vi "Actor Core.vi"(8 "error in":errorcluster, 11 "ZenGage v3.0 UI in":refnum<class "ZenGage v3.0 UI.lvclass">) -> (0 "error out":errorcluster, 3 "Actor out":refnum<class "Actor.lvclass">)   [LabVIEW 2019, in "ZenGage v3.0 UI.lvclass"]
uses:
  ZenGage v3.0 UI.lvclass
  <vilib>/ActorFramework/Actor/Actor.lvclass
  <vilib>/ActorFramework/Message Enqueuer/Message Priority.ctl
  <vilib>/ActorFramework/Message Enqueuer/Message Enqueuer.lvclass
  <vilib>/event_ctls.llb/usereventprio.ctl
  Type Definitions/Controls and Indicators/General_Control references.ctl
  Type Definitions/Controls and Indicators/Inspection control references.ctl
  Type Definitions/Controls and Indicators/Diagnostics control referencs.ctl
  Type Definitions/Controls and Indicators/EDL control references.ctl
  Type Definitions/Controls and Indicators/Controls and Indicators Cluster.ctl
  Common/Controls/Acknowledgement.ctl
  Type Definitions/Controls and Indicators/String2.ctl
  <vilib>/vision/Image Controls.llb/IMAQ Image.ctl
  Type Definitions/Diagnostics/OpticsPOSTInputCluster.ctl
  <vilib>/Utility/miscctls.llb/LVPoint32TypeDef.ctl
  User Interface Messages/User Interface messages/Call function_UI Msg/ButtonPress_UI.lvclass
  Common/Controls/Pop-up Input.ctl
  User Interface Messages/User Interface messages/Display Popup Msg/DisplayPopup_UI.lvclass
  Type Definitions/General/OutputDetails.ctl
  Type Definitions/General/Output choice.ctl
  Type Definitions/JSON Read/UI JSON read cluster.ctl
  Type Definitions/General/JSONRead.ctl
  Type Definitions/Inspection/Inspection Cluster.ctl
  Type Definitions/Diagnostics/Diagnostics(Cluster).ctl
  Type Definitions/Edit tolerance settings/Rack Selection.ctl
  Type Definitions/Edit tolerance settings/Edit Tolerance Input.ctl
  Type Definitions/Edit tolerance settings/Edit Tolerance Overall Cluster.ctl
  Type Definitions/General/UI States(UI button enable disable).ctl
  Type Definitions/General/UIDataCluster.ctl
  Type Definitions/General/Master sample references.ctl
  C:/Program Files/National Instruments/LabVIEW 2019/vi.lib/ActorFramework/Actor/Actor.lvclass
  User interface UX/LabVIEW components (Controls and Indiactors)/Tables and listboxes/Combo box conventional list.ctl
panel:
  out "Ignored count":u64
  in  "Main Tab":T1(tab)=enum."Blank"
  in  "Diagnostics Tab":T2(tab)
  out "TL":string
  out "SensorDiagnosticsImage":T3(plugin-control)
  out "BUZZER OFF":u32(colorbox)=14803425
  out "STOP":u32(colorbox)=14803425
  out "PAUSE":u32(colorbox)=14803425
  out "RUN":u32(colorbox)=14803425
  out "CAMERA STATUS\n       MESSAGE":string
  out "DUST INDICATOR":dbl format="%#.3f"
  out "Diagnostics Image_Diagnostics":T3(plugin-control)
  in  "Master sample tab":enum32{"Master sample", "Inspection"}(tab)
  out "Master sample message":string
  in  "Hide":bool
  out "Counts":T4 {"Production counts clustwer"."TOTAL" scale=0.0..100.0; "Production counts clustwer"."PASS" scale=0.0..100.0; "Production counts clustwer"."FAIL" scale=0.0..100.0; "Reel counts cluster"."TOTAL" scale=0.0..100.0; "Reel counts cluster"."PASS" scale=0.0..100.0; "Reel counts cluster"."FAIL" scale=0.0..100.0}
  in  "Image label 4":string(combo)
  in  "Image label 3":string(combo)
  in  "Image label 1":string(combo)
  out "Image 4":T3(plugin-control)
  out "Image 3":T3(plugin-control)
  in  "Image label 2":string(combo)
  out "Image 2":T3(plugin-control)
  out "Image 1":T3(plugin-control)
  in  "Tolerance Limits Listbox":i32(listbox)
  in  "Command Tab":T5(tab)=enum."Inspection"
  out "Production Fail Ignore Count":u64
  in  "Fail count reverse":bool
  in  "Select a part":T6="Select a part"
  in  "Door Poka \nYoke":bool
  in  "Factory reset":bool
  in  "Restore to defaults_Edit Tolerance":bool
  in  "Logout_EditTolerance":bool
  in  "Measurement\nEnable":bool
  in  "Update List":bool
  in  "Save":bool
  out "Reel Fail Ignore Count":u64
  in  "Select message":string
  in  "Settings_Inspection":bool
  in  "Analytics_Inspection":bool
  in  "Event reason switching tab":enum32{"EventReason", "InspectionButtons"}(tab)
  in  "Event  Reason  List":string(combo)
  out "Event reason blink":string="Select an event\n  reason below"
  in  "confirm_eventReason":bool
  in  "Run_Inspection":bool
  in  "Pause_Inspection":bool
  in  "Stop_Inspection":bool
  in  "confirm":bool
  in  "Total Count":u64
  in  "Reel Count":u64
  in  "Operator Name":string
  in  "Part Name":T6
  in  "reset":bool
  in  "ok":bool
  in  "change":bool
  out "VERIFIED":bool
  in  "Master sample part message":string
  in  "Repeat":bool
  in  "Next":bool
  in  "Select a sub diagnostics":T6="Select a part"
  in  "logout_Diagnostics":bool
  in  "Select a diagnostics":T6="Select a part"
  in  "JSONRead.ConfigurationCluster.UIParameters.ImageIndicatorLayouts":T7(array[cluster])=[{"NumberOfImageIndicators"=1.0, "ImageSpecificData"=[{"Width"=0.98, "Left"=0.0, "Top"=0.0, "ImagePercentage"={"Height"=0.95, "Widthcorrection"=-20, "Heightcorrection"=-44, "Leftcorrection"=0.0, "Topcorrection"=0.0}, "StringPercentage"={"Height"=0.05, "Widthcorrection"=-14, "Heightcorrection"=0.0, "Leftcorrection"=0.0, "Topcorrection"=5.0}}]}, {"NumberOfImageIndicators"=2.0, "ImageSpecificData"=[{"Width"=0.5, "Left"=0.0, "Top"=0.0, "ImagePercentage"={"Height"=0.95, "Widthcorrection"=-20, "Heightcorrection"=-47, "Leftcorrection"=0.0, "Topcorrection"=3.0}, "StringPercentage"={"Height"=0.05, "Widthcorrection"=-30, "Heightcorrection"=0.0, "Leftcorrection"=0.0, "Topcorrection"=7.0}}, {"Width"=0.5, "Left"=0.0, "Top"=0.0, "ImagePercentage"={"Height"=0.95, "Widthcorrection"=-20, "Heightcorrection"=-47, "Leftcorrection"=0.0, "Topcorrection"=3.0}, "StringPercentage"={"Height"=0.05, "Widthcorrection"=-30, "Heightcorrection"=0.0, "Leftcorrection"=0.0, "Topcorrection"=7.0}}]}, {"NumberOfImageIndicators"=3.0, "ImageSpecificData"=[{"Width"=0.5, "Left"=0.0, "Top"=0.0, "ImagePercentage"={"Height"=0.45, "Widthcorrection"=-30, "Heightcorrection"=-50, "Leftcorrection"=0.0, "Topcorrection"=5.0}, "StringPercentage"={"Height"=0.05, "Widthcorrection"=-30, "Heightcorrection"=0.0, "Leftcorrection"=0.0, "Topcorrection"=7.0}}, {"Width"=0.5, "Left"=0.0, "Top"=0.5, "ImagePercentage"={"Height"=0.45, "Widthcorrection"=-30, "Heightcorrection"=-50, "Leftcorrection"=0.0, "Topcorrection"=5.0}, "StringPercentage"={"Height"=0.05, "Widthcorrection"=-30, "Heightcorrection"=0.0, "Leftcorrection"=0.0, "Topcorrection"=5.0}}, {"Width"=0.5, "Left"=0.5, "Top"=0.0, "ImagePercentage"={"Height"=0.95, "Widthcorrection"=-30, "Heightcorrection"=-47, "Leftcorrection"=-3.0, "Topcorrection"=5.0}, "StringPercentage"={"Height"=0.05, "Widthcorrection"=-33, "Heightcorrection"=3.0, "Leftcorrection"=3.0, "Topcorrection"=5.0}}]}, {"NumberOfImageIndicators"=3.0, "ImageSpecificData"=[{"Width"=0.5, "Left"=0.0, "Top"=0.0, "ImagePercentage"={"Height"=0.45, "Widthcorrection"=-30, "Heightcorrection"=-50, "Leftcorrection"=0.0, "Topcorrection"=5.0}, "StringPercentage"={"Height"=0.05, "Widthcorrection"=-30, "Heightcorrection"=0.0, "Leftcorrection"=0.0, "Topcorrection"=7.0}}, {"Width"=0.5, "Left"=0.0, "Top"=0.5, "ImagePercentage"={"Height"=0.45, "Widthcorrection"=-30, "Heightcorrection"=-50, "Leftcorrection"=0.0, "Topcorrection"=5.0}, "StringPercentage"={"Height"=0.05, "Widthcorrection"=-30, "Heightcorrection"=0.0, "Leftcorrection"=0.0, "Topcorrection"=5.0}}, {"Width"=0.5, "Left"=0.5, "Top"=0.0, "ImagePercentage"={"Height"=0.95, "Widthcorrection"=-30, "Heightcorrection"=-47, "Leftcorrection"=-3.0, "Topcorrection"=5.0}, "StringPercentage"={"Height"=0.05, "Widthcorrection"=-33, "Heightcorrection"=3.0, "Leftcorrection"=3.0, "Topcorrection"=5.0}}, {"Width"=0.5, "Left"=0.5, "Top"=0.5, "ImagePercentage"={"Height"=0.45, "Widthcorrection"=-30, "Heightcorrection"=-50, "Leftcorrection"=0.0, "Topcorrection"=5.0}, "StringPercentage"={"Height"=0.05, "Widthcorrection"=-30, "Heightcorrection"=0.0, "Leftcorrection"=0.0, "Topcorrection"=5.0}}]}]
  in  "UpdateImagingViews":bool
  out "Program flow":string
  in  "Inspection Tab":T8(tab)=enum."Diagnostics"
  in  "Tab Control":enum32{"EventReason"}(tab)
  out "Cards array":T9(array[cluster]) {"Measurement value" format="%#.3g"}
  out "Pass-Fail Indicator String":string
  out "Status display":u32(colorbox)=14277081
  in  "Diagnostics Status\nString":string
  out "Current\nDiagnostics\nStatus":u32(colorbox)=11776947
  in  "ETS tab":enum32{"Display", "Blank"}(tab)=enum."Blank"
  in  "Cluster of limits":T10
  in  "Threshold limits":T11 {"Spec Limit Fail Window" max=100000; "Control Limit Fail Window" max=100; "Spec Limit Fail Allowable" max=100000; "Control Limit Fail Allowable" max=100}
  in  "Bias Correction":dbl
  in  "Linearity Correction":dbl
  in  "ETL count error message":string
  out "ETL help string":string
  in  "SoftwareExit":bool caption="SoftwareExit_Inspection"
  # "Please select a measurement checkbox to make the required changes for that particular measurement"
  # "%"
  # "PRODUCTION"
  # "REEL"
  # "MASTER SAMPLE       VALIDATION"
  # "mm"
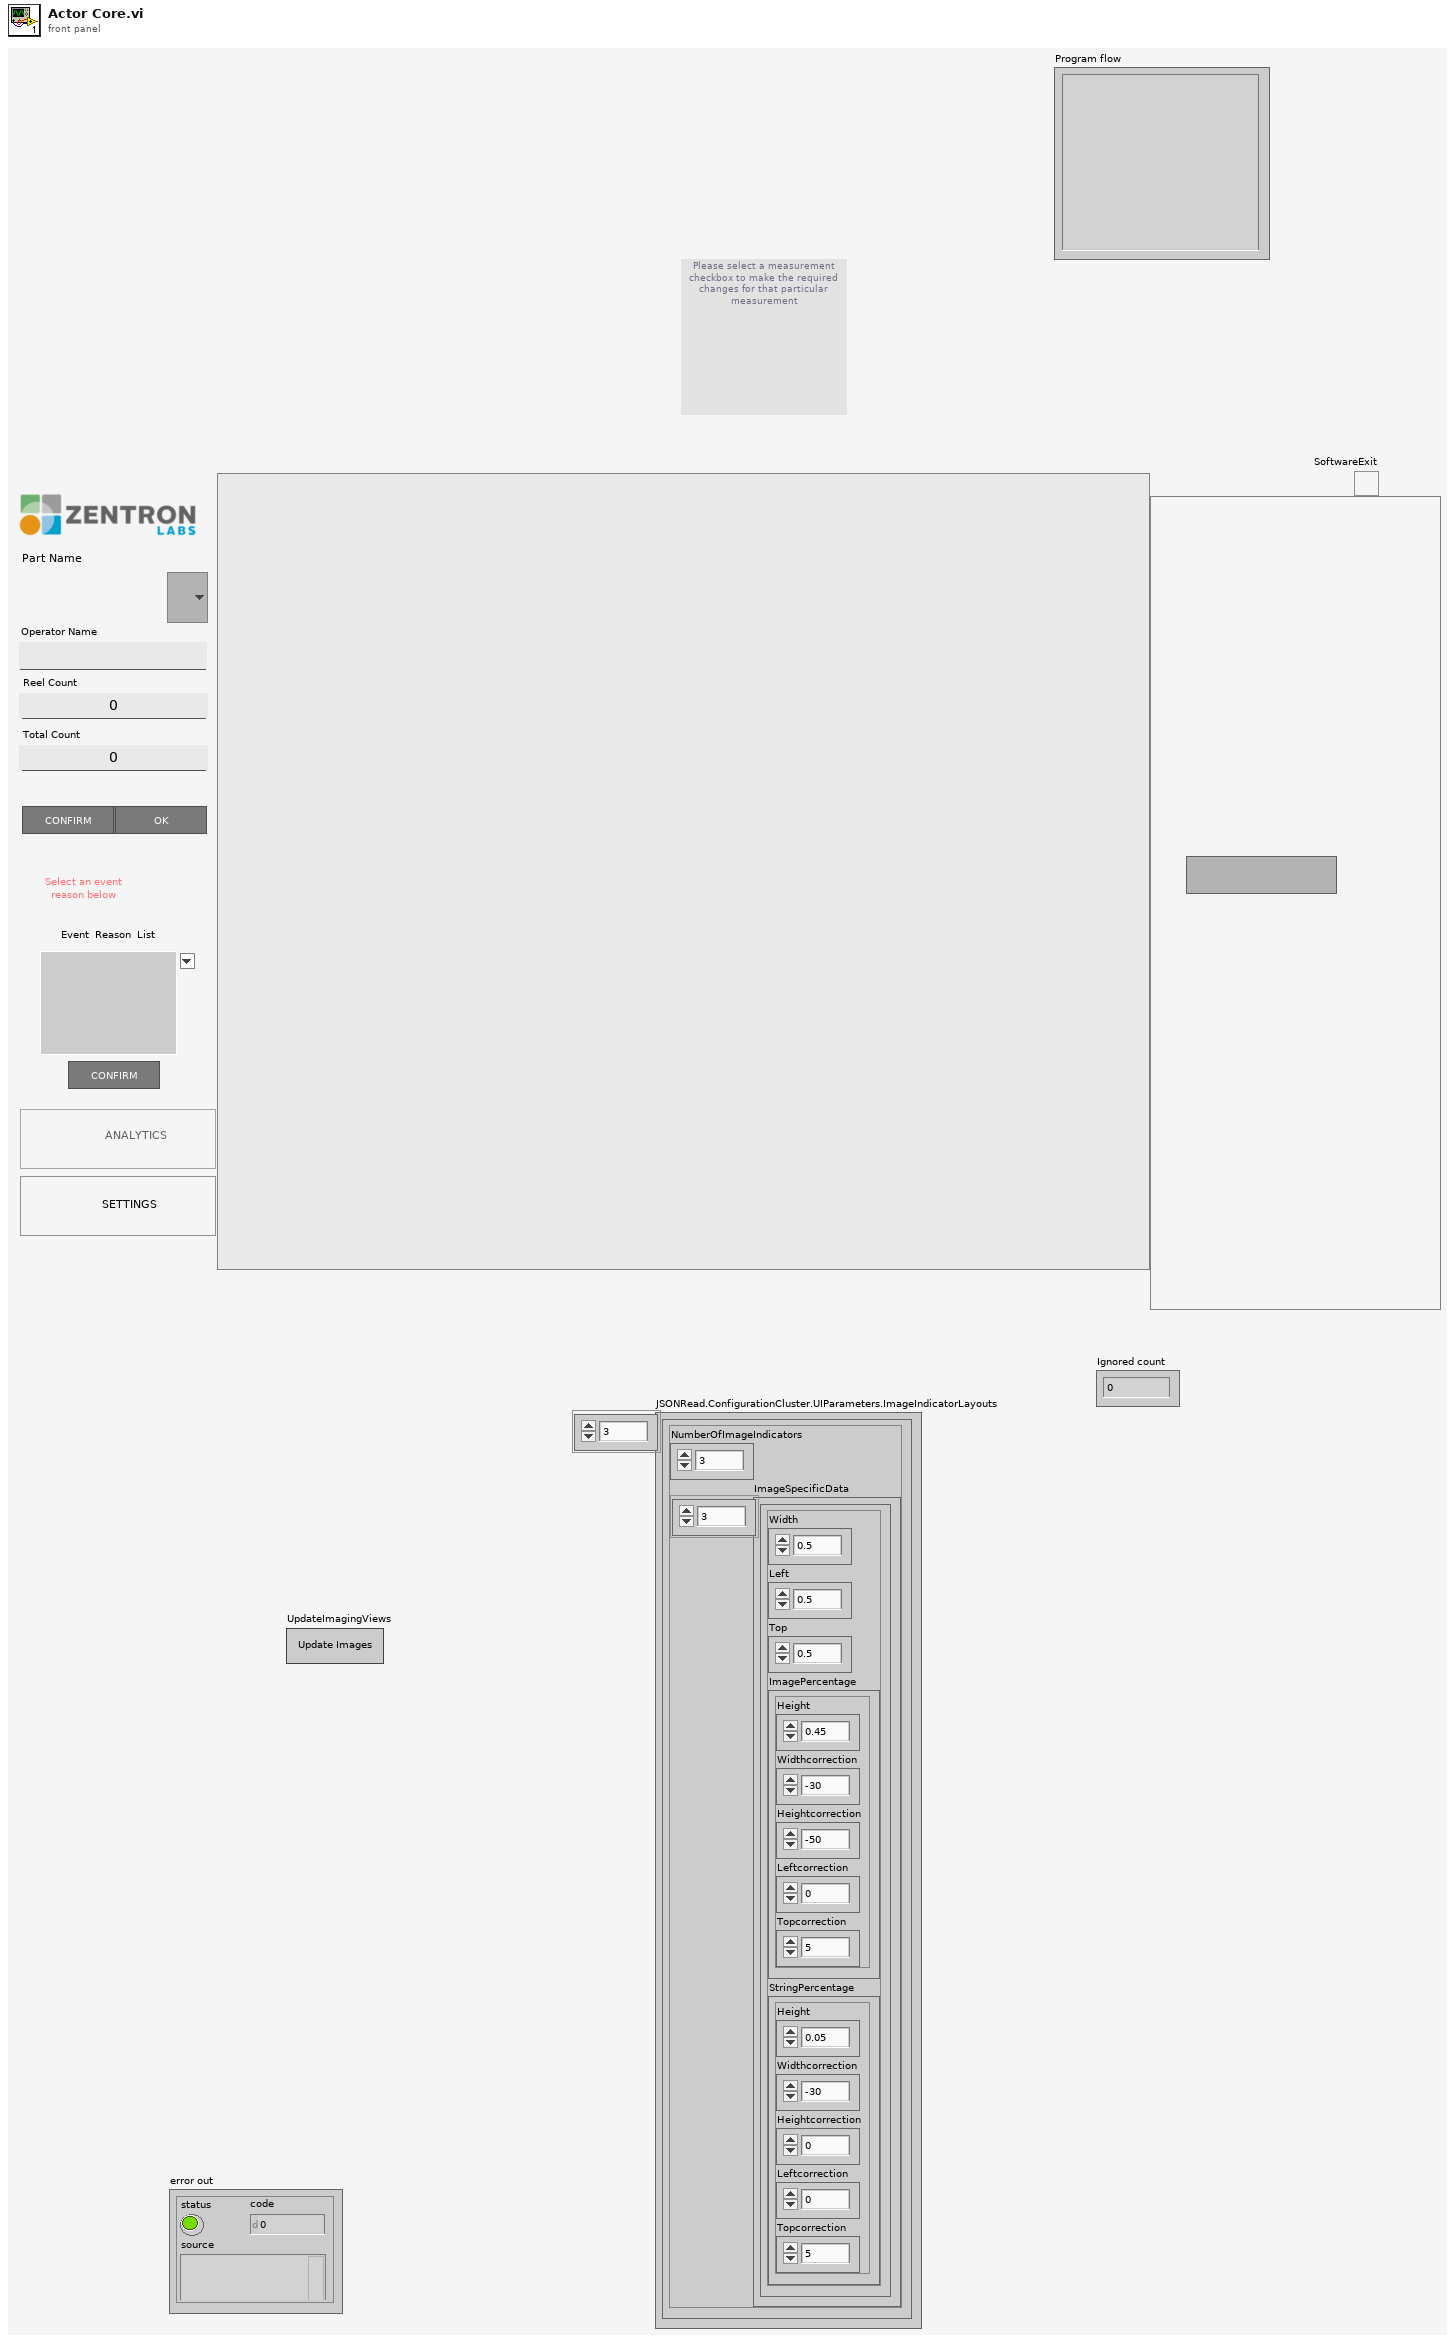
[diagram p1: front panel]
types:
  T1 = enum32{"Analytics", "Blank", "Diagnostics", "Run", "Edit Tolerance Settings"}
  T2 = enum32{"Arduino Motor", "Sensor trigger", "Hardware Button", "Camera Optics"}
  T3 = typedef "IMAQ Image.ctl" = refnum<image>
  T4 = cluster{"Reel counts cluster":cluster{"PASS":u64, "FAIL":u64, "TOTAL":u64}, "Production counts clustwer":cluster{"PASS":u64, "FAIL":u64, "TOTAL":u64}}
  T5 = enum32{"Edit Tolerance Limits1", "Inspection", "Master sample", "Diagnostics"}
  T6 = typedef "ZenGage v3.0 UI.lvclass/Combo box conventional list.ctl" = string
  T7 = cluster{"NumberOfImageIndicators":dbl, "ImageSpecificData":cluster{"Width":dbl, "Left":dbl, "Top":dbl, "ImagePercentage":cluster{"Height":dbl, "Widthcorrection":i64, "Heightcorrection":i64, "Leftcorrection":dbl, "Topcorrection":dbl}, "StringPercentage":cluster{"Height":dbl, "Widthcorrection":i64, "Heightcorrection":dbl, "Leftcorrection":dbl, "Topcorrection":dbl}}[]}[]
  T8 = enum32{"Inspection", "Diagnostics", "Edit Tolerance Settings"}
  T9 = cluster{"Measruement Name":string, "Measruement pass?":bool, "LSL":string, "USL 2":string, "Measurement value":dbl}[]
  T10 = cluster{"LSL":dbl, "USL":dbl, "LCL":dbl, "UCL":dbl}
  T11 = cluster{"Control Limit Fail Allowable":u64, "Spec Limit Fail Allowable":u64, "Control Limit Fail Window":u64, "Spec Limit Fail Window":u64}
  T12 = typedef "ZenGage v3.0 UI.lvclass/Controls and Indicators Cluster.ctl" = cluster{"General":T13, "Inspection":T14, "Diagnostics":T15, "Edit Tolerance Limits":T16, "Master sample":T17}
  T13 = typedef "ZenGage v3.0 UI.lvclass/General_Control references.ctl" = cluster{"Main Tab":refnum<vi>, "Inspection SubPanel_Inspection":refnum<vi>, "Zen Logo_Inspection":refnum<vi>, "SoftwareExit":refnum<vi>, "Loading Bar VI Ref":refnum<vi>, "Right Pane Tab":refnum<vi>, "Image Reference array":refnum<vi>[], "Command tab":refnum<vi>, "Inspection subTab control ref":refnum<vi>, "SelectionCluster":cluster{"ok":refnum<vi>, "confirm":refnum<vi>, "reset":refnum<vi>, "change":refnum<vi>, "TOTAL COUNT":refnum<vi>, "REEL COUNT":refnum<vi>, "PART NAME":refnum<vi>, "VERIFIED":refnum<vi>, "OPERATOR NAME":refnum<vi>, "Select message":refnum<vi>}, "Event  Reason  List":refnum<vi>, "Event reason blink":refnum<vi>, "Event reason switching tab":refnum<vi>, "confirm_eventReason":refnum<vi>}
  T14 = typedef "ZenGage v3.0 UI.lvclass/Inspection control references.ctl" = cluster{"Inspection Status":refnum<vi>, "Run_Inspection":refnum<vi>, "Pause_Inspection":refnum<vi>, "Stop_Inspection":refnum<vi>, "Settings_Inspection":refnum<vi>, "Inspection Images VI Ref":refnum<vi>, "Pass-Fail Indicator String":refnum<vi>, "Analytics_Inspection":refnum<vi>, "Label array":refnum<vi>[], "Analytics VI\nreference":refnum<vi>, "Counts":refnum<vi>, "Cards array":refnum<vi>, "Counts array":refnum<vi>[]}
  T15 = typedef "ZenGage v3.0 UI.lvclass/Diagnostics control referencs.ctl" = cluster{"Diagnostics Tab":refnum<vi>, "Dust indicator :":refnum<vi>, "Logout_Diagnostics":refnum<vi>, "CAMERA STATUS MESSAGE":refnum<vi>, "BUZZER OFF":refnum<vi>, "PAUSE":refnum<vi>, "STOP":refnum<vi>, "RUN":refnum<vi>, "Current Diagnostics Status":refnum<vi>, "Select a diagnostics":refnum<vi>, "Diagnostics Status":refnum<vi>, "Select a sub diagnostics":refnum<vi>, "Optics img":refnum<vi>, "Diagnostics Status\nString":refnum<vi>}
  T16 = typedef "ZenGage v3.0 UI.lvclass/EDL control references.ctl" = cluster{"Tolerance Limits Listbox":refnum<vi>, "Enable Disable":refnum<vi>, "Cluster of limits":refnum<vi>, "Thresholds limits":refnum<vi>, "Update List":refnum<vi>, "Save":refnum<vi>, "Back_Edit Tolerance":refnum<vi>, "logout":refnum<vi>, "Select a part":refnum<vi>, "Bias Correction":refnum<vi>, "Linearity Correction":refnum<vi>, "Select a Rack":refnum<vi>, "ETS tab":refnum<vi>, "Factory reset":refnum<vi>, "Door\nPoka Yoke":refnum<vi>, "Fail count reverse":refnum<vi>, "ETL count error message":refnum<vi>, "ETL help string":refnum<vi>}
  T17 = typedef "Master sample references.ctl" = cluster{"Master sample message":refnum<vi>, "Master sample tab":refnum<vi>, "Next":refnum<vi>, "Repeat":refnum<vi>, "Master sample part message":refnum<vi>}
  T18 = cluster{"ok":refnum<vi>, "confirm":refnum<vi>, "reset":refnum<vi>, "change":refnum<vi>, "TOTAL COUNT":refnum<vi>, "REEL COUNT":refnum<vi>, "PART NAME":refnum<vi>, "VERIFIED":refnum<vi>, "OPERATOR NAME":refnum<vi>, "Select message":refnum<vi>}
  T19 = typedef "ZenGage v3.0 UI.lvclass/OpticsPOSTInputCluster.ctl" = cluster{"Dust Percentage":dbl, "Diagnostics Sstatus string":string, "Pass?":bool, "final image":T3}
  T20 = typedef "ZenGage v3.0 UI.lvclass/String2.ctl" = string
  T21 = cluster{"MNA":string[], "ISIM":u8[], "Image update":cluster{"Rack Id":i32, "Update image":bool[]}[], "Current rack Id":u8, "LSL":string[], "USL":string[]}
  T22 = cluster{"Camera names":string[], "Rack Id 2":u8, "Measurement names":string[], "Number of racks":u8, "Tolerance limits":string[]}
  T23 = enum32{"invalid app kind", "Development System", "Run Time System", "Student Edition", "Embedded LabVIEW", "Evaluation", "Custom"}
  T24 = typedef "ZenGage v3.0 UI.lvclass/Output choice.ctl" = enum16{"SendIgnoredFailCount", "SendPartDetails", "ButtonPress", "SendAcknowledgement", "InitiateCameraDiagnostics", "InitiateSensorDiagnostics", "SendPopupResponse", "SendEventReasonResponse", "SendErrorDetails"}
  T25 = typedef "ZenGage v3.0 UI.lvclass/OutputDetails.ctl" = cluster{"Acknowledgement_SM":T26, "Button name":string, "PartDetails":cluster{"PartName":string, "ConnectorsInReel":u64, "TotalCounts":u64, "OperatorName":string, "StampingMachineID":u32}, "SensorName":string, "CameraName":string, "PopupFeedbackDetails":cluster{"Pop-up Type":enum16{"Open Logo Display", "Close Logo Display", "Open Loading Bar", "Close Loading Bar", "Open Alert Display", "Close Alert Display", "One button dialog box", "Two button dialog box", "User Authentication"}, "Message":string, "Pressed Button":string}, "EventResponse":string, "ErrorMessage":string, "FailCountIgnore":cluster{"ReelIgnoreCount":u64, "ProductionIgnoreCount":u64}}
  T26 = typedef "Acknowledgement.ctl" = cluster{"Enqueuer":refnum<class "Message Enqueuer.lvclass">, "VIReference":refnum<vi>, "VIName":string}
  T27 = enum32{"Invalid", "Standard", "Closed", "Hidden", "Minimized", "Maximized"}
  T28 = enum8{"Enabled", "Disabled", "Disabled and Grayed Out"}
  T29 = typedef "usereventprio.ctl" = enum32{"high priority", "normal priority"}
  T30 = cluster{"Image refnum":refnum<vi>, "Label refnum":refnum<vi>}
  T31 = cluster{"Part Name":refnum<vi>, "Verification":refnum<vi>, "Change":refnum<vi>, "Confirm":refnum<vi>, "OK Button":refnum<vi>, "Reset Button":refnum<vi>, "Total count":refnum<vi>, "Reel count":refnum<vi>, "Operator ID":refnum<vi>, "Select message":refnum<vi>, "Inspection Run":refnum<vi>}
  T32 = cluster{"Selection cluster":cluster{"ok":refnum<vi>, "confirm":refnum<vi>, "reset":refnum<vi>, "change":refnum<vi>, "TOTAL COUNT":refnum<vi>, "REEL COUNT":refnum<vi>, "PART NAME":refnum<vi>, "VERIFIED":refnum<vi>, "OPERATOR NAME":refnum<vi>, "Select message":refnum<vi>}, "Event  Reason  List":refnum<vi>}
  T33 = cluster{"Label array":refnum<vi>[], "Image ref array":refnum<vi>[], "Rack 1 Tbl Refnum":refnum<vi>, "Tab control":refnum<vi>, "Rack 2 Tbl Refnum":refnum<vi>, "String label":refnum<vi>[], "Diagnostics tab ref":refnum<vi>, "Counts":refnum<vi>}
  T34 = typedef "Actor Framework.lvlib/Message Enqueuer.lvclass/Message Priority.ctl" = enum16{"Low", "Normal", "High"}
  T35 = enum16{"Open Logo Display", "Close Logo Display", "Open Loading Bar", "Close Loading Bar", "Open Alert Display", "Close Alert Display", "One button dialog box", "Two button dialog box", "User Authentication"}
  T36 = cluster{"Stop slave user event_UI":refnum<user-event>, "Enable shortkey":refnum<user-event>, "SendClusterData":refnum<user-event>, "SendClusterData to MainLoop":refnum<user-event>}
  T37 = typedef "ZenGage v3.0 UI.lvclass/UserEvents_UI.ctl" = cluster{"LoadingBar_General_UI":refnum<user-event>, "OpticsDiagnostics_UI":refnum<user-event>, "DisplayResult_UI":refnum<user-event>, "DisplayPopup_UI":refnum<user-event>, "DisplayProcessCapabilityPopup_UI":refnum<user-event>, "ButtonPress_UI":refnum<user-event>, "GetAnalyticsVI_UI":refnum<user-event>, "SystemInfo_UI":refnum<user-event>, "PartInfo_UI":refnum<user-event>, "TriggerSensorDiagnostics_UI":refnum<user-event>, "AskEventReason_UI":refnum<user-event>, "Display CpCpk data_UI":refnum<user-event>, "MasterSampleMessageUpdate_UI":refnum<user-event>}
  T38 = typedef "UIDataCluster.ctl" = cluster{"JSONRead":T39, "Inspection":T41, "Diagnostics":T42, "EditToleranceSettings":T43, "ControlsIndicators":T12, "AdditionalFeatures":cluster{"Cp Cpk details":cluster{"CpCpkData":string[][], "Cp Cpk popup":refnum<vi>}, "Popup":cluster{"Restore main tab":string, "Popup data":cluster{"Loading bar data":cluster{"Open?":bool, "Display string":string}, "Pop-up":T47}}, "DynamicImageHandling":cluster{"Image update":cluster{"Rack Id":i32, "Update image":bool[]}[], "RBCIA":cluster{"Rack Id":u8, "Imaging view names":string[]}[], "ISIM":u8[], "Camera labels list":string[], "Enable DIH?":bool, "Init DIH params?":bool}, "PageHandling":cluster{"Previous State":T48, "Current state":string, "Previous control access state":string}, "Core":cluster{"Current VI Reference":refnum<vi>, "Close Panel on Exit?":bool}, "SlaveLoopData":cluster{"EnableShortKeyPress":bool, "Point32":T46}, "Chosen event reason":string, "Master sample validation":cluster{"Master sample general message":string, "Master sample part message":string}, "Fail Ignore Count Reversal":cluster{"Production ignored count":u64, "Reel ignored count":u64}}}
  T39 = typedef "ZenGage v3.0 UI.lvclass/JSONRead.ctl" = cluster{"ConfigurationFilePaths":cluster{"Default JSON Path in":path, "Rack Controller Override JSON file path in":path, "Algorithm Overrride JSON file path in ":path}, "ConfigurationVariants":cluster{"Default JSON \nVariant":variant, "Algorithm Override\nJSON Variant":variant, "Rack Controller Override\nJSON Variant":variant}, "ConfigurationCluster":T40}
  T40 = typedef "ZenGage v3.0 UI.lvclass/UI JSON read cluster.ctl" = cluster{"UIParameters":cluster{"SpecificationVersion":string, "Title":string, "NumberOfImagesToBeDisplayed":dbl, "ImageCountWindow":dbl, "FontName":string, "FontSize":dbl, "CustomerLogoFilePath":string, "ZentronLogoFilePath":string, "CompatibleSoftwareVersions":string[], "CameraLabelMapping":cluster{"CameraName":string, "ImageLabel":string}[], "ImageIndicatorLayouts":cluster{"NumberOfImageIndicators":dbl, "ImageSpecificData":cluster{"Width":dbl, "Left":dbl, "Top":dbl, "ImagePercentage":cluster{"Height":dbl, "Widthcorrection":i64, "Heightcorrection":i64, "Leftcorrection":dbl, "Topcorrection":dbl}, "StringPercentage":cluster{"Height":dbl, "Widthcorrection":i64, "Heightcorrection":dbl, "Leftcorrection":dbl, "Topcorrection":dbl}}[]}[], "SoftwareButtonLabels":cluster{"SelectLabel":string, "RunLabel":string, "PauseLabel":string, "StopLabel":string}, "DiagnosticsParameters":cluster{"CameraOpticsDiagnostics":cluster{"Label":string, "CameraLabelsList":cluster{"CameraName":string, "ImageLabel":string}[]}, "ArduinoDiagnostics":cluster{"Label":string}, "MotorDiagnostics":cluster{"Label":string}, "ReelerMotor":cluster{"Label":string}, "TowerLampDiagnostics":cluster{"Label":string}, "TriggerSensor":cluster{"Label":string, "SensorsList":cluster{"SensorName":string, "LabelName":string}[]}, "HardwareButtonDiagnostics":cluster{"Label":string}, "MasterSampleDiagnostics":cluster{"Label":string}}, "DieIdParameters":cluster{"DefaultDieId":string, "DieIdsList":string[]}, "EventReasonsList":cluster{"Pause":string[], "Stop":string[], "FailPause":string[], "Ignored":string[], "DefaultEventReason":string}, "StampingMachineIds":string[], "ErrorPopupStrings":cluster{"ErrorCode":string, "ErrorString":string}[]}}
  T41 = typedef "ZenGage v3.0 UI.lvclass/Inspection Cluster.ctl" = cluster{"Inspection After Stop":bool, "IsPaused":bool, "Camera Names":string[], "Fail Array":bool[], "Reel Number":u32, "Image details_init":cluster{"Mapped view names":string[], "Camera image map array":i32[], "Camera names":string[]}[], "LSL":string[], "USL":string[], "Max limits":cluster{"Production max":u64, "Reel max":u64}, "parts List":string[], "#Racks":u8, "MeasurementNames":string[], "Reel complete":bool, "Fail event reason list":string[]}
  T42 = typedef "ZenGage v3.0 UI.lvclass/Diagnostics(Cluster).ctl" = cluster{"Selection Done?":bool, "Diagnostics details":cluster{"Diagnostics names":cluster{"Main diagnostics":string[], "Sub diagnostics names":cluster{"Camera optics":string[], "Trigger sensor":string[]}}, "Diagnostics labels":cluster{"Main diagnostics":string[], "Sub diagnostics names":cluster{"Camera optics":string[], "Trigger sensor":string[]}}}, "DiagnosticsFeatures":cluster{"ArduinoDiagnostics":bool, "MotorDiagnostics":bool, "CameraOpticsDiagnostics":bool, "ReelerMotor":bool, "HardwareButtonDiagnostics":bool, "TriggerSensor":bool, "TowerLampDiagnostics":bool, "MasterSampleDiagnostics":bool}, "SelectedDiagnostics":string}
  T43 = typedef "ZenGage v3.0 UI.lvclass/Edit Tolerance Overall Cluster.ctl" = cluster{"Input ListBox":T44, "Saved?":bool, "IsETLSelected":bool, "IsPartSelected":bool}
  T44 = typedef "ZenGage v3.0 UI.lvclass/Edit Tolerance Input.ctl" = cluster{"Measurement Values":string[][], "Cluster of Limits":cluster{"LSL":dbl, "USL":dbl, "LCL":dbl, "UCL":dbl}, "Rack Selection":T45, "M and N Array":cluster{"M1":u64, "M2":u64, "N1":u64, "N2":u64}[], "Ticked Measurement Index":u32[], "Measurements Enabled":bool[], "Current Active Position":T46, "Current ticked measurement":dbl}
  T45 = typedef "ZenGage v3.0 UI.lvclass/Rack Selection.ctl" = enum16{"Both Racks", "Rack 2", "Rack 1"}
  T46 = typedef "LVPoint32TypeDef.ctl" = cluster{"Horizontal":i32, "Vertical":i32}
  T47 = typedef "Pop-up Input.ctl" = cluster{"Pop-up Type":enum16{"Open Logo Display", "Close Logo Display", "Open Loading Bar", "Close Loading Bar", "Open Alert Display", "Close Alert Display", "One button dialog box", "Two button dialog box", "User Authentication"}, "Title":string, "Message":string, "Button 1 Text":string, "Button 2 Text":string, "Show Close? T/F":bool, "Title Blink? T/F":bool, "Title Blink Colour":u32}
  T48 = typedef "ZenGage v3.0 UI.lvclass/UI States(UI button enable disable).ctl" = cluster{"Inspection":cluster{"Inspection States":enum16{"PreSelect", "Back _Inspection", "Analytics", "Ready To Run", "Ready To Insert", "Enable All buttons", "Disable All Buttons", "Settings", "Select", "Stop", "Pause", "Inspect"}}, "Diagnostics":cluster{"Diagnostics States":enum16{"Enable All", "Camera Optics Fail", "Loading Bar", "Camera Optics", "Motor", "Arduino", "POST Done", "POST"}}, "Edit Tolerance":cluster{"Edit Limits":enum16{"Update List"}, "Enable Disable Measurements":enum16{"Back to Edit Tolerance"}, "Page Select":enum16{"Edit Tolerance Limits", "Enable Disable Buttons"}}, "Page Select":enum16{"Edit Tolerance", "Diagnostics", "Inspection"}}
  T49 = cluster{"Total Count":dbl, "Total Pass":dbl, "Total Fail":dbl}
  T50 = typedef "ZenGage v3.0 UI.lvclass/Result Cluster.ctl" = cluster{"Rack Id":u64, "Measurement Values Array ":dbl[], "Images_Array_in":T3[], "ResultPF":bool, "Production count details":cluster{"Total Count":dbl, "Total Pass":dbl, "Total Fail":dbl}, "Control Pass Fail":bool[], "ReelCount Details":cluster{"Reel Count":dbl, "Reel Pass":dbl, "Reel Fail":dbl}, "Specification Pass Fail":bool[], "SpecificationFail":bool}
  T51 = cluster{"Top Left":T3, "Bottom Left":T3, "Top Right":T3, "Inspection Status 2":u32, "Pass-Fail Indicator String 2":string, "Bottom right":T3, "Valid image data?":bool[], "Valid table data?":bool[], "Cards":cluster{"Measurement Name":string, "Pass?":bool, "LSL":string, "USL":string, "Measruement Value":dbl}[], "Counts":cluster{"Reel":cluster{"Pass":u64, "Fail":u64, "Total":u64}, "Production":cluster{"Pass":u64, "Fail":u64, "Total":u64}}}
  T52 = cluster{"Reel":cluster{"Pass":u64, "Fail":u64, "Total":u64}, "Production":cluster{"Pass":u64, "Fail":u64, "Total":u64}}
  T53 = cluster{"Measurement Name":string, "Pass?":bool, "LSL":string, "USL":string, "Measruement Value":dbl}[]
  T54 = cluster{"ArduinoDiagnostics":bool, "MotorDiagnostics":bool, "CameraOpticsDiagnostics":bool, "ReelerMotor":bool, "TowerLampDiagnostics":bool, "HardwareButtonDiagnostics":bool, "TriggerSensor":bool, "MasterSampleDiagnostics":bool}
  T55 = cluster{"Part name":string, "NumberOfRacks":u8}[]
  T56 = cluster{"LCL":dbl, "UCL":dbl, "LSL":dbl, "USL":dbl, "NominalValue":dbl}[]
  T57 = cluster{"Mapped view names":string[], "Camera image map array":i32[], "Camera names":string[]}[]
  T58 = cluster{"Cp Cpk details":cluster{"CpCpkData":string[][], "Cp Cpk popup":refnum<vi>}, "Popup":cluster{"Restore main tab":string, "Popup data":cluster{"Loading bar data":cluster{"Open?":bool, "Display string":string}, "Pop-up":T47}}, "DynamicImageHandling":cluster{"Image update":cluster{"Rack Id":i32, "Update image":bool[]}[], "RBCIA":cluster{"Rack Id":u8, "Imaging view names":string[]}[], "ISIM":u8[], "Camera labels list":string[], "Enable DIH?":bool, "Init DIH params?":bool}, "PageHandling":cluster{"Previous State":T48, "Current state":string, "Previous control access state":string}, "Core":cluster{"Current VI Reference":refnum<vi>, "Close Panel on Exit?":bool}, "SlaveLoopData":cluster{"EnableShortKeyPress":bool, "Point32":T46}, "Chosen event reason":string, "Master sample validation":cluster{"Master sample general message":string, "Master sample part message":string}, "Fail Ignore Count Reversal":cluster{"Production ignored count":u64, "Reel ignored count":u64}}
  T59 = cluster{"Image update":cluster{"Rack Id":i32, "Update image":bool[]}[], "RBCIA":cluster{"Rack Id":u8, "Imaging view names":string[]}[], "ISIM":u8[], "Camera labels list":string[], "Enable DIH?":bool, "Init DIH params?":bool}
  T60 = cluster{"Image update":cluster{"Rack Id":i32, "Update image":bool[]}[], "RBCIA":cluster{"Rack Id":u8, "Imaging view names":string[]}[], "ISIM":u8[], "Camera labels list":string[], "Enable DIH?":bool, "Init params":bool}
  T61 = cluster{"Default JSON Path in":path, "Rack Controller Override JSON file path in":path, "Algorithm Overrride JSON file path in ":path}
  T62 = cluster{"Current VI Reference":refnum<vi>, "Close Panel on Exit?":bool}
  T63 = typedef "ZenGage v3.0 UI.lvclass/Pop-up Output.ctl" = cluster{"Pop-up Type":enum16{"Open Logo Display", "Close Logo Display", "Open Loading Bar", "Close Loading Bar", "Open Alert Display", "Close Alert Display", "One button dialog box", "Two button dialog box", "User Authentication"}, "Message":string, "Pressed Button":string}
  T64 = cluster{"PartName":string, "ConnectorsInReel":u64, "TotalCounts":u64, "OperatorName":string, "StampingMachineID":u32}
  T65 = cluster{"CameraName":string, "ImageLabel":string}[]
  T66 = enum16{"cancel", "edit tolerance", "diagnostics"}
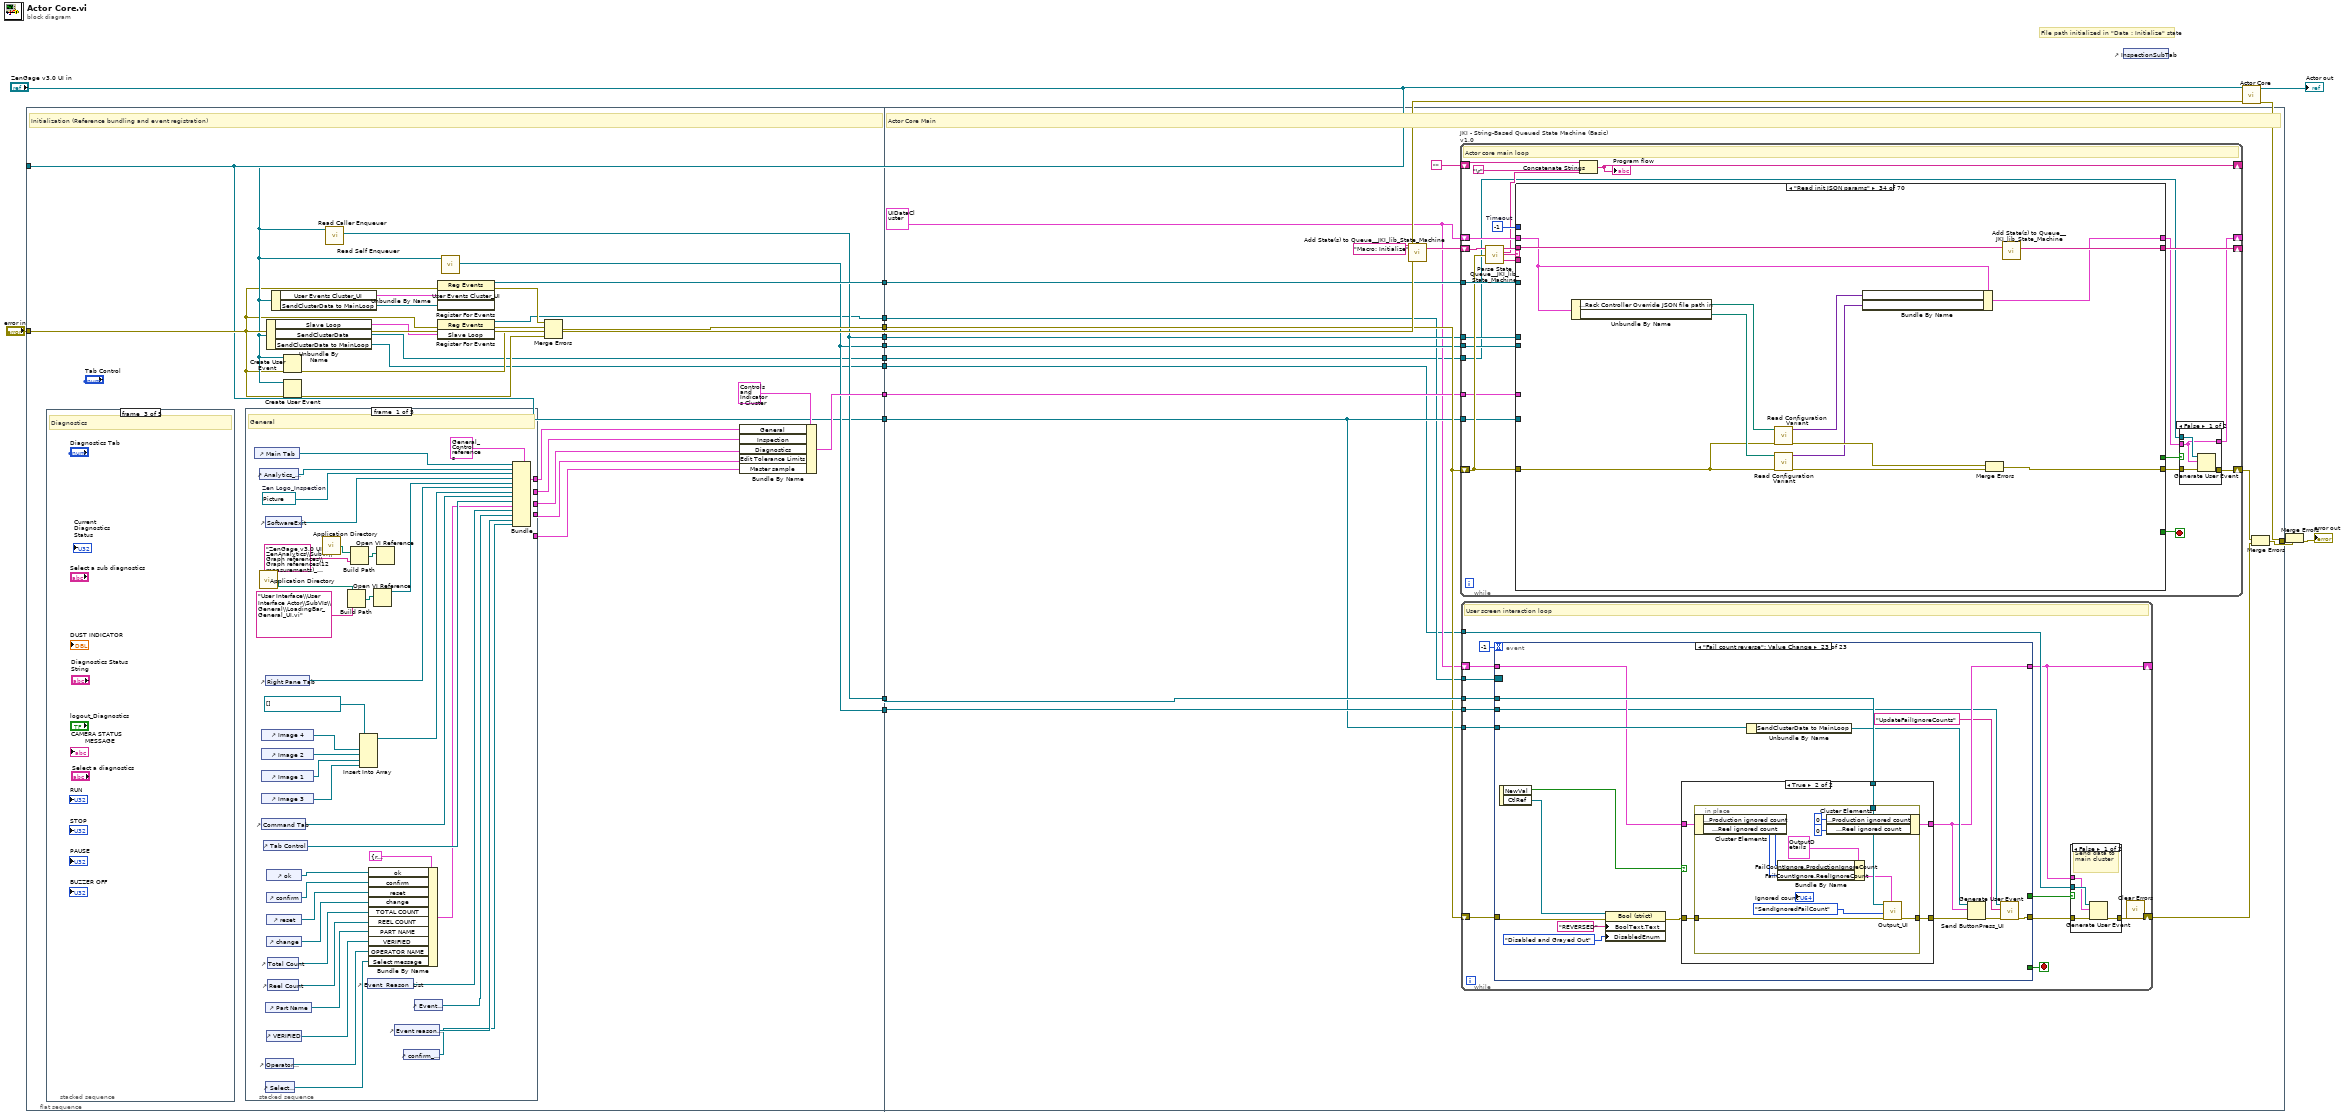
[diagram p0: block diagram]
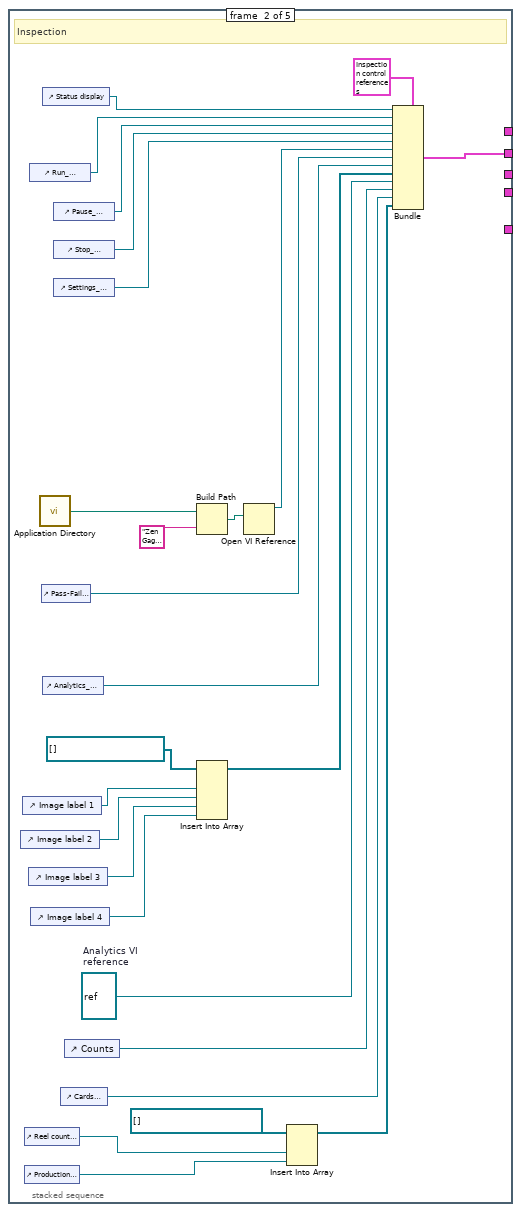
[diagram p2: hidden frame]
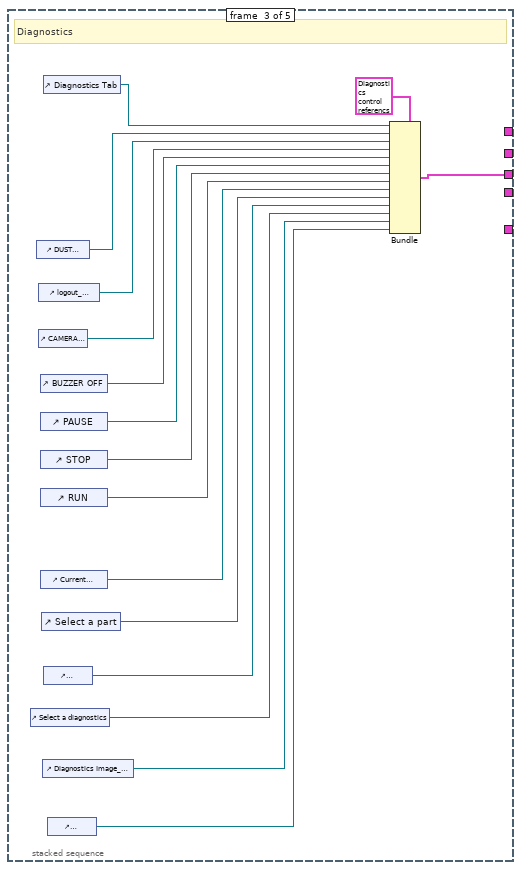
[diagram p3: hidden frame]
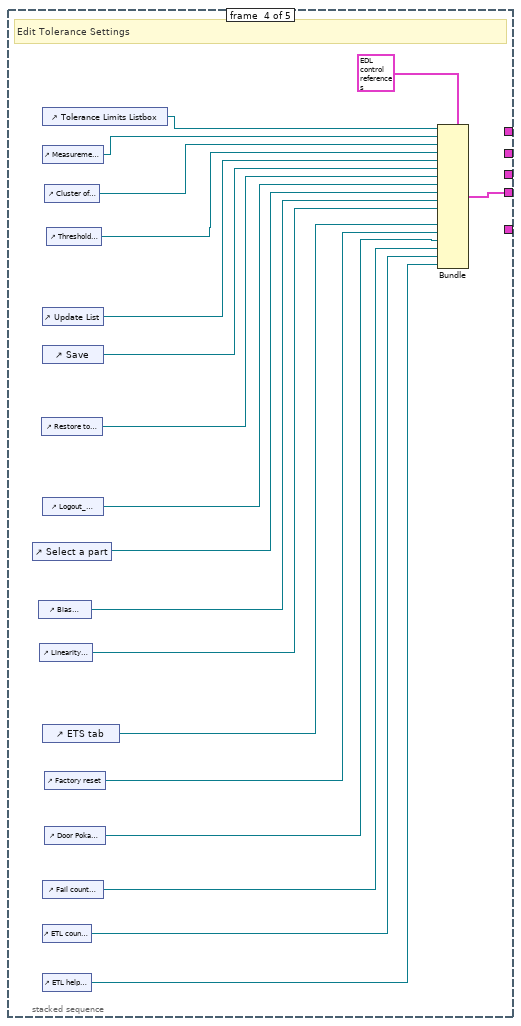
[diagram p4: hidden frame]
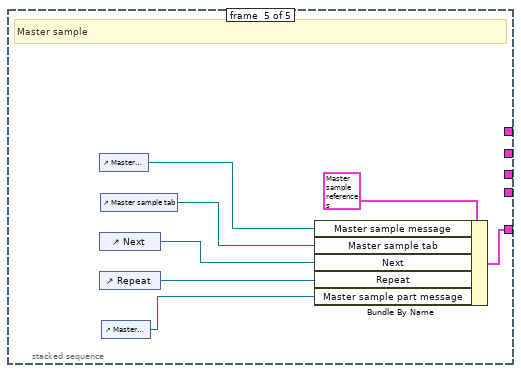
[diagram p5: hidden frame]
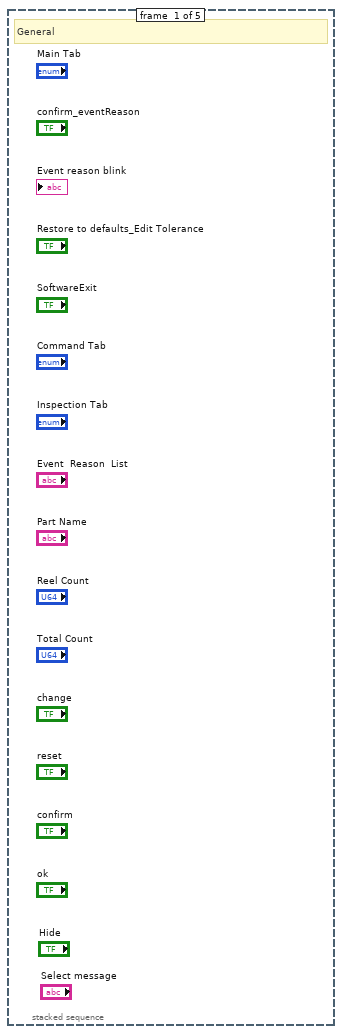
[diagram p6: hidden frame]
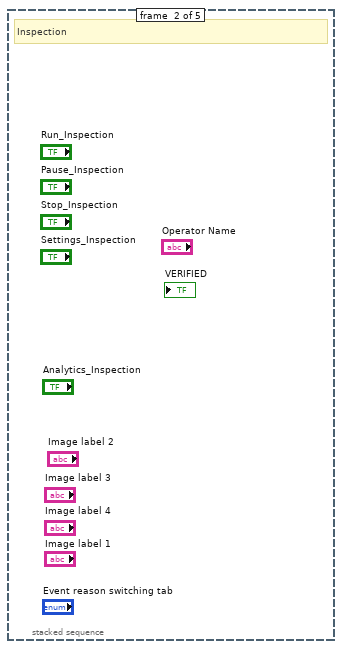
[diagram p7: hidden frame]
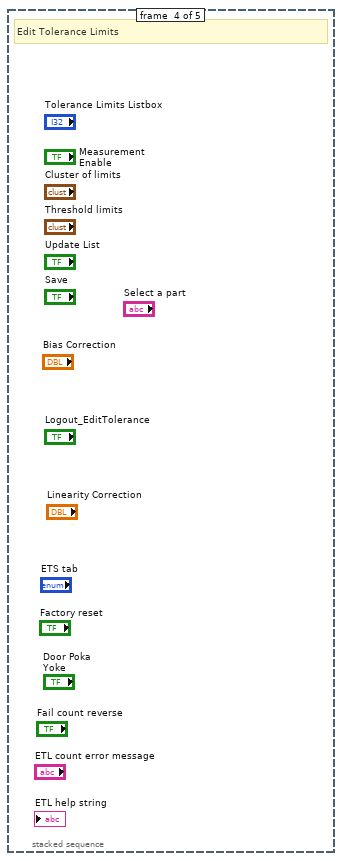
[diagram p8: hidden frame]
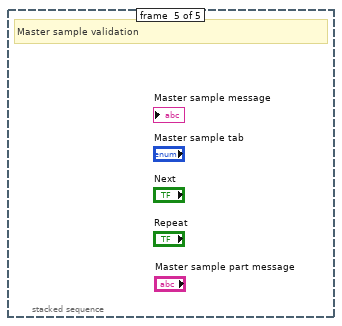
[diagram p9: hidden frame]
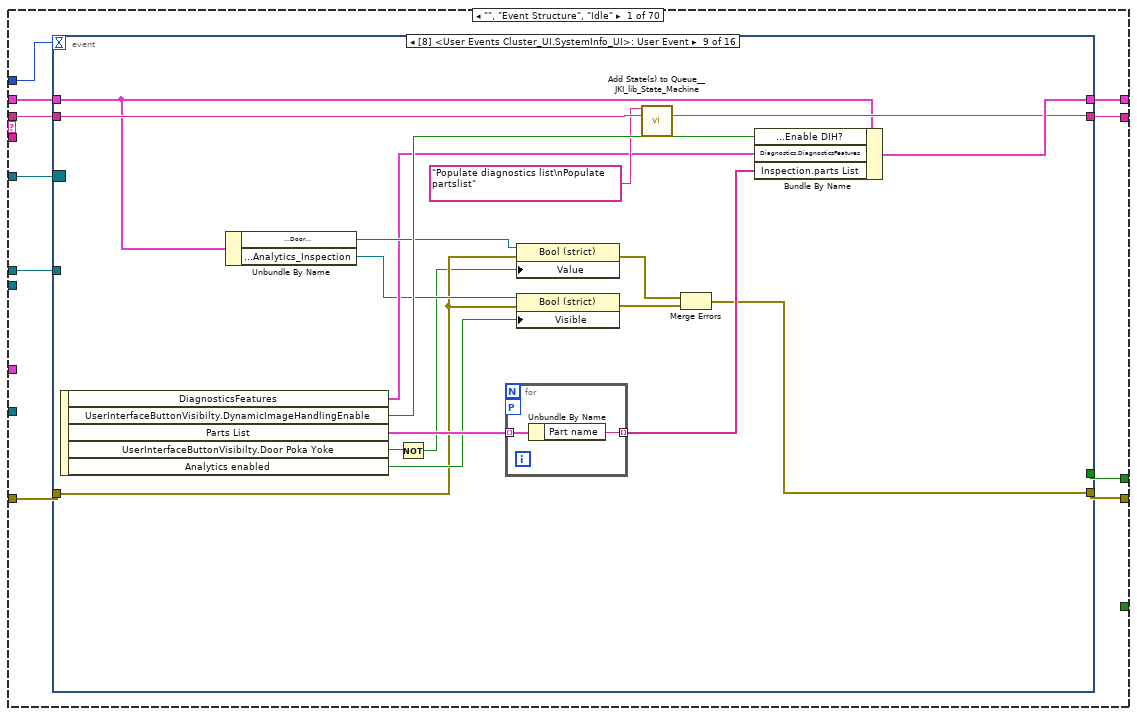
[diagram p11: hidden frame]
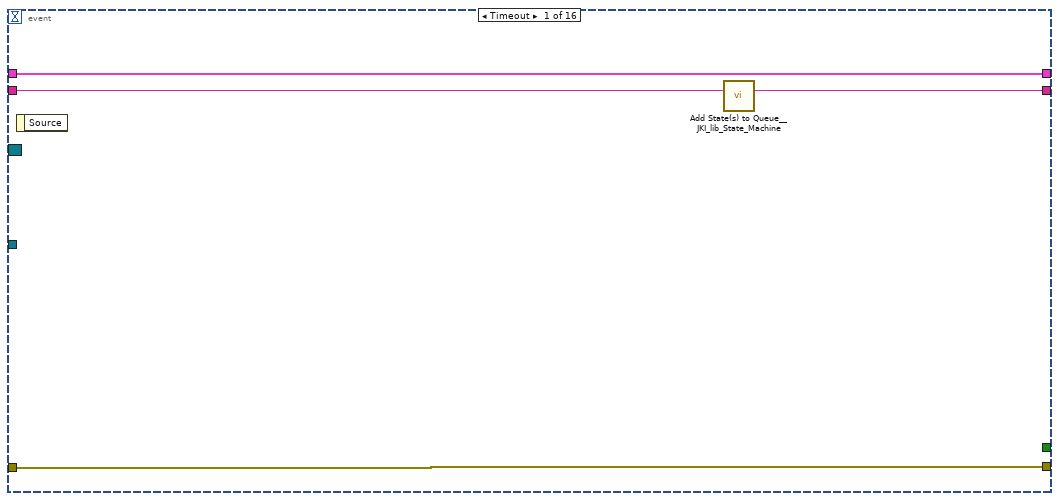
[diagram p12: hidden frame]
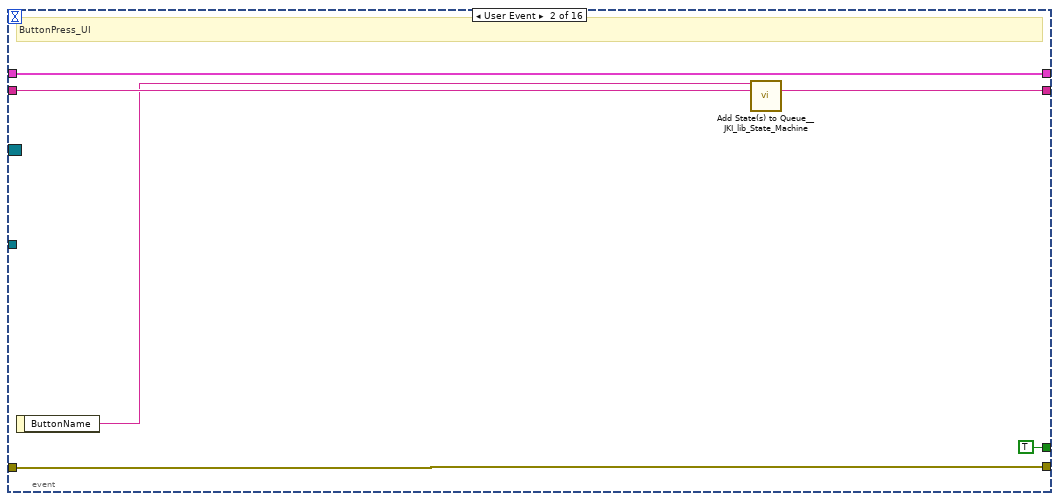
[diagram p13: hidden frame]
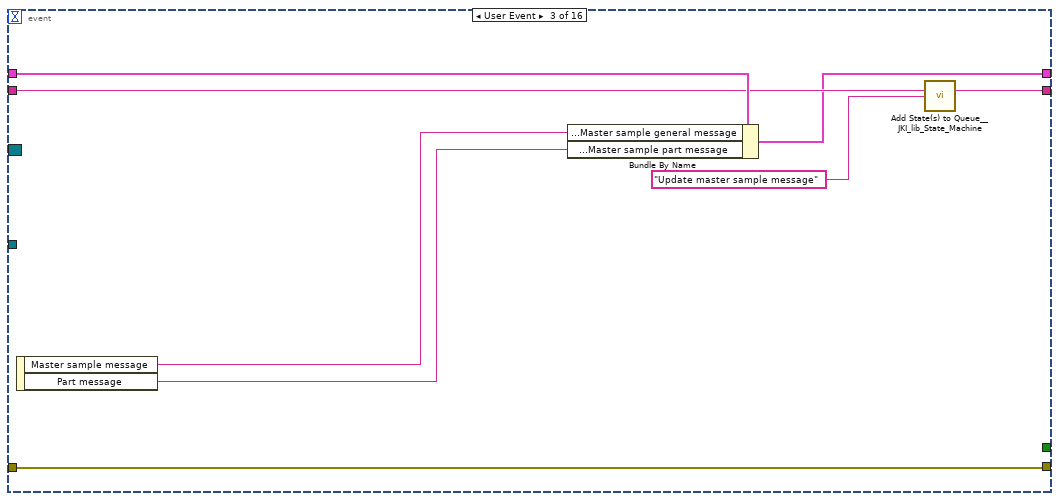
[diagram p14: hidden frame]
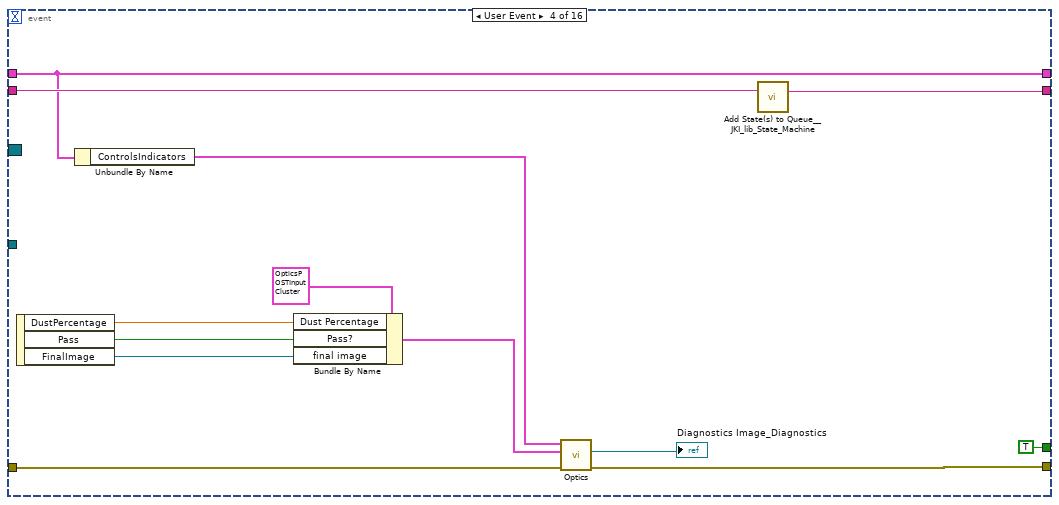
[diagram p15: hidden frame]
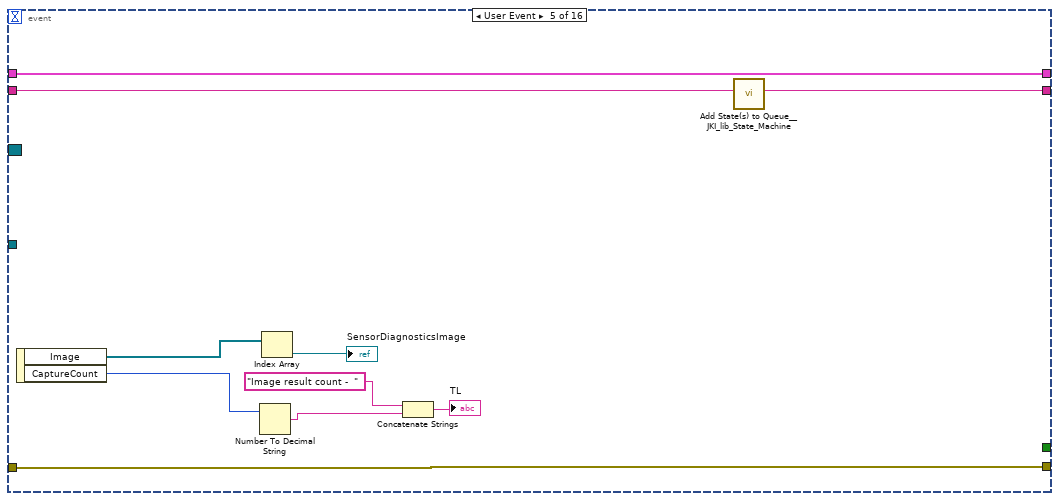
[diagram p16: hidden frame]
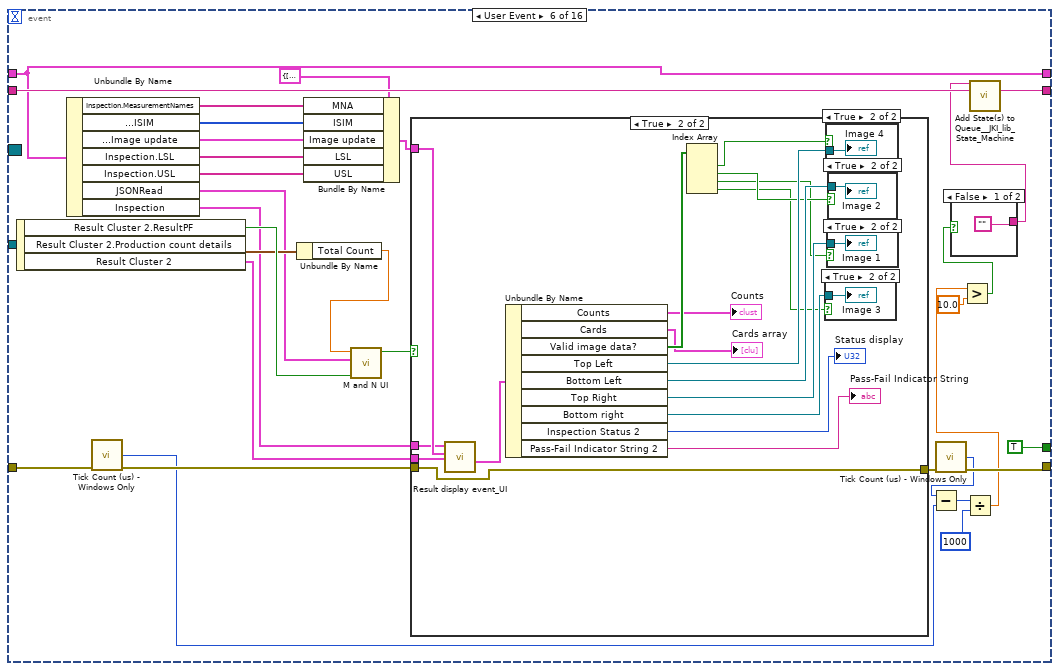
[diagram p17: hidden frame]
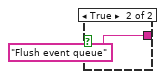
[diagram p18: hidden frame]
diagram:
  # "File path initialized in \"Data : Initialize\" state"
  n1 = flat-sequence {
    tunnel: "error in" -> [w24]
    tunnel: "ZenGage v3.0 UI in" -> [w27]
    tunnel: [w33] -> w17
    tunnel: [w32] -> w16
    tunnel: [w29] -> w15
    tunnel: [w28] -> w14
    tunnel: [w27] -> w13
    tunnel: [w30] -> w6
    tunnel: [w29] -> w5
    tunnel: [w28] -> w4
    tunnel: [w21] -> w3
    tunnel: [w19] -> w2
    tunnel: [w18] -> w1
    tunnel: w17 -> [w153]
    tunnel: w16 -> [w157]
    tunnel: w15 -> [w160]
    tunnel: w14 -> [w159]
    tunnel: w13 -> [w152]
    tunnel: [w158] -> w9
    tunnel: w6 -> [w156]
    tunnel: w5 -> [w155]
    tunnel: w4 -> [w154]
    tunnel: w3 -> [w150]
    tunnel: w2 -> [w148]
    tunnel: w1 -> [w147]
    frame #0 {
      # "Initialization (Reference bundling and event registration)"
      n2 = stacked-sequence {
        frame #0 {
          # "General"
        }
        frame #1 {
          # "Inspection"
        }
        frame #2 {
          # "Diagnostics"
        }
        frame #3 {
          # "Edit Tolerance Limits"
        }
        frame #4 {
          # "Master sample validation"
        }
      }
      n3 = stacked-sequence {
        tunnel: [_ _ _ w134 _] -> w36
        tunnel: [w73 _ _ _ _] -> w39
        tunnel: [_ w101 _ _ _] -> w38
        tunnel: [_ _ w119 _ _] -> w37
        tunnel: [_ _ _ _ w146] -> w20
        frame #0 {
          w63 = refnum<vi> refnum  # Zen Logo_Inspection
          # "General"
          n4 = control-ref of="Main Tab"() -> (w71:refnum<vi>)
          n5 = call <vilib>:"Application Directory.vi"() -> ("Application Directory"=w74:path)
          n6 = control-ref of="Analytics_subpanel"() -> (w64:refnum<vi>)
          n7 = control-ref of="Image 4"() -> (w69:refnum<vi>)
          n8 = control-ref of="Image 2"() -> (w68:refnum<vi>)
          n9 = control-ref of="Image 1"() -> (w66:refnum<vi>)
          n10 = control-ref of="Image 3"() -> (w65:refnum<vi>)
          n11 = control-ref of="Command Tab"() -> (w44:refnum<vi>)
          n12 = control-ref of="Tab Control"() -> (w48:refnum<vi>)
          n13 = control-ref of="Right Pane Tab"() -> (w60:refnum<vi>)
          n14 = control-ref of="Operator Name"() -> (w50:refnum<vi>)
          n15 = control-ref of="SoftwareExit"() -> (w62:refnum<vi>)
          n16 = control-ref of="Part Name"() -> (w52:refnum<vi>)
          n17 = control-ref of="Select message"() -> (w41:refnum<vi>)
          n18 = control-ref of="ok"() -> (w58:refnum<vi>)
          n19 = control-ref of="confirm"() -> (w57:refnum<vi>)
          n20 = control-ref of="reset"() -> (w56:refnum<vi>)
          n21 = control-ref of="change"() -> (w55:refnum<vi>)
          n22 = control-ref of="VERIFIED"() -> (w51:refnum<vi>)
          n23 = control-ref of="Total Count"() -> (w54:refnum<vi>)
          n24 = control-ref of="Reel Count"() -> (w53:refnum<vi>)
          n25 = call <vilib>:"Application Directory.vi"() -> ("Application Directory"=w78:path)
          n26 = Build Path(base path=w74, name or relative path="User Interface\\User Interface Actor\\SubVIs\\General\\LoadingBar_General_UI.vi") -> (appended path=w76:path)
          n27 = Build Path(base path=w78, name or relative path="ZenGage v3.0 UI\\ZenAnalytics\\SubVI\\Graph references\\Graph references(12 measurements)_Trend_Hist_test.vi") -> (appended path=w77:path)
          n28 = Insert Into Array(array=refnum<vi>[] [], new element #1=w69, new element #2=w68, new element #3=w66, new element #4=w65) -> (w59:refnum<vi>[])  [unwired: 1 in]
          n29 = control-ref of="Event  Reason  List"() -> (w49:refnum<vi>)
          n30 = Bundle By Name(cluster=T18 {"ok"=refnum, "confirm"=refnum, "reset"=refnum, "change"=refnum, "TOTAL COUNT"=refnum, "REEL COUNT"=refnum, "PART NAME"=refnum, "VERIFIED"=refnum, "OPERATOR NAME"=refnum, "Select message"=refnum} ("SelectionCluster"), "ok"=w58, "confirm"=w57, "reset"=w56, "change"=w55, "TOTAL COUNT"=w54, "REEL COUNT"=w53, "PART NAME"=w52, "VERIFIED"=w51, "OPERATOR NAME"=w50, "Select message"=w41) -> (w42:T18)
          n31 = Open VI Reference(vi path=w76) -> (vi reference=w61:refnum<vi>)  [unwired: 5 in, 1 out]
          n32 = Open VI Reference(vi path=w77) -> ()  [unwired: 5 in, 2 out]
          n33 = control-ref of="Event reason switching tab"() -> (w46:refnum<vi>)
          n34 = control-ref of="confirm_eventReason"() -> (w45:refnum<vi>)
          n35 = control-ref of="Event reason blink"() -> (w47:refnum<vi>)
          n36 = Bundle(cluster=T13 {"Main Tab"=refnum, "Inspection SubPanel_Inspection"=refnum, "Zen Logo_Inspection"=refnum, "SoftwareExit"=refnum, "Loading Bar VI Ref"=refnum, "Right Pane Tab"=refnum, "Image Reference array"=[], "Command tab"=refnum, "Inspection subTab control ref"=refnum, "SelectionCluster"={"ok"=refnum, "confirm"=refnum, "reset"=refnum, "change"=refnum, "TOTAL COUNT"=refnum, "REEL COUNT"=refnum, "PART NAME"=refnum, "VERIFIED"=refnum, "OPERATOR NAME"=refnum, "Select message"=refnum}, "Event  Reason  List"=refnum, "Event reason blink"=refnum, "Event reason switching tab"=refnum, "confirm_eventReason"=refnum} ("General"), "Main Tab"=w71, "Inspection SubPanel_Inspection"=w64, "Zen Logo_Inspection"=w63, "SoftwareExit"=w62, "Loading Bar VI Ref"=w61, "Right Pane Tab"=w60, "Image Reference array"=w59, "Command tab"=w44, "Inspection subTab control ref"=w48, "SelectionCluster"=w42, "Event  Reason  List"=w49, "Event reason blink"=w47, "Event reason switching tab"=w46, "confirm_eventReason"=w45) -> (w73:T13)
        }
        frame #1 {
          w85 = refnum<vi> refnum  # Analytics VI reference
          # "Inspection"
          n37 = control-ref of="Image label 2"() -> (w97:refnum<vi>)
          n38 = control-ref of="Image label 1"() -> (w98:refnum<vi>)
          n39 = control-ref of="Reel counts cluster"() -> (w79:refnum<vi>)
          n40 = control-ref of="Production counts clustwer"() -> (w80:refnum<vi>)
          n41 = control-ref of="Image label 3"() -> (w96:refnum<vi>)
          n42 = control-ref of="Run_Inspection"() -> (w93:refnum<vi>)
          n43 = control-ref of="Image label 4"() -> (w95:refnum<vi>)
          n44 = call <vilib>:"Application Directory.vi"() -> ("Application Directory"=w103:path)
          n45 = control-ref of="Pass-Fail Indicator String"() -> (w88:refnum<vi>)
          n46 = control-ref of="Status display"() -> (w94:refnum<vi>)
          n47 = control-ref of="Analytics_Inspection"() -> (w87:refnum<vi>)
          n48 = control-ref of="Pause_Inspection"() -> (w92:refnum<vi>)
          n49 = control-ref of="Stop_Inspection"() -> (w91:refnum<vi>)
          n50 = control-ref of="Settings_Inspection"() -> (w90:refnum<vi>)
          n51 = control-ref of="Cards array"() -> (w83:refnum<vi>)
          n52 = control-ref of="Counts"() -> (w84:refnum<vi>)
          n53 = Build Path(base path=w103, name or relative path="ZenGage v3.0 UI\\SubVIs\\Inspection\\Inspection Images\\Inspection(Simulate3images)_without Zoom Factor_Inspection_UI.vi") -> (appended path=w104:path)
          n54 = Insert Into Array(array=refnum<vi>[] [] ("Array"), new element #1=w98, new element #2=w97, new element #3=w96, new element #4=w95) -> (w86:refnum<vi>[])  [unwired: 1 in]
          n55 = Open VI Reference(vi path=w104) -> (vi reference=w89:refnum<vi>)  [unwired: 5 in, 1 out]
          n56 = Insert Into Array(array=refnum<vi>[] [] ("Counts array"), new element #1=w79, new element #2=w80) -> (w81:refnum<vi>[])  [unwired: 1 in]
          n57 = Bundle(cluster=T14 {"Inspection Status"=refnum, "Run_Inspection"=refnum, "Pause_Inspection"=refnum, "Stop_Inspection"=refnum, "Settings_Inspection"=refnum, "Inspection Images VI Ref"=refnum, "Pass-Fail Indicator String"=refnum, "Analytics_Inspection"=refnum, "Label array"=[], "Analytics VI\nreference"=refnum, "Counts"=refnum, "Cards array"=refnum, "Counts array"=[]} ("Inspection"), "Inspection Status"=w94, "Run_Inspection"=w93, "Pause_Inspection"=w92, "Stop_Inspection"=w91, "Settings_Inspection"=w90, "Inspection Images VI Ref"=w89, "Pass-Fail Indicator String"=w88, "Analytics_Inspection"=w87, "Label array"=w86, "Analytics VI\nreference"=w85, "Counts"=w84, "Cards array"=w83, "Counts array"=w81) -> (w101:T14)
        }
        frame #2 {
          # "Diagnostics"
          n58 = control-ref of="Select a diagnostics"() -> (w106:refnum<vi>)
          n59 = control-ref of="DUST INDICATOR"() -> (w117:refnum<vi>)
          n60 = control-ref of="logout_Diagnostics"() -> (w116:refnum<vi>)
          n61 = control-ref of="CAMERA STATUS\n       MESSAGE"() -> (w115:refnum<vi>)
          n62 = control-ref of="BUZZER OFF"() -> (w114:refnum<vi>)
          n63 = control-ref of="PAUSE"() -> (w113:refnum<vi>)
          n64 = control-ref of="STOP"() -> (w112:refnum<vi>)
          n65 = control-ref of="RUN"() -> (w111:refnum<vi>)
          n66 = control-ref of="Current\nDiagnostics\nStatus"() -> (w110:refnum<vi>)
          n67 = control-ref of="Select a part"() -> (w107:refnum<vi>)
          n68 = control-ref of="Diagnostics Image_Diagnostics"() -> (w108:refnum<vi>)
          n69 = control-ref of="Diagnostics Tab"() -> (w120:refnum<vi>)
          n70 = control-ref of="Diagnostics Status\nString"() -> (w109:refnum<vi>)
          n71 = control-ref of="Diagnostics Status\nString"() -> (w105:refnum<vi>)
          n72 = Bundle(cluster=T15 {"Diagnostics Tab"=refnum, "Dust indicator :"=refnum, "Logout_Diagnostics"=refnum, "CAMERA STATUS MESSAGE"=refnum, "BUZZER OFF"=refnum, "PAUSE"=refnum, "STOP"=refnum, "RUN"=refnum, "Current Diagnostics Status"=refnum, "Select a diagnostics"=refnum, "Diagnostics Status"=refnum, "Select a sub diagnostics"=refnum, "Optics img"=refnum, "Diagnostics Status\nString"=refnum} ("Diagnostics"), "Diagnostics Tab"=w120, "Dust indicator :"=w117, "Logout_Diagnostics"=w116, "CAMERA STATUS MESSAGE"=w115, "BUZZER OFF"=w114, "PAUSE"=w113, "STOP"=w112, "RUN"=w111, "Current Diagnostics Status"=w110, "Select a diagnostics"=w107, "Diagnostics Status"=w109, "Select a sub diagnostics"=w106, "Optics img"=w108, "Diagnostics Status\nString"=w105) -> (w119:T15)
        }
        frame #3 {
          # "Edit Tolerance Settings"
          n73 = control-ref of="Select a part"() -> (w128:refnum<vi>)
          n74 = control-ref of="Bias Correction"() -> (w125:refnum<vi>)
          n75 = control-ref of="Linearity Correction"() -> (w124:refnum<vi>)
          n76 = control-ref of="Restore to defaults_Edit Tolerance"() -> (w135:refnum<vi>)
          n77 = control-ref of="Tolerance Limits Listbox"() -> (w133:refnum<vi>)
          n78 = control-ref of="Measurement\nEnable"() -> (w139:refnum<vi>)
          n79 = control-ref of="Update List"() -> (w138:refnum<vi>)
          n80 = control-ref of="Save"() -> (w137:refnum<vi>)
          n81 = control-ref of="Logout_EditTolerance"() -> (w136:refnum<vi>)
          n82 = control-ref of="ETS tab"() -> (w131:refnum<vi>)
          n83 = control-ref of="Fail count reverse"() -> (w123:refnum<vi>)
          n84 = control-ref of="ETL count error message"() -> (w122:refnum<vi>)
          n85 = control-ref of="ETL help string"() -> (w121:refnum<vi>)
          n86 = control-ref of="Cluster of limits"() -> (w127:refnum<vi>)
          n87 = control-ref of="Factory reset"() -> (w130:refnum<vi>)
          n88 = control-ref of="Door Poka \nYoke"() -> (w129:refnum<vi>)
          n89 = control-ref of="Threshold limits"() -> (w126:refnum<vi>)
          n90 = Bundle(cluster=T16 {"Tolerance Limits Listbox"=refnum, "Enable Disable"=refnum, "Cluster of limits"=refnum, "Thresholds limits"=refnum, "Update List"=refnum, "Save"=refnum, "Back_Edit Tolerance"=refnum, "logout"=refnum, "Select a part"=refnum, "Bias Correction"=refnum, "Linearity Correction"=refnum, "Select a Rack"=refnum, "ETS tab"=refnum, "Factory reset"=refnum, "Door\nPoka Yoke"=refnum, "Fail count reverse"=refnum, "ETL count error message"=refnum, "ETL help string"=refnum} ("Edit Tolerance Limits"), "Tolerance Limits Listbox"=w133, "Enable Disable"=w139, "Cluster of limits"=w127, "Thresholds limits"=w126, "Update List"=w138, "Save"=w137, "Back_Edit Tolerance"=w135, "logout"=w136, "Select a part"=w128, "Bias Correction"=w125, "Linearity Correction"=w124, "ETS tab"=w131, "Factory reset"=w130, "Door\nPoka Yoke"=w129, "Fail count reverse"=w123, "ETL count error message"=w122, "ETL help string"=w121) -> (w134:T16)  [unwired: 1 in]
        }
        frame #4 {
          # "Master sample"
          n91 = control-ref of="Master sample message"() -> (w145:refnum<vi>)
          n92 = control-ref of="Next"() -> (w144:refnum<vi>)
          n93 = control-ref of="Repeat"() -> (w143:refnum<vi>)
          n94 = control-ref of="Master sample tab"() -> (w141:refnum<vi>)
          n95 = control-ref of="Master sample part message"() -> (w140:refnum<vi>)
          n96 = Bundle By Name(cluster=T17 {"Master sample message"=refnum, "Master sample tab"=refnum, "Next"=refnum, "Repeat"=refnum, "Master sample part message"=refnum} ("Master sample"), "Master sample message"=w145, "Master sample tab"=w141, "Next"=w144, "Repeat"=w143, "Master sample part message"=w140) -> (w146:T17)
        }
      }
      n97 = Unbundle By Name(w27) -> ("Slave Loop"=w25:T36, "SendClusterData"=w19:refnum<user-event>, "SendClusterData to MainLoop"=w18:refnum<user-event>)
      n98 = Unbundle By Name(w27) -> ("User Events Cluster_UI"=w35:T37, "SendClusterData to MainLoop"=w26:refnum<user-event>)
      n99 = Create User Event(user event datatype=w27, error in=w24) -> (error out=w34:errorcluster)  [unwired: 1 out]
      n100 = Create User Event(user event datatype=w27, error in=w24) -> (error out=w31:errorcluster)  [unwired: 1 out]
      n101 = call <vilib>:"Read Caller Enqueuer.vi"("Actor"=w27) -> ("Caller Enqueuer"=w29:refnum<class "Message Enqueuer.lvclass">)  [unwired: 10 in]
      n102 = register-events(error in=w24, w35, w26) -> (reference out=w33:refnum<event-registration>, error out=w23:errorcluster)  [unwired: 1 in]
      n103 = register-events(error in=w24, w25) -> (reference out=w21:refnum<event-registration>, error out=w22:errorcluster)  [unwired: 1 in]
      n104 = call <vilib>:"Read Self Enqueuer.vi"("Actor"=w27) -> ("Self Enqueuer"=w28:refnum<class "Message Enqueuer.lvclass">)  [unwired: 10 in]
      n105 = Merge Errors(w23, w22, w34, w31) -> (w32:errorcluster)
      n106 = Bundle By Name(cluster=T12 {"General"={"Main Tab"=refnum, "Inspection SubPanel_Inspection"=refnum, "Zen Logo_Inspection"=refnum, "SoftwareExit"=refnum, "Loading Bar VI Ref"=refnum, "Right Pane Tab"=refnum, "Image Reference array"=[], "Command tab"=refnum, "Inspection subTab control ref"=refnum, "SelectionCluster"={"ok"=refnum, "confirm"=refnum, "reset"=refnum, "change"=refnum, "TOTAL COUNT"=refnum, "REEL COUNT"=refnum, "PART NAME"=refnum, "VERIFIED"=refnum, "OPERATOR NAME"=refnum, "Select message"=refnum}, "Event  Reason  List"=refnum, "Event reason blink"=refnum, "Event reason switching tab"=refnum, "confirm_eventReason"=refnum}, "Inspection"={"Inspection Status"=refnum, "Run_Inspection"=refnum, "Pause_Inspection"=refnum, "Stop_Inspection"=refnum, "Settings_Inspection"=refnum, "Inspection Images VI Ref"=refnum, "Pass-Fail Indicator String"=refnum, "Analytics_Inspection"=refnum, "Label array"=[], "Analytics VI\nreference"=refnum, "Counts"=refnum, "Cards array"=refnum, "Counts array"=[]}, "Diagnostics"={"Diagnostics Tab"=refnum, "Dust indicator :"=refnum, "Logout_Diagnostics"=refnum, "CAMERA STATUS MESSAGE"=refnum, "BUZZER OFF"=refnum, "PAUSE"=refnum, "STOP"=refnum, "RUN"=refnum, "Current Diagnostics Status"=refnum, "Select a diagnostics"=refnum, "Diagnostics Status"=refnum, "Select a sub diagnostics"=refnum, "Optics img"=refnum, "Diagnostics Status\nString"=refnum}, "Edit Tolerance Limits"={"Tolerance Limits Listbox"=refnum, "Enable Disable"=refnum, "Cluster of limits"=refnum, "Thresholds limits"=refnum, "Update List"=refnum, "Save"=refnum, "Back_Edit Tolerance"=refnum, "logout"=refnum, "Select a part"=refnum, "Bias Correction"=refnum, "Linearity Correction"=refnum, "Select a Rack"=refnum, "ETS tab"=refnum, "Factory reset"=refnum, "Door\nPoka Yoke"=refnum, "Fail count reverse"=refnum, "ETL count error message"=refnum, "ETL help string"=refnum}, "Master sample"={"Master sample message"=refnum, "Master sample tab"=refnum, "Next"=refnum, "Repeat"=refnum, "Master sample part message"=refnum}} ("Controls and Indicators\nReferences"), "General"=w39, "Inspection"=w38, "Diagnostics"=w37, "Edit Tolerance Limits"=w36, "Master sample"=w20) -> (w30:T12)
    }
    frame #1 {
      w149 = T38 {"JSONRead"={"ConfigurationFilePaths"={"Default JSON Path in"=path "", "Rack Controller Override JSON file path in"=path "", "Algorithm Overrride JSON file path in "=path ""}, "ConfigurationVariants"={"Default JSON \nVariant"=variant(cluster{"Inspection States":enum16{"PreSelect", "Back _Inspection", "Analytics", "Ready To Run", "Ready To Insert", "Enable All buttons", "Disable All Buttons", "Settings", "Select", "Stop", "Pause", "Inspect"}} {"Inspection States"=enum."PreSelect"}), "Algorithm Override\nJSON Variant"=variant(cluster{"Diagnostics States":enum16{"Enable All", "Camera Optics Fail", "Loading Bar", "Camera Optics", "Motor", "Arduino", "POST Done", "POST"}} {"Diagnostics States"=enum."Enable All"}), "Rack Controller Override\nJSON Variant"=variant(cluster{"Edit Limits":enum16{"Update List"}, "Enable Disable Measurements":enum16{"Back to Edit Tolerance"}, "Page Select":enum16{"Edit Tolerance Limits", "Enable Disable Buttons"}} {"Edit Limits"=enum."Update List", "Enable Disable Measurements"=enum."Back to Edit Tolerance", "Page Select"=enum."Edit Tolerance Limits"})}, "ConfigurationCluster"={"UIParameters"={"SpecificationVersion"="", "Title"="", "NumberOfImagesToBeDisplayed"=0.0, "ImageCountWindow"=0.0, "FontName"="", "FontSize"=0.0, "CustomerLogoFilePath"="", "ZentronLogoFilePath"="", "CompatibleSoftwareVersions"=[], "CameraLabelMapping"=[], "ImageIndicatorLayouts"=[], "SoftwareButtonLabels"={"SelectLabel"="", "RunLabel"="", "PauseLabel"="", "StopLabel"=""}, "DiagnosticsParameters"={"CameraOpticsDiagnostics"={"Label"="", "CameraLabelsList"=[]}, "ArduinoDiagnostics"={"Label"=""}, "MotorDiagnostics"={"Label"=""}, "ReelerMotor"={"Label"=""}, "TowerLampDiagnostics"={"Label"=""}, "TriggerSensor"={"Label"="", "SensorsList"=[]}, "HardwareButtonDiagnostics"={"Label"=""}, "MasterSampleDiagnostics"={"Label"=""}}, "DieIdParameters"={"DefaultDieId"="", "DieIdsList"=[]}, "EventReasonsList"={"Pause"=[], "Stop"=[], "FailPause"=[], "Ignored"=[], "DefaultEventReason"=""}, "StampingMachineIds"=[], "ErrorPopupStrings"=[]}}}, "Inspection"={"Inspection After Stop"=FALSE, "IsPaused"=FALSE, "Camera Names"=[], "Fail Array"=[], "Reel Number"=0, "Image details_init"=[], "LSL"=[], "USL"=[], "Max limits"={"Production max"=0, "Reel max"=0}, "parts List"=[], "#Racks"=0, "MeasurementNames"=[], "Reel complete"=FALSE, "Fail event reason list"=[]}, "Diagnostics"={"Selection Done?"=FALSE, "Diagnostics details"={"Diagnostics names"={"Main diagnostics"=[], "Sub diagnostics names"={"Camera optics"=[], "Trigger sensor"=[]}}, "Diagnostics labels"={"Main diagnostics"=[], "Sub diagnostics names"={"Camera optics"=[], "Trigger sensor"=[]}}}, "DiagnosticsFeatures"={"ArduinoDiagnostics"=FALSE, "MotorDiagnostics"=FALSE, "CameraOpticsDiagnostics"=FALSE, "ReelerMotor"=FALSE, "HardwareButtonDiagnostics"=FALSE, "TriggerSensor"=FALSE, "TowerLampDiagnostics"=FALSE, "MasterSampleDiagnostics"=FALSE}, "SelectedDiagnostics"=""}, "EditToleranceSettings"={"Input ListBox"={"Measurement Values"=[], "Cluster of Limits"={"LSL"=0.0, "USL"=0.0, "LCL"=0.0, "UCL"=0.0}, "Rack Selection"=enum."Both Racks", "M and N Array"=[], "Ticked Measurement Index"=[], "Measurements Enabled"=[], "Current Active Position"={"Horizontal"=0, "Vertical"=0}, "Current ticked measurement"=0.0}, "Saved?"=FALSE, "IsETLSelected"=FALSE, "IsPartSelected"=FALSE}, "ControlsIndicators"={"General"={"Main Tab"=refnum, "Inspection SubPanel_Inspection"=refnum, "Zen Logo_Inspection"=refnum, "SoftwareExit"=refnum, "Loading Bar VI Ref"=refnum, "Right Pane Tab"=refnum, "Image Reference array"=[], "Command tab"=refnum, "Inspection subTab control ref"=refnum, "SelectionCluster"={"ok"=refnum, "confirm"=refnum, "reset"=refnum, "change"=refnum, "TOTAL COUNT"=refnum, "REEL COUNT"=refnum, "PART NAME"=refnum, "VERIFIED"=refnum, "OPERATOR NAME"=refnum, "Select message"=refnum}, "Event  Reason  List"=refnum, "Event reason blink"=refnum, "Event reason switching tab"=refnum, "confirm_eventReason"=refnum}, "Inspection"={"Inspection Status"=refnum, "Run_Inspection"=refnum, "Pause_Inspection"=refnum, "Stop_Inspection"=refnum, "Settings_Inspection"=refnum, "Inspection Images VI Ref"=refnum, "Pass-Fail Indicator String"=refnum, "Analytics_Inspection"=refnum, "Label array"=[], "Analytics VI\nreference"=refnum, "Counts"=refnum, "Cards array"=refnum, "Counts array"=[]}, "Diagnostics"={"Diagnostics Tab"=refnum, "Dust indicator :"=refnum, "Logout_Diagnostics"=refnum, "CAMERA STATUS MESSAGE"=refnum, "BUZZER OFF"=refnum, "PAUSE"=refnum, "STOP"=refnum, "RUN"=refnum, "Current Diagnostics Status"=refnum, "Select a diagnostics"=refnum, "Diagnostics Status"=refnum, "Select a sub diagnostics"=refnum, "Optics img"=refnum, "Diagnostics Status\nString"=refnum}, "Edit Tolerance Limits"={"Tolerance Limits Listbox"=refnum, "Enable Disable"=refnum, "Cluster of limits"=refnum, "Thresholds limits"=refnum, "Update List"=refnum, "Save"=refnum, "Back_Edit Tolerance"=refnum, "logout"=refnum, "Select a part"=refnum, "Bias Correction"=refnum, "Linearity Correction"=refnum, "Select a Rack"=refnum, "ETS tab"=refnum, "Factory reset"=refnum, "Door\nPoka Yoke"=refnum, "Fail count reverse"=refnum, "ETL count error message"=refnum, "ETL help string"=refnum}, "Master sample"={"Master sample message"=refnum, "Master sample tab"=refnum, "Next"=refnum, "Repeat"=refnum, "Master sample part message"=refnum}}, "AdditionalFeatures"={"Cp Cpk details"={"CpCpkData"=[], "Cp Cpk popup"=refnum}, "Popup"={"Restore main tab"="", "Popup data"={"Loading bar data"={"Open?"=FALSE, "Display string"=""}, "Pop-up"={"Pop-up Type"=enum."Open Logo Display", "Title"="", "Message"="", "Button 1 Text"="", "Button 2 Text"="", "Show Close? T/F"=FALSE, "Title Blink? T/F"=FALSE, "Title Blink Colour"=0}}}, "DynamicImageHandling"={"Image update"=[], "RBCIA"=[], "ISIM"=[], "Camera labels list"=[], "Enable DIH?"=FALSE, "Init DIH params?"=FALSE}, "PageHandling"={"Previous State"={"Inspection"={"Inspection States"=enum."PreSelect"}, "Diagnostics"={"Diagnostics States"=enum."Enable All"}, "Edit Tolerance"={"Edit Limits"=enum."Update List", "Enable Disable Measurements"=enum."Back to Edit Tolerance", "Page Select"=enum."Edit Tolerance Limits"}, "Page Select"=enum."Edit Tolerance"}, "Current state"="", "Previous control access state"="Diagnostics"}, "Core"={"Current VI Reference"=refnum, "Close Panel on Exit?"=FALSE}, "SlaveLoopData"={"EnableShortKeyPress"=FALSE, "Point32"={"Horizontal"=0, "Vertical"=0}}, "Chosen event reason"="", "Master sample validation"={"Master sample general message"="", "Master sample part message"=""}, "Fail Ignore Count Reversal"={"Production ignored count"=0, "Reel ignored count"=0}}}
      # "Actor Core Main"
      n107 = call <vilib>:"Add State(s) to Queue__JKI_lib_State_Machine.vi"("State(s) in (\"\")"="Macro: Initialize") -> ("States Out"=w162:string)  [unwired: 14 in]
      n108 = while "JKI - String-Based Queued State Machine (Basic) v1.0" {
        shift-right: [w165] -> _
        shift-left: w149 -> [w183]
        shift-right: [w169] -> w164
        shift-left: w157 -> [w180]
        shift-right: [w185] -> _
        shift-left: w162 -> [w186]
        tunnel: w153 -> [w181]
        tunnel: w156 -> [w176]
        tunnel: w152 -> [w179]
        tunnel: w155 -> [w178]
        tunnel: w154 -> [w177]
        shift-right: [w172] -> _
        shift-left: "" -> [w174]
        tunnel: w148 -> [w167]
        stop <- w184 stop-if-true
        w182 = -1  # Timeout
        # "Actor core main loop"
        n109 = call <vilib>:"Parse State Queue__JKI_lib_State_Machine.vi"("State Queue"=w186, "Error In (no error)"=w180) -> ("Remaining States"=w173:string, "Current State"=w171:string, "Arguments"=w187:string)  [unwired: 11 in]
        n110 = case shown="\"Read init JSON params\"" w171 {
          selector: w171 -> [_ _ w440 _ _ _ _ _ _ _ _ _ _ _ _ _ _ _ _ _ _ _ _ _ _ _ _ _ _ _ _ _ _ _ _ _ _ _ _ _ _ w969 _ _ _ _ _ _ _ _ _ _ _ _ _ _ _ _ _ _ _ _ _ _ _ _ _ _ _ _]
          tunnel: w173 -> [w203 w438 w443 w461 w480 w490 w494 w513 w519 w523 w527 w533 w544 w570 w575 w585 w589 w600 w619 w629 w643 w650 w656 w677 w687 w736 w769 w781 w799 w809 w817 w829 w833 w852 w863 w874 w882 w890 w933 w939 w951 w974 w990 w994 w1005 w1016 w1020 w1040 w1082 w1096 w1110 w1115 w1123 w1138 w1181 w1209 w1221 w1259 w1284 w1288 w1297 w1349 w1363 w1368 w1377 w1392 w1397 w1412 w1421 w1433]
          tunnel: w187 -> [_ _ _ _ _ _ _ _ _ _ _ w529 w539 _ _ _ _ _ _ w626 _ _ _ w670 w679 _ _ w777 w798 _ _ _ _ _ _ _ _ w886 _ _ _ _ _ _ _ _ _ w1028 _ _ _ _ w1119 _ _ _ w1223 _ _ _ w1296 _ _ _ _ _ _ _ _ w1435]
          tunnel: w183 -> [w201 w435 w439 w453 w467 w486 w491 w508 w514 w520 w524 w528 w538 w567 w571 w576 w586 w595 w617 w625 w631 w646 w652 w669 w682 w727 w765 w778 w795 w807 w812 w821 w836 w843 w862 w872 w879 w885 w931 w934 w946 w966 w986 w991 w1001 w1013 w1017 w1036 w1078 w1094 w1108 w1113 w1121 w1133 w1161 w1198 w1219 w1252 w1279 w1286 w1292 w1334 w1361 w1366 w1373 w1391 w1396 w1411 w1419 w1428]
          tunnel: [w200 w436 w445 w459 errorcluster {"status"=FALSE, "code"=0, "source"=""} ("error out") w488 w492 w509 w515 w521 w525 w530 w541 w568 w573 w583 w587 w591 w616 w627 w640 w647 w653 w676 w685 w722 w766 w779 w792 w808 w815 w827 w840 w844 w856 w865 w880 w887 w914 w935 w947 w964 w987 w992 w996 w1006 w1018 w1039 w1083 w1091 w1109 w1114 w1122 w1136 w1141 w1211 w1224 w1255 w1281 w1287 w1294 w1341 w1362 w1367 w1371 w1390 w1395 w1405 w1420 w1424] -> w170
          tunnel: w180 -> [w199 w436 w444 w459 w476 w488 w492 w510 w516 w521 w525 w531 w542 w568 w573 w583 w587 w598 w615 w627 w641 w648 w654 w675 w684 w735 w767 w780 w788 w808 w816 w828 w841 w846 w859 w866 w880 w888 w902 w936 w948 w961 w988 w992 w999 w1012 w1018 w1050 w1083 w1095 w1109 w1114 w1122 w1137 w1156 w1200 w1226 w1256 w1282 w1287 w1295 w1337 w1362 w1367 w1372 w1390 w1395 w1400 w1420 w1432]
          tunnel: [w202 w437 w442 w460 w479 w489 w493 w512 w518 w522 w526 w532 w543 w569 w574 w584 w588 w599 w618 w628 w642 w649 w655 w678 w686 w737 w768 w782 w800 w810 w818 w830 w832 w853 w864 w873 w881 w889 w932 w938 w950 w973 w989 w993 w1004 w1015 w1019 w1051 w1084 w1097 w1111 w1116 w1124 w1139 w1182 w1208 w1228 w1260 w1285 w1289 w1298 w1350 w1364 w1369 w1378 w1393 w1398 w1413 w1422 w1437] -> w185
          tunnel: [_ _ _ _ _ TRUE _ _ _ _ _ _ _ _ _ _ _ _ _ _ _ _ _ _ _ _ _ _ _ _ _ _ _ _ _ _ _ _ _ _ _ _ _ _ _ _ _ _ _ _ _ _ _ _ _ _ _ _ _ _ _ _ _ _ _ _ _ _ _ w1434] -> w184
          tunnel: w182 -> [w198 _ _ _ _ _ _ _ _ _ _ _ _ _ _ _ _ _ _ _ _ _ _ _ _ _ _ _ _ _ _ _ _ _ _ _ _ _ _ _ _ _ _ _ _ _ _ _ _ _ _ _ _ _ _ _ _ _ _ _ _ _ _ _ _ _ _ _ _ _]
          tunnel: w181 -> [w196 _ _ _ _ _ _ _ _ _ _ _ _ _ _ _ _ _ _ _ _ _ _ _ _ _ _ _ _ _ _ _ _ _ _ _ _ _ _ _ _ _ _ _ _ _ _ _ _ _ _ _ _ w1135 _ _ w1225 w1257 _ _ _ _ _ _ _ _ _ _ _ w1429]
          tunnel: w179 -> [_ _ _ _ _ _ _ _ _ _ _ _ _ _ _ _ _ _ _ _ _ _ _ _ _ _ w763 _ _ _ w814 _ _ _ _ _ _ _ _ _ _ _ _ _ _ _ _ _ _ _ _ _ _ _ w1155 _ w1217 w1251 _ _ _ _ _ _ _ _ _ _ _ w1426]
          tunnel: [w197 w435 w439 w450 w467 w486 w491 w504 w514 w520 w524 w528 w538 w567 w571 w576 w586 w594 w617 w624 w631 w646 w651 w668 w681 w727 w764 w778 w795 w807 w812 w821 w836 w842 w862 w872 w879 w884 w931 w934 w946 w966 w986 w991 w1001 w1013 w1017 w1035 w1075 w1093 w1108 w1112 w1120 w1133 w1159 w1196 w1218 w1249 w1279 w1286 w1291 w1332 w1361 w1366 w1374 w1391 w1396 w1411 w1419 w1430] -> w166
          tunnel: w178 -> [w195 _ _ _ w466 _ _ _ _ _ _ _ _ _ _ _ _ _ _ _ w630 _ _ _ _ w726 _ _ _ _ _ w819 _ _ _ _ _ _ _ _ _ _ _ _ _ _ _ w1034 _ _ _ _ _ _ _ _ _ _ _ _ _ _ _ _ _ _ _ _ _ _]
          tunnel: w177 -> [_ _ _ _ _ _ _ _ _ _ _ _ _ _ _ _ _ _ _ _ _ _ _ _ _ _ _ _ _ _ _ w820 _ _ _ _ _ _ _ _ _ _ _ _ _ _ _ w1030 _ _ _ _ _ _ _ _ _ _ _ _ w1290 _ _ _ _ _ _ _ _ _]
          tunnel: w176 -> [_ _ _ _ _ _ _ w507 _ _ _ _ _ _ _ _ _ _ _ _ _ _ _ _ _ _ _ _ _ _ _ _ _ _ _ _ _ _ _ _ _ _ _ _ _ _ _ _ _ _ _ _ _ _ _ _ _ _ _ _ _ _ _ _ _ _ _ _ _ _]
          tunnel: [w194 _ _ _ _ _ _ _ _ _ _ _ _ _ _ _ _ TRUE _ _ _ _ _ TRUE _ _ _ _ _ _ _ _ _ _ _ _ _ TRUE TRUE _ _ _ _ _ _ _ _ _ _ _ _ _ _ _ _ _ TRUE TRUE _ _ _ _ _ _ _ _ _ _ _ _] -> w168
          frame "", "Event Structure", "Idle" {
            n111 = event shown="[8] <User Events Cluster_UI.SystemInfo_UI>: User Event" {
              selector: w196 -> [_ _ _ _ _ _ _ _ _ _ _ _ _ _ _ _]
              dyn-events: _ -> [_ _ _ _ _ _ _ _ _ _ _ _ _ _ _ _]
              timeout: w198 -> [_ _ _ _ _ _ _ _ _ _ _ _ _ _ _ _]
              tunnel: w203 -> [w207 w212 w219 w233 w242 w273 w314 w332 w347 w353 w389 w394 w401 w413 w421 w430]
              tunnel: [w206 w213 w220 w234 w243 w274 w315 w332 w346 w354 w390 w395 w402 w414 w420 w429] -> w202
              tunnel: w201 -> [w204 w210 w221 w224 w240 w248 w308 w330 w342 w356 w385 w397 w403 w406 w418 w423]
              tunnel: [w205 w209 w215 w232 w241 w263 w307 w328 w335 w361 w384 w393 w398 w415 w419 w427] -> w200
              tunnel: w199 -> [w205 w209 w215 w227 w241 w268 w307 w329 w338 w362 w384 w393 w398 w415 w419 w428]
              tunnel: [w204 w210 w216 w224 w240 w248 w300 w331 w349 w355 w385 w396 w400 w405 w418 w422] -> w197
              tunnel: w195 -> [_ _ _ _ _ _ _ _ _ _ _ _ _ _ _ _]
              tunnel: [_ TRUE _ TRUE _ TRUE _ _ _ _ _ _ _ TRUE _ _] -> w194
              event Timeout {
                n112 = event-data() -> ()  [unwired: 1 in, 1 out]
                n113 = call <vilib>:"Add State(s) to Queue__JKI_lib_State_Machine.vi"("State(s) in (\"\")"=w207) -> ("States Out"=w206:string)  [unwired: 14 in]
              }
              event User Event {
                # "ButtonPress_UI"
                n114 = event-data() -> ("ButtonName"=w211:string)  [unwired: 1 in]
                n115 = call <vilib>:"Add State(s) to Queue__JKI_lib_State_Machine.vi"("State(s) in Front (\"\")"=w211, "State(s) in (\"\")"=w212) -> ("States Out"=w213:string)  [unwired: 13 in]
              }
              event User Event {
                n116 = event-data() -> ("Master sample message"=w218:string, "Part message"=w217:string)  [unwired: 1 in]
                n117 = Bundle By Name(cluster=w221, "AdditionalFeatures.Master sample validation.Master sample general message"=w218, "AdditionalFeatures.Master sample validation.Master sample part message"=w217) -> (w216:T38)
                n118 = call <vilib>:"Add State(s) to Queue__JKI_lib_State_Machine.vi"("State(s) in (\"\")"=w219, "State(s) at Back (\"\")"="Update master sample message" ("State(s) in Front (\"\")")) -> ("States Out"=w220:string)  [unwired: 13 in]
              }
              event User Event {
                n119 = event-data() -> ("DustPercentage"=w229:dbl, "Pass"=w226:bool, "FinalImage"=w225:T3)  [unwired: 1 in]
                n120 = Unbundle By Name(w224) -> ("ControlsIndicators"=w223:T12)
                n121 = Bundle By Name(cluster=T19 {"Dust Percentage"=0.0, "Diagnostics Sstatus string"="", "Pass?"=FALSE, "final image"=refnum} ("Optics_Diagnostics_UI"), "Dust Percentage"=w229, "Pass?"=w226, "final image"=w225) -> (w228:T19)
                n122 = call "Optics.vi"("error in (no error)"=w227, "Optics POST Input Cluster"=w228, "Controls and Indicators\nReferences"=w223) -> ("error out"=w232:errorcluster, "Diagnostics Image_Diagnostics"=→"Diagnostics Image_Diagnostics":T3)  [unwired: 7 in]
                n123 = call <vilib>:"Add State(s) to Queue__JKI_lib_State_Machine.vi"("State(s) in (\"\")"=w233) -> ("States Out"=w234:string)  [unwired: 14 in]
              }
              event User Event {
                n124 = event-data() -> ("Image"=w244:T3[], "CaptureCount"=w239:u64)  [unwired: 1 in]
                n125 = Number To Decimal String(number=w239) -> (decimal integer string=w237:string)  [unwired: 1 in]
                n126 = Index Array(array=w244) -> (element=→"SensorDiagnosticsImage":T3)  [unwired: 1 in]
                n127 = Concatenate Strings(T20 "Image result count -  " ("TL"), w237) -> (→"TL":string)
                n128 = call <vilib>:"Add State(s) to Queue__JKI_lib_State_Machine.vi"("State(s) in (\"\")"=w242) -> ("States Out"=w243:string)  [unwired: 14 in]
              }
              event User Event {
                n129 = event-data() -> ("Result Cluster 2.ResultPF"=w272:bool, "Result Cluster 2.Production count details"=w250:T49, "Result Cluster 2"=w269:T50)  [unwired: 1 in]
                n130 = Unbundle By Name(w248) -> ("Inspection.MeasurementNames"=w260:string[], "AdditionalFeatures.DynamicImageHandling.ISIM"=w259:u8[], "AdditionalFeatures.DynamicImageHandling.Image update"=w258:cluster{"Rack Id":i32, "Update image":bool[]}[], "Inspection.LSL"=w252:string[], "Inspection.USL"=w251:string[], "JSONRead"=w247:T39, "Inspection"=w246:T41)
                n131 = call "Tick Count (us) - Windows Only.vi"("error in (no error)"=w268) -> ("micorsecond timer value"=w261:u64, "error out"=w267:errorcluster)  [unwired: 13 in]
                n132 = Unbundle By Name(w250) -> ("Total Count"=w271:dbl)
                n133 = Bundle By Name(cluster=T21 {"MNA"=[], "ISIM"=[], "Image update"=[{"Rack Id"=0, "Update image"=[TRUE, TRUE, FALSE, FALSE]}, {"Rack Id"=1, "Update image"=[FALSE, FALSE, TRUE, TRUE]}], "Current rack Id"=0, "LSL"=[], "USL"=[]} ("Result cluster details"), "MNA"=w260, "ISIM"=w259, "Image update"=w258, "LSL"=w252, "USL"=w251) -> (w253:T21)
                n134 = call "M and N UI.vi"("Result Count"=w271, "JSON Read"=w247, "Result PF"=w272) -> ("Display UI Result?"=w270:bool)  [unwired: 7 in]
                n135 = case shown="True" w270 {
                  tunnel: w267 -> [w277 w281]
                  tunnel: [w277 w281] -> w264
                  tunnel: w269 -> [_ w278]
                  tunnel: w253 -> [_ w280]
                  tunnel: w246 -> [_ w279]
                  frame False {
                  }
                  frame True {
                    n136 = call "Result display event_UI.vi"("Result Cluster"=w278, "Result cluster details"=w280, "InspectionCluster in"=w279) -> ("output cluster"=w291:T51)  [unwired: 7 in, 1 out]
                    n137 = Unbundle By Name(w291) -> ("Counts"=→"Counts":T52, "Cards"=→"Cards array":T53, "Valid image data?"=w289:bool[], "Top Left"=w295:T3, "Bottom Left"=w294:T3, "Top Right"=w292:T3, "Bottom right"=w290:T3, "Inspection Status 2"=→"Status display":u32, "Pass-Fail Indicator String 2"=→"Pass-Fail Indicator String":string)
                    n138 = Index Array(array=w289) -> (element #1=w288:bool, element #2=w287:bool, element #3=w286:bool, element #4=w285:bool)  [unwired: 4 in]
                    n139 = case shown="True" w285 {
                      tunnel: w290 -> [_ w296]
                      frame False {
                      }
                      frame True {
                        "Image 3" <- w296
                      }
                    }
                    n140 = case shown="True" w288 {
                      tunnel: w295 -> [_ w299]
                      frame False {
                      }
                      frame True {
                        "Image 4" <- w299
                      }
                    }
                    n141 = case shown="True" w286 {
                      tunnel: w292 -> [_ w297]
                      frame False {
                      }
                      frame True {
                        "Image 1" <- w297
                      }
                    }
                    n142 = case shown="True" w287 {
                      tunnel: w294 -> [_ w298]
                      frame False {
                      }
                      frame True {
                        "Image 2" <- w298
                      }
                    }
                  }
                }
                n143 = call "Tick Count (us) - Windows Only.vi"("error in (no error)"=w264) -> ("micorsecond timer value"=w262:u64, "error out"=w263:errorcluster)  [unwired: 13 in]
                n144 = Subtract(x=w262, y=w261) -> (x-y=w265:u64)
                n145 = Divide(x=w265, y=u64 1000) -> (x/y=w257:dbl)
                n146 = Greater?(x=w257, y=10.0) -> (0:w254:bool)
                n147 = case shown="False" w254 {
                  tunnel: ["" "Flush event queue"] -> w255
                  frame False {
                  }
                  frame True {
                  }
                }
                n148 = call <vilib>:"Add State(s) to Queue__JKI_lib_State_Machine.vi"("State(s) in Front (\"\")"=w255, "State(s) in (\"\")"=w273) -> ("States Out"=w274:string)  [unwired: 13 in]
              }
              event User Event {
                n149 = event-data() -> ("Pop-up Type"=w304:T35, "Title"=w313:string, "Message"=w312:string, "Button 1 Text"=w311:string, "Button 2 Text"=w310:string, "Show Close? T/F"=w309:bool, "Title Blink? T/F"=w306:bool, "Title Blink Colour"=w305:u32, "Message"=w302:string)  [unwired: 1 in]
                n150 = Bundle By Name(cluster=w308, "AdditionalFeatures.Popup.Popup data.Pop-up.Pop-up Type"=w304, "JSONRead.ConfigurationCluster.UIParameters.Title"=w313, "AdditionalFeatures.Popup.Popup data.Pop-up.Message"=w312, "AdditionalFeatures.Popup.Popup data.Pop-up.Button 1 Text"=w311, "AdditionalFeatures.Popup.Popup data.Pop-up.Button 2 Text"=w310, "AdditionalFeatures.Popup.Popup data.Pop-up.Show Close? T/F"=w309, "AdditionalFeatures.Popup.Popup data.Pop-up.Title Blink? T/F"=w306, "AdditionalFeatures.Popup.Popup data.Pop-up.Title Blink Colour"=w305, "AdditionalFeatures.Popup.Popup data.Loading bar data.Display string"=w302) -> (w301:T38)
                n151 = case shown="\"Close Loading Bar\"" w304 {
                  tunnel: ["Display loading bar>>Open" ("State(s) in Front (\"\")") "Display loading bar>>Close" ("State(s) in Front (\"\")") "Display popup" ("State(s) in Front (\"\")")] -> w303
                  tunnel: w301 -> [w318 w321 w324]
                  tunnel: [w317 w320 w324] -> w300
                  frame "Open Loading Bar" {
                    n152 = Bundle By Name(cluster=w318, "AdditionalFeatures.Popup.Popup data.Loading bar data.Open?"=TRUE ("Loading bar data.Open?")) -> (w317:T38)
                  }
                  frame "Close Loading Bar" {
                    n153 = Bundle By Name(cluster=w321, "AdditionalFeatures.Popup.Popup data.Loading bar data.Open?"=FALSE ("Loading bar data.Open?")) -> (w320:T38)
                  }
                  frame "Close Logo Display", Default {
                  }
                }
                n154 = call <vilib>:"Add State(s) to Queue__JKI_lib_State_Machine.vi"("State(s) in Front (\"\")"=w303, "State(s) in (\"\")"=w314) -> ("States Out"=w315:string)  [unwired: 13 in]
              }
              event User Event {
                # "GetAnalyticsVI_UI"
                n155 = event-data() -> ("AnalyticsVIRefnum"=w327:refnum<vi>)  [unwired: 1 in]
                n156 = Unbundle By Name(w330) -> ("ControlsIndicators.General.Inspection SubPanel_Inspection"=w326:refnum<vi>)
                n157 = invoke class="SubPnl" method="Insert VI"(reference=w326, error in=w329, "VI Ref"=w327) -> (error out=w328:errorcluster)  [unwired: 1 in, 3 out]
                n158 = Bundle By Name(cluster=w330, "ControlsIndicators.Inspection.Analytics VI\nreference"=w327) -> (w331:T38)
              }
              event User Event {
                n159 = event-data() -> ("DiagnosticsFeatures"=w343:T54, "UserInterfaceButtonVisibilty.DynamicImageHandlingEnable"=w350:bool, "Parts List"=w348:T55, "UserInterfaceButtonVisibilty.Door Poka Yoke"=w334:bool, "Analytics enabled"=w339:bool)  [unwired: 1 in]
                n160 = Unbundle By Name(w342) -> ("ControlsIndicators.Edit Tolerance Limits.Door\nPoka Yoke"=w344:refnum<vi>, "ControlsIndicators.Inspection.Analytics_Inspection"=w340:refnum<vi>)
                n161 = Not(x=w334) -> (.not. x?=w333:bool)
                n162 = for {
                  tunnel: w348 -> [w352] mode=indexing
                  tunnel: [w351] -> w341 mode=indexing
                  workers-P: _ -> [_]
                  n163 = Unbundle By Name(w352) -> ("Part name"=w351:string)
                }
                n164 = property class="Bool (strict)"(reference=w344, error in=w338, "Value"=w333) -> (error out=w336:errorcluster)  [unwired: 1 out]
                n165 = property class="Bool (strict)"(reference=w340, error in=w338, "Visible"=w339) -> (error out=w337:errorcluster)  [unwired: 1 out]
                n166 = call <vilib>:"Add State(s) to Queue__JKI_lib_State_Machine.vi"("State(s) in Front (\"\")"="Populate diagnostics list\nPopulate partslist" ("State(s) in Front (\"\")"), "State(s) in (\"\")"=w347) -> ("States Out"=w346:string)  [unwired: 13 in]
                n167 = Merge Errors(w336, w337) -> (w335:errorcluster)
                n168 = Bundle By Name(cluster=w342, "AdditionalFeatures.DynamicImageHandling.Enable DIH?"=w350, "Diagnostics.DiagnosticsFeatures"=w343, "Inspection.parts List"=w341) -> (w349:T38)
              }
              event User Event {
                n169 = event-data() -> ("CameraNames"=w359:string[], "MeasurementNames"=w358:string[], "RackId"=w360:u8, "SpecValues"=w357:T56)  [unwired: 1 in]
                n170 = in-place {
                  in-place-border: w362 -> [w363]
                  in-place-border: [w363] -> w361
                  in-place-border: w360 -> [w374]
                  in-place-border: w359 -> [w373]
                  in-place-border: w358 -> [w368]
                  in-place-border: w357 -> [w371]
                  # "code modified (24-07-2018)\nnumber of racks"
                  n171 = in-place-cluster #1(w356) -> ("AdditionalFeatures.DynamicImageHandling.Enable DIH?"=w364:bool, "Inspection.Image details_init"=w365:T57)  [unwired: 4 out]
                  n172 = for {
                    tunnel: w371 -> [w383] mode=indexing
                    tunnel: [w378] -> w369 mode=indexing
                    tunnel: [w377] -> w366 mode=indexing
                    workers-P: _ -> [_]
                    n173 = Unbundle By Name(w383) -> ("LSL"=w382:dbl, "USL"=w381:dbl)
                    n174 = Number To Fractional String(number=w382, precision (6)=i16 3) -> (F-format string=w378:string)  [unwired: 2 in]
                    n175 = Number To Fractional String(number=w381, precision (6)=i16 3) -> (F-format string=w377:string)  [unwired: 2 in]
                  }
                  n176 = Bundle By Name(cluster=T22 {"Camera names"=[], "Rack Id 2"=0, "Measurement names"=[], "Number of racks"=0, "Tolerance limits"=[]} ("Input event data"), "Camera names"=w373, "Measurement names"=w368, "Rack Id 2"=w374, "Number of racks"=u8 1) -> (w375:T22)
                  n177 = call "Post-select init.vi"("Init DIH params?"=w364, "Input event data"=w375, "Inspection.Image details_init"=w365) -> ("Number of racks"=w367:u8, "Inspection.Image details_init"=w370:T57)  [unwired: 7 in]
                  n178 = in-place-cluster #1("AdditionalFeatures.DynamicImageHandling.Enable DIH?"=w364, "Inspection.Image details_init"=w370, "Inspection.MeasurementNames"=w368, "Inspection.LSL"=w369, "Inspection.#Racks"=w367, "Inspection.USL"=w366) -> (w355:T38)
                }
                n179 = call <vilib>:"Add State(s) to Queue__JKI_lib_State_Machine.vi"("State(s) in (\"\")"=w353) -> ("States Out"=w354:string)  [unwired: 14 in]
              }
              event User Event {
                n180 = event-data() -> ("EventState"=w387:string)  [unwired: 1 in]
                n181 = Concatenate Strings("DisplayEventReason>>", w387) -> (w386:string)
                n182 = call <vilib>:"Add State(s) to Queue__JKI_lib_State_Machine.vi"("State(s) in Front (\"\")"=w386, "State(s) in (\"\")"=w389) -> ("States Out"=w390:string)  [unwired: 13 in]
              }
              event User Event {
                n183 = event-data() -> ("CpCpk data"=w391:string[][])  [unwired: 1 in]
                n184 = Bundle By Name(cluster=w397, "AdditionalFeatures.Cp Cpk details.CpCpkData"=w391) -> (w396:T38)
                n185 = call <vilib>:"Add State(s) to Queue__JKI_lib_State_Machine.vi"("State(s) in Front (\"\")"="Display CpCpk popup" ("State(s) in Front (\"\")"), "State(s) in (\"\")"=w394) -> ("States Out"=w395:string)  [unwired: 13 in]
              }
              event "UpdateImagingViews": Value Change {
                n186 = event-data() -> ()  [unwired: 1 in, 1 out]
                n187 = Bundle By Name(cluster=w403, "JSONRead.ConfigurationCluster.UIParameters.ImageIndicatorLayouts"="JSONRead.ConfigurationCluster.UIParameters.ImageIndicatorLayouts") -> (w400:T38)
                n188 = call <vilib>:"Add State(s) to Queue__JKI_lib_State_Machine.vi"("State(s) in (\"\")"=w401) -> ("States Out"=w402:string)  [unwired: 14 in]
              }
              event User Event {
                n189 = event-data() -> ("JSONRead"=w412:T39, "Inspection"=w411:T41, "Diagnostics"=w410:T42, "EditToleranceSettings"=w409:T43, "ControlsIndicators"=w408:T12, "AdditionalFeatures"=w407:T58)  [unwired: 1 in]
                n190 = Bundle By Name(cluster=w406, "JSONRead"=w412, "Inspection"=w411, "Diagnostics"=w410, "EditToleranceSettings"=w409, "ControlsIndicators"=w408, "AdditionalFeatures"=w407) -> (w405:T38)
                n191 = call <vilib>:"Add State(s) to Queue__JKI_lib_State_Machine.vi"("State(s) in (\"\")"=w413) -> ("States Out"=w414:string)  [unwired: 14 in]
              }
              event Panel Close? {
                n192 = event-data() -> ()  [unwired: 1 in, 1 out]
                n193 = call <vilib>:"Add State(s) to Queue__JKI_lib_State_Machine.vi"("State(s) in Front (\"\")"="Macro: Exit", "State(s) in (\"\")"=w421) -> ("States Out"=w420:string)  [unwired: 13 in]
                n194 = event-data("Discard?"=TRUE) -> ()  [unwired: 1 in, 1 out]
              }
              event "Image label 2", "Image label 3", "Image label 1", "Image label 4": Value Change {
                n195 = event-data() -> ("CtlRef"=w426:refnum<vi>, "NewVal"=w424:string)  [unwired: 1 in, 4 out]
                n196 = property class="CmbBox"(reference=w426, error in=w428) -> (error out=w427:errorcluster, "Label.Text"=w425:string)  [unwired: 1 out]
                n197 = in-place {
                  in-place-border: w425 -> [w434]
                  in-place-border: w424 -> [w433]
                  n198 = in-place-cluster #2(w423) -> ("AdditionalFeatures.DynamicImageHandling"=w431:T59)
                  n199 = call "Camera indicator mapping.vi"("Dynamic image update params in"=w431, "Selected imaging view name"=w433, "Selected label name"=w434) -> ("Dynamic image update params out"=w432:T60)  [unwired: 8 in]
                  n200 = in-place-cluster #2("AdditionalFeatures.DynamicImageHandling"=w432) -> (w422:T38)
                }
                n201 = call <vilib>:"Add State(s) to Queue__JKI_lib_State_Machine.vi"("State(s) in (\"\")"=w430) -> ("States Out"=w429:string)  [unwired: 14 in]
              }
            }
          }
          frame "---------- Core ----------" {
            # "Do not put any code in this frame.\n(it is a separator no-op)"
            n202 = call <vilib>:"Add State(s) to Queue__JKI_lib_State_Machine.vi"("State(s) in (\"\")"=w438) -> ("States Out"=w437:string)  [unwired: 14 in]
          }
          frame Default {
            w448 = 42 items=["No error", "Argument error", "Memory is full", "Out of zone", "End of file", "File already open", "Generic file I/O error", "File not found", "File permission error", "Disk is full", "Duplicate path", "Too many files open", "System feature not enabled", "Resource file not found", "Cannot add resource", "Resource not found", "Image not found", "Image memory error", "Pen does not exist", "Config type invalid", "Config token not found", "Config parse error", "Config memory error", "Bad external code format", "Bad external code offset", "External code not present", "Null window", "Destroy window error", "Null menu", "Print aborted", "Bad print record", "Print driver error", "Windows error during printing", "Memory error during printing", "Print dialog error", "Generic print error", "Invalid device refnum", "Device not found", "Device parameter error", "Device unit error", "Cannot open device", "Device call aborted", "Generic error", "Cancelled by user", "Object ID too low", "Object ID too high", "Object not in heap", "Unknown heap", "Unknown object (invalid DefProc)", "Unknown object (DefProc not in table)", "Message out of range", "Invalid (null) method", "Unknown message", "Manager call not supported", "Bad address", "Network operation in progress", "Network operation timed out", "Connection is busy", "Network attribute not supported", "Network error", "Address in use", "System out of memory", "Connection aborted", "Connection refused", "Not connected", "Already connected", "Connection closed", "Initialization error (interapplication manager)", "Bad occurrence", "Wait on unbound occurrence handler", "Occurrence queue overflow", "Datalog type conflict", "Unused", "Unrecognized type (interapplication manager)", "Memory corrupt", "Failed to make temporary DLL", "Old CIN version", "Drag socket not found", "Failed to load drop-object", "Failed to register OLE object", "Failed to release OLE object", "Format specifier type mismatch", "Unknown format specifier", "Too few format specifiers", "Too many format specifiers", "Scan failed", "Newer CIN version", "Error converting to variant", "Runtime menu error", "Password tampered", "Variant attribute not found", "Incompatible variant data type", "Event data is not available", "Event Store is not present", "Occurrence is not found", "Event Queue is not created", "Event info is not available", "Refnum passed is NULL", "Error retrieving Class GUID", "Error retrieving CoClass GUID", "Error retrieving TypeLib GUID.", "Bad built application magic bytes.", "Specific driver is different from the specific driver associated with the Logical Name.", "There is no session opened to the class driver.", "Max Error", "MAX - Error with config objects", "MAX - Error loading configuration", "MAX - Group not supported"]
            # "Current State"
            # "Do not delete, rename, or modify this frame.\n(this is used to capture unhandled states and typos)"
            # "Handle mistyped state name (developer tool)"
            n203 = Format Into String(format string="Software Exception: Unhandled State \"%s\"." ("message"), error in=w444, w440) -> (resulting string=w447:string, error out=w446:errorcluster)  [unwired: 1 in]
            n204 = call <vilib>:"Error Cluster From Error Code.vi"("show call chain? (False)"=TRUE, "error in (no error)"=w446, "error message (\"\")"=w447, "error code (0)"=w448) -> ("error out"=w445:errorcluster)  [unwired: 5 in]
            n205 = call <vilib>:"Add State(s) to Queue__JKI_lib_State_Machine.vi"("State(s) in (\"\")"=w443) -> ("States Out"=w442:string)  [unwired: 14 in]
          }
          frame "Initialize Core Data" {
            # "Do not delete, rename, or modify this frame.\n(this is used to determine panel behavior on exit)"
            # "originally closed?"
            # "exe?"
            # "If panel starts closed or is an EXE, then close it when we exit"
            n206 = property class="VI"() -> ("Front Panel.Open"=w458:bool)  [unwired: 2 in, 2 out]
            n207 = property class="App"() -> ("App.Kind"=w457:T23)  [unwired: 2 in, 2 out]
            n208 = control-ref of="Current VI Reference"() -> (w451:refnum<vi>)
            n209 = Not(x=w458) -> (.not. x?=w455:bool)
            n210 = Equal?(x=w457, y=T23."Run Time System" ("Application:Kind")) -> (x = y?=w454:bool)
            n211 = Or(x=w455, y=w454) -> (x .or. y?=w452:bool)
            n212 = Bundle By Name(cluster=w453, "AdditionalFeatures.Core.Current VI Reference"=w451, "AdditionalFeatures.Core.Close Panel on Exit?"=w452) -> (w450:T38)
            n213 = call <vilib>:"Add State(s) to Queue__JKI_lib_State_Machine.vi"("State(s) in (\"\")"=w461) -> ("States Out"=w460:string)  [unwired: 14 in]
          }
          frame "Error Handler" {
            # "Output.vi_code modified (02-08-2018)"
            # "Handle any errors here.\nYou can also output any states to clean-up after errors occur"
            n214 = Unbundle By Name(w476) -> ("code"=w464:i32, "source"=w470:string)
            n215 = case shown="Default" w464 {
              tunnel: ["InspectionUIError_0xF601\n[JKI Serilization / Generate user event]" ("Error Message") "InspectionUIError_0xF60F\n[Unknown error]" ("Error Message") "InspectionUIError_0xF603\n[JSON variant to data]" ("Error Message") "InspectionUIError_0xF602\n[Property Node]" ("Error Message") "InspectionUIError_0xF600\n[Loading bar reference]" ("Error Message")] -> w472
              frame 1 {
                # "JKI Serialization error / Generate User Event"
              }
              frame Default {
                # "Unknown error"
              }
              frame 91 {
                # "JSON Variant to Data"
              }
              frame 1055 {
                # "File Read Error"
              }
              frame 1149 {
                # "Closed loading bar reference can be closed again"
              }
            }
            n216 = call <vilib>:"Clear Errors.vi"("error in (no error)"=w476) -> ("error out"=w475:errorcluster)  [unwired: 5 in, 1 out]
            n217 = One Button Dialog(message=w470, button name ("OK")="Ok") -> ()  [unwired: 1 out]
            n218 = Bundle By Name(cluster=T25 {"Acknowledgement_SM"={"Enqueuer"=refnum, "VIReference"=refnum, "VIName"=""}, "Button name"="", "PartDetails"={"PartName"="", "ConnectorsInReel"=0, "TotalCounts"=0, "OperatorName"="", "StampingMachineID"=0}, "SensorName"="", "CameraName"="", "PopupFeedbackDetails"={"Pop-up Type"=enum."Open Logo Display", "Message"="", "Pressed Button"=""}, "EventResponse"="", "ErrorMessage"="", "FailCountIgnore"={"ReelIgnoreCount"=0, "ProductionIgnoreCount"=0}} ("OutputDetails"), "ErrorMessage"=w472) -> (w473:T25)
            n219 = Number To Decimal String(number=w464) -> (decimal integer string=w463:string)  [unwired: 1 in]
            n220 = call "Output_UI.vi"("OutputDetails"=w473, "error in"=w475, "Functionality"=Output_choice."SendErrorDetails" ("Functionality 2"), "Testbench"=TRUE, "SMEnqueuer"=w466) -> ()  [unwired: 6 in, 1 out]
            n221 = Concatenate Strings("Error occured : " ("message"), w463) -> (w462:string)
            n222 = One Button Dialog(message=w462) -> ()  [unwired: 1 in, 1 out]
            n223 = call <vilib>:"Add State(s) to Queue__JKI_lib_State_Machine.vi"("State(s) in Front (\"\")"="/* Post Error States", "State(s) in (\"\")"=w480) -> ("States Out"=w479:string)  [unwired: 13 in]
          }
          frame "Exit" {
            # "Do not put any code in this frame.\n(No errors that occur here will be handled.)"
            n224 = call <vilib>:"Add State(s) to Queue__JKI_lib_State_Machine.vi"("State(s) in (\"\")"=w490) -> ("States Out"=w489:string)  [unwired: 14 in]
          }
          frame "---------- Initialize ----------" {
            # "Do not put any code in this frame.\n(It is a separator no-op. You can make a copy of this frame to create a new Data frame)"
            n225 = call <vilib>:"Add State(s) to Queue__JKI_lib_State_Machine.vi"("State(s) in (\"\")"=w494) -> ("States Out"=w493:string)  [unwired: 14 in]
          }
          frame "Data: Initialize" {
            w503 = T61 {"Default JSON Path in"=path "", "Rack Controller Override JSON file path in"=path "", "Algorithm Overrride JSON file path in "=path ""}  # JSONRead.ConfigurationFilePaths
            w506 = T62 {"Current VI Reference"=refnum, "Close Panel on Exit?"=FALSE}  # Core
            n226 = call <vilib>:"Application Directory.vi"() -> ("Application Directory"=w501:path)
            n227 = Build Path(base path=w501, name or relative path="Configuration file\\Zengage System Parameters.json") -> (appended path=w497:path)
            n228 = Build Path(base path=w501, name or relative path="Configuration file\\Rack Controller Parameters Override.json") -> (appended path=w496:path)
            n229 = Build Path(base path=w501, name or relative path="Configuration file\\Algorithm Parameters Override.json") -> (appended path=w495:path)
            n230 = Bundle By Name(cluster=w503, "Default JSON Path in"=w497, "Rack Controller Override JSON file path in"=w496, "Algorithm Overrride JSON file path in"=w495) -> (w502:T61)
            n231 = call <vilib>:"Add State(s) to Queue__JKI_lib_State_Machine.vi"("State(s) in (\"\")"=w513, "State(s) at Back (\"\")"="Send acknowledge\nPart selection>>Initialize\nUpdate user screen interaction loop\nDisableAllButtons\nRead init JSON params\nPart selection>>Enable selection\nInitialize images" ("State(s) in Front (\"\")")) -> ("States Out"=w512:string)  [unwired: 13 in]
            n232 = Bundle By Name(cluster=w508, "ControlsIndicators"=w507, "AdditionalFeatures.Core"=w506, "JSONRead.ConfigurationFilePaths"=w502) -> (w505:T38)
            n233 = call "JSON read.vi"("error in (no error)"=w510, "ZenGage v3.0 UI in"=w505) -> ("error out"=w509:errorcluster, "ZenGage v3.0 UI in"=w504:T38)  [unwired: 8 in]
          }
          frame "Data: Cleanup" {
            n234 = Unbundle By Name(w514) -> ("AdditionalFeatures.Core.Current VI Reference"=w517:refnum<vi>)
            n235 = Close Reference(reference=w517, error in (no error)=w516) -> (error out=w515:errorcluster)
            n236 = call <vilib>:"Add State(s) to Queue__JKI_lib_State_Machine.vi"("State(s) in (\"\")"=w519) -> ("States Out"=w518:string)  [unwired: 14 in]
          }
          frame "---------- UI ----------" {
            n237 = call <vilib>:"Add State(s) to Queue__JKI_lib_State_Machine.vi"("State(s) in (\"\")"=w523) -> ("States Out"=w522:string)  [unwired: 14 in]
          }
          frame "UI: Initialize" {
            # "Initialize the User Interface, here.\n(this is called automatically, by the Macro: Init)"
            n238 = call <vilib>:"Add State(s) to Queue__JKI_lib_State_Machine.vi"("State(s) in (\"\")"=w527) -> ("States Out"=w526:string)  [unwired: 14 in]
          }
          frame "UI: Cursor Set" {
            # "Argument"
            n239 = case shown="\"Busy\"" w529 {
              tunnel: w531 -> [w535 w537]
              tunnel: [w534 w536] -> w530
              frame "Idle", Default {
                n240 = call <vilib>:"Unset Busy.vi"("error in (no error)"=w535) -> ("error out"=w534:errorcluster)  [unwired: 10 in]
              }
              frame "Busy" {
                n241 = call <vilib>:"Set Busy.vi"("error in (no error)"=w537) -> ("error out"=w536:errorcluster)  [unwired: 9 in, 1 out]
              }
            }
            n242 = call <vilib>:"Add State(s) to Queue__JKI_lib_State_Machine.vi"("State(s) in (\"\")"=w533) -> ("States Out"=w532:string)  [unwired: 14 in]
          }
          frame "UI: Front Panel State" {
            # "Argument"
            # "Set Front Panel Open or Closed\n(Usage: \"UI: Front Panel State >> Open|Close\")"
            n243 = Unbundle By Name(w538) -> ("AdditionalFeatures.Core.Current VI Reference"=w540:refnum<vi>)
            n244 = case shown="\"Open\", Default" w539 {
              tunnel: w542 -> [w548 w561]
              tunnel: [w550 w562] -> w541
              tunnel: w540 -> [w549 w559]
              frame "Open", Default {
                n245 = property class="VI"(reference=w549, error in=w548) -> (reference out=w546:refnum<vi>, error out=w547:errorcluster, "Front Panel.Open"=w545:bool)
                n246 = case shown="False" w545 {
                  tunnel: [w553 w556] -> w550
                  tunnel: w547 -> [w552 w556]
                  tunnel: w546 -> [w551 _]
                  frame False {
                    n247 = invoke class="VI" method="FP.Open"(reference=w551, error in=w552, "Activate"=TRUE, "State"=T27."Standard") -> (error out=w553:errorcluster)  [unwired: 1 in, 4 out]
                  }
                  frame True {
                  }
                }
              }
              frame "Close" {
                n248 = property class="VI"(reference=w559, error in=w561) -> (reference out=w558:refnum<vi>, error out=w560:errorcluster, "Front Panel.Open"=w557:bool)
                n249 = case shown="True" w557 {
                  tunnel: [w563 w566] -> w562
                  tunnel: w560 -> [w563 w565]
                  tunnel: w558 -> [_ w564]
                  frame False {
                  }
                  frame True {
                    n250 = invoke class="VI" method="FP.Close"(reference=w564, error in=w565) -> (error out=w566:errorcluster)  [unwired: 1 in, 2 out]
                  }
                }
              }
            }
            n251 = call <vilib>:"Add State(s) to Queue__JKI_lib_State_Machine.vi"("State(s) in (\"\")"=w544) -> ("States Out"=w543:string)  [unwired: 14 in]
          }
          frame "---------- Macro ----------" {
            n252 = call <vilib>:"Add State(s) to Queue__JKI_lib_State_Machine.vi"("State(s) in (\"\")"=w570) -> ("States Out"=w569:string)  [unwired: 14 in]
          }
          frame "Macro: Initialize" {
            w572 = "Data: Initialize\nInitialize Core Data\nUI: Initialize\nUI: Front Panel State >> Close"  # Data: Initialize Initialize Core Data UI: Initialize UI: Front Panel State >> Close
            # "Initialization Macro\n(This is called once, when the VI starts)"
            n253 = call <vilib>:"Add State(s) to Queue__JKI_lib_State_Machine.vi"("State(s) in Front (\"\")"=w572, "State(s) in (\"\")"=w575) -> ("States Out"=w574:string)  [unwired: 13 in]
          }
          frame "Macro: Exit" {
            n254 = Unbundle By Name(w576) -> ("AdditionalFeatures.Core.Close Panel on Exit?"=w582:bool)
            n255 = Select(t="UI: Front Panel State >> Close", s=w582, f="") -> (s? t:f=w579:string)
            n256 = call <vilib>:"Add State(s) to Queue__JKI_lib_State_Machine.vi"("State(s) in (\"\")"=w579, "State(s) at Back (\"\")"="Data: Cleanup\nExit") -> ("States Out"=w577:string)  [unwired: 13 in]
            n257 = call <vilib>:"Add State(s) to Queue__JKI_lib_State_Machine.vi"("State(s) in Front (\"\")"=w577, "State(s) in (\"\")"=w585) -> ("States Out"=w584:string)  [unwired: 13 in]
          }
          frame "---------- Common Access ----------" {
            n258 = call <vilib>:"Add State(s) to Queue__JKI_lib_State_Machine.vi"("State(s) in (\"\")"=w589) -> ("States Out"=w588:string)  [unwired: 14 in]
          }
          frame "Initialize images" {
            n259 = call "IMAQ Create"("Image Name"="empty image", "error in (no error)"=w598) -> ("New Image"=w590:T3, "error out"=w593:errorcluster)  [unwired: 3 in]
            n260 = in-place {
              in-place-border: w590 -> [w605]
              in-place-border: w593 -> [w603]
              in-place-border: [w601] -> w592
              n261 = in-place-cluster #3(w595) -> ("ControlsIndicators.General.Image Reference array"=w604:refnum<vi>[])
              n262 = for {
                tunnel: w605 -> [w608]
                tunnel: w604 -> [w610] mode=indexing
                shift-right: [w607] -> w601
                shift-left: w603 -> [w609]
                tunnel: [w606] -> w602 mode=indexing
                n263 = property class="ImageControl"(reference=w610, error in=w609, "Value"=w608) -> (reference out=w606:refnum<vi>, error out=w607:errorcluster)
              }
              n264 = in-place-cluster #3("ControlsIndicators.General.Image Reference array"=w602) -> (w594:T38)
            }
            n265 = call "IMAQ Dispose"("Image"=w590, "error in (no error)"=w592) -> ("error out"=w591:errorcluster)  [unwired: 4 in]
            n266 = call <vilib>:"Add State(s) to Queue__JKI_lib_State_Machine.vi"("State(s) in (\"\")"=w600) -> ("States Out"=w599:string)  [unwired: 14 in]
          }
          frame "CloseCpCpkPopup" {
            n267 = Unbundle By Name(w617) -> ("AdditionalFeatures.Cp Cpk details.Cp Cpk popup"=w613:refnum<vi>)
            n268 = property class="VI"(reference=w613, error in=w615) -> (reference out=w611:refnum<vi>, error out=w614:errorcluster, "FP.State"=w612:T27)
            n269 = case shown="\"Standard\", Default" w612 {
              tunnel: w614 -> [w620 w623]
              tunnel: [w620 w622] -> w616
              tunnel: w611 -> [_ w621]
              frame "Closed" {
              }
              frame "Standard", Default {
                n270 = invoke class="VI" method="FP.Close"(reference=w621, error in=w623) -> (error out=w622:errorcluster)  [unwired: 1 in, 2 out]
              }
            }
            n271 = call <vilib>:"Add State(s) to Queue__JKI_lib_State_Machine.vi"("State(s) in (\"\")"=w619) -> ("States Out"=w618:string)  [unwired: 14 in]
          }
          frame "StateChange" {
            # "Template Separator\n(You can make a copy of, or modify, this frame)"
            n272 = Bundle By Name(cluster=w625, "AdditionalFeatures.PageHandling.Current state"=w626) -> (w624:T38)
            n273 = call <vilib>:"Add State(s) to Queue__JKI_lib_State_Machine.vi"("State(s) in (\"\")"=w629) -> ("States Out"=w628:string)  [unwired: 14 in]
          }
          frame "Display popup" {
            # "popup_code modified(02-08-2018)"
            n274 = Unbundle By Name(w631) -> ("AdditionalFeatures.Popup.Popup data.Pop-up"=w638:T47)
            n275 = call "main pop-up.vi"("error in"=w641, "Pop-up Input"=w638) -> ("error out"=w637:errorcluster, "Pop-up Output"=w634:T63)  [unwired: 8 in]
            n276 = Bundle By Name(cluster=T25 {"Acknowledgement_SM"={"Enqueuer"=refnum, "VIReference"=refnum, "VIName"=""}, "Button name"="", "PartDetails"={"PartName"="", "ConnectorsInReel"=0, "TotalCounts"=0, "OperatorName"="", "StampingMachineID"=0}, "SensorName"="", "CameraName"="", "PopupFeedbackDetails"={"Pop-up Type"=enum."Open Logo Display", "Message"="", "Pressed Button"=""}, "EventResponse"="", "ErrorMessage"="", "FailCountIgnore"={"ReelIgnoreCount"=0, "ProductionIgnoreCount"=0}} ("OutputDetails"), "PopupFeedbackDetails"=w634) -> (w635:T25)
            n277 = call "Output_UI.vi"("OutputDetails"=w635, "error in"=w637, "Functionality"=Output_choice."SendPopupResponse", "Testbench"=TRUE, "SMEnqueuer"=w630) -> ("error out"=w640:errorcluster)  [unwired: 6 in]
            n278 = call <vilib>:"Add State(s) to Queue__JKI_lib_State_Machine.vi"("State(s) in Front (\"\")"="Idle" ("State(s) in Front (\"\")"), "State(s) in (\"\")"=w643) -> ("States Out"=w642:string)  [unwired: 13 in]
          }
          frame "DisableAllButtons" {
            # "Template Copyright © 2015 JKI - http://jki.net/state-machine"
            n279 = Unbundle By Name(w646) -> ("ControlsIndicators"=w645:T12, "AdditionalFeatures.PageHandling.Current state"=w644:string)
            n280 = call "Disable All Buttons_UI.vi"("error in (no error)"=w648, "state"=w644, "ZenGage v3.0 UI in"=w645) -> ("error out"=w647:errorcluster)  [unwired: 8 in]
            n281 = call <vilib>:"Add State(s) to Queue__JKI_lib_State_Machine.vi"("State(s) in (\"\")"=w650) -> ("States Out"=w649:string)  [unwired: 14 in]
          }
          frame "Display loading bar" {
            n282 = in-place {
              in-place-border: w654 -> [w665]
              in-place-border: [w664] -> w653
              n283 = in-place-cluster #4(w652) -> ("AdditionalFeatures.PageHandling.Previous control access state"=w661:string, "AdditionalFeatures.Popup.Popup data.Loading bar data.Open?"=w660:bool, "AdditionalFeatures.Popup.Popup data.Loading bar data.Display string"=w659:string, "AdditionalFeatures.Popup.Restore main tab"=w663:string, "ControlsIndicators"=w658:T12)
              n284 = call "Display loading bar.vi"("Previous state"=w663, "Loading Bar Display"=w659, "error in (no error)"=w665, "Open?"=w660, "Previous control access state"=w661, "ControlsIndicators in"=w658) -> ("error out"=w664:errorcluster, "Previous state"=w662:string, "ControlsIndicators out"=w657:T12)  [unwired: 3 in]
              n285 = in-place-cluster #4("AdditionalFeatures.PageHandling.Previous control access state"=w661, "AdditionalFeatures.Popup.Popup data.Loading bar data.Open?"=w660, "AdditionalFeatures.Popup.Popup data.Loading bar data.Display string"=w659, "AdditionalFeatures.Popup.Restore main tab"=w662, "ControlsIndicators"=w657) -> (w651:T38)
            }
            n286 = call <vilib>:"Add State(s) to Queue__JKI_lib_State_Machine.vi"("State(s) in (\"\")"=w656) -> ("States Out"=w655:string)  [unwired: 14 in]
          }
          frame "UI controls access" {
            # "Your code here.\n(You can make a copy of, or modify, this frame)"
            n287 = Unbundle By Name(w669) -> ("ControlsIndicators"=w667:T12)
            n288 = call "Segregate parameters.vi"("Input statement"=w670, "Number of parameters"=2) -> ("Parameter values array"=w673:string[])  [unwired: 9 in]
            n289 = Index Array(array=w673) -> (element #1=w671:string, element #2=w672:string)  [unwired: 2 in]
            n290 = Bundle By Name(cluster=w669, "AdditionalFeatures.PageHandling.Previous control access state"=w670) -> (w668:T38)
            n291 = call "UI controls access.vi"("error in (no error)"=w675, "Sub UI state"=w672, "Main UI State"=w671, "Controls and Indicators\nReferences"=w667) -> ("error out"=w676:errorcluster)  [unwired: 7 in]
            n292 = call <vilib>:"Add State(s) to Queue__JKI_lib_State_Machine.vi"("State(s) in (\"\")"=w677) -> ("States Out"=w678:string)  [unwired: 14 in]
          }
          frame "DisplayInspectionPage" {
            # "Template Separator\n(You can make a copy of, or modify, this frame)"
            n293 = case shown="\"Images\"" w679 {
              tunnel: [w705 w714] -> w685
              tunnel: w684 -> [w691 w715]
              tunnel: w682 -> [w688 w716]
              frame "NoOperation", "Reset", Default {
                n294 = Unbundle By Name(w688) -> ("ControlsIndicators.Inspection.Settings_Inspection"=w692:refnum<vi>, "ControlsIndicators.General.Command tab"=w697:refnum<vi>, "ControlsIndicators.Master sample.Master sample tab"=w696:refnum<vi>, "ControlsIndicators.Diagnostics.Current Diagnostics Status"=w710:refnum<vi>, "ControlsIndicators.General.Main Tab"=w709:refnum<vi>, "ControlsIndicators.General.Right Pane Tab"=w707:refnum<vi>, "ControlsIndicators.General.Inspection subTab control ref"=w701:refnum<vi>)
                n295 = property class="TabCtl (strict)"(reference=w697, error in=w691, "Value"=T5."Inspection") -> (error out=w695:errorcluster)  [unwired: 1 out]
                n296 = property class="TabCtl (strict)"(reference=w696, error in=w691, "Value"=enum32{"Master sample", "Inspection"}."Inspection") -> (error out=w694:errorcluster)  [unwired: 1 out]
                n297 = property class="TabCtl (strict)"(reference=w709, error in=w691, "Value"=T1."Blank") -> (error out=w704:errorcluster)  [unwired: 1 out]
                n298 = property class="ColBox"(reference=w710, error in=w691, "Value"=u32 11776947) -> (error out=w706:errorcluster)  [unwired: 1 out]
                n299 = property class="TabCtl (strict)"(reference=w707, error in=w691, "Value"=T8."Inspection") -> (error out=w703:errorcluster)  [unwired: 1 out]
                n300 = property class="TabCtl (strict)"(reference=w701, error in=w691, "Value"=enum32{"EventReason"}."EventReason") -> (error out=w700:errorcluster)  [unwired: 1 out]
                n301 = property class="Bool (strict)"(reference=w692, error in=w691, "Visible"=TRUE) -> (error out=w689:errorcluster)  [unwired: 1 out]
                n302 = Merge Errors(w689, w695, w694, w704, w706, w703, w700) -> (w705:errorcluster)
              }
              frame "Images" {
                n303 = Unbundle By Name(w716) -> ("ControlsIndicators.General.Main Tab"=w713:refnum<vi>)
                n304 = property class="TabCtl (strict)"(reference=w713, error in=w715, "Value"=T1."Run") -> (error out=w714:errorcluster)  [unwired: 1 out]
              }
            }
            n305 = case shown="\"Images\"" w679 {
              tunnel: ["UI controls access>>[Inspection,Select]" ("State(s) in Front (\"\")") "" "UI controls access>>[Inspection,Reset]" ("State(s) in Front (\"\")")] -> w680
              frame "NoOperation", Default {
              }
              frame "Images" {
              }
              frame "Reset" {
              }
            }
            n306 = call <vilib>:"Add State(s) to Queue__JKI_lib_State_Machine.vi"("State(s) in Front (\"\")"=w680, "State(s) in (\"\")"=w687) -> ("States Out"=w686:string)  [unwired: 13 in]
            n307 = Bundle By Name(cluster=w682, "AdditionalFeatures.PageHandling.Current state"="Inspection") -> (w681:T38)
          }
          frame "UserAuthentication" {
            # "code modified (02-08-2018)\nuserauthentication"
            # "Your code here.\n(You can make a copy of, or modify, this frame)"
            n308 = Unbundle By Name(w727) -> ("ControlsIndicators.Inspection.Settings_Inspection"=w720:refnum<vi>, "AdditionalFeatures.PageHandling.Current state"=w731:string)
            n309 = call <vilib>:"Application Directory.vi"() -> ("Application Directory"=w730:path)
            n310 = Build Path(base path=w730, name or relative path="Configuration file\\user_database.csv") -> (appended path=w733:path)
            n311 = call "User Authentication.vi"("error in"=w735, "file path"=w733) -> ("error out"=w724:errorcluster, "USER EXISTS?"=w729:bool, "Exit button pressed"=w725:bool, "Authentication message"=w728:string)  [unwired: 5 in, 1 out]
            n312 = case shown="\"settings\"" w731 {
              tunnel: ["Idle" w754] -> w732
              tunnel: w729 -> [_ w753]
              tunnel: w726 -> [w750 _]
              tunnel: w724 -> [w743 w752]
              tunnel: [w748 w752] -> w723
              tunnel: w728 -> [w745 _]
              frame "False", Default {
                # "code modified (08-08-2018)"
                n313 = Bundle By Name(cluster=T25 {"Acknowledgement_SM"={"Enqueuer"=refnum, "VIReference"=refnum, "VIName"=""}, "Button name"="", "PartDetails"={"PartName"="", "ConnectorsInReel"=0, "TotalCounts"=0, "OperatorName"="", "StampingMachineID"=0}, "SensorName"="", "CameraName"="", "PopupFeedbackDetails"={"Pop-up Type"=enum."Open Logo Display", "Message"="", "Pressed Button"=""}, "EventResponse"="", "ErrorMessage"="", "FailCountIgnore"={"ReelIgnoreCount"=0, "ProductionIgnoreCount"=0}} ("OutputDetails"), "PopupFeedbackDetails.Message"=w745) -> (w746:T25)
                n314 = call "Output_UI.vi"("OutputDetails"=w746, "error in"=w743, "Functionality"=Output_choice."SendPopupResponse", "Testbench"=TRUE, "SMEnqueuer"=w750) -> ("error out"=w748:errorcluster)  [unwired: 6 in]
              }
              frame "settings" {
                n315 = case shown="True" w753 {
                  tunnel: "DisplaySettingsOptions" -> [w757 w761]
                  tunnel: [w756 w759] -> w754
                  frame False {
                    # "user doesn't exist"
                    n316 = Concatenate Strings(w757, ">>user doesn't exist" ("string")) -> (w756:string)
                  }
                  frame True {
                    # "User exists"
                    n317 = Concatenate Strings(w761, ">>user exists" ("string")) -> (w759:string)
                  }
                }
              }
            }
            n318 = case shown="True" w725 {
              tunnel: w724 -> [w738 w742]
              tunnel: [w738 w741] -> w721
              tunnel: w720 -> [_ w740]
              frame False {
              }
              frame True {
                n319 = property class="Bool (strict)"(reference=w740, error in=w742, "DisabledEnum"=T28."Enabled" ("Disabled")) -> (error out=w741:errorcluster)  [unwired: 1 out]
              }
            }
            n320 = Merge Errors(w721, w723) -> (w722:errorcluster)
            n321 = call <vilib>:"Add State(s) to Queue__JKI_lib_State_Machine.vi"("State(s) in Front (\"\")"=w732, "State(s) in (\"\")"=w736) -> ("States Out"=w737:string)  [unwired: 13 in]
          }
          frame "Display CpCpk popup" {
            # "Template Separator\n(You can make a copy of, or modify, this frame)"
            n322 = Unbundle By Name(w763) -> ("ButtonPress_UI"=w762:refnum<user-event>)
            n323 = in-place {
              in-place-border: w767 -> [w775]
              in-place-border: [w774] -> w766
              in-place-border: w762 -> [w770]
              n324 = in-place-cluster #5(w765) -> ("AdditionalFeatures.Cp Cpk details.CpCpkData"=w773:string[][], "Inspection.MeasurementNames"=w772:string[])  [unwired: 1 out]
              n325 = call "Cp-Cpk Popup.vi"("error in"=w775, "ButtonPress_UI"=w770, "Measurement Names"=w772, "Cp-Cpk Popup input"=w773) -> ("error out"=w774:errorcluster, "Cp Cpk Popup VI reference"=w771:refnum<vi>)  [unwired: 6 in]
              n326 = in-place-cluster #5("AdditionalFeatures.Cp Cpk details.CpCpkData"=w773, "Inspection.MeasurementNames"=w772, "AdditionalFeatures.Cp Cpk details.Cp Cpk popup"=w771) -> (w764:T38)
            }
            n327 = call <vilib>:"Add State(s) to Queue__JKI_lib_State_Machine.vi"("State(s) in (\"\")"=w769) -> ("States Out"=w768:string)  [unwired: 14 in]
          }
          frame "Display zentron stratuplogo" {
            n328 = case shown="\"False\", Default" w777 {
              tunnel: ["" "UI: Front Panel State>>Open" ("State(s) in Front (\"\")")] -> w776
              frame "False", Default {
              }
              frame "close" {
              }
            }
            n329 = call "Manual open close init image.vi"("error in (no error)"=w780, "Function\ncommand"=w777) -> ("error out"=w779:errorcluster)  [unwired: 9 in]
            n330 = call <vilib>:"Add State(s) to Queue__JKI_lib_State_Machine.vi"("State(s) in Front (\"\")"=w776, "State(s) in (\"\")"=w781) -> ("States Out"=w782:string)  [unwired: 13 in]
          }
          frame "DisplayEventReason" {
            # "code modified (01-10-2018)"
            n331 = case shown="\"Fail\"" w798 {
              tunnel: w795 -> [w802 w804 w806]
              tunnel: [w801 w803 w805] -> w797
              frame "Pause", Default {
                n332 = Unbundle By Name(w802) -> ("JSONRead.ConfigurationCluster.UIParameters.EventReasonsList.Pause"=w801:string[])
              }
              frame "Fail" {
                n333 = Unbundle By Name(w804) -> ("Inspection.Fail event reason list"=w803:string[])
              }
              frame "Stop" {
                n334 = Unbundle By Name(w806) -> ("JSONRead.ConfigurationCluster.UIParameters.EventReasonsList.Stop"=w805:string[])
              }
            }
            n335 = Unbundle By Name(w795) -> ("ControlsIndicators.General.Event  Reason  List"=w796:refnum<vi>, "ControlsIndicators.General.Event reason switching tab"=w791:refnum<vi>, "ControlsIndicators.General.Event reason blink"=w790:refnum<vi>)
            n336 = property class="TabCtl (strict)"(reference=w791, error in=w788, "Value"=enum32{"EventReason", "InspectionButtons"}."EventReason") -> (error out=w794:errorcluster)  [unwired: 1 out]
            n337 = property class="CmbBox"(reference=w796, error in=w788, "Strings[]"=w797, "Text.Text"="Select an event\nreason") -> (error out=w793:errorcluster)  [unwired: 1 out]
            n338 = property class="Str"(reference=w790, error in=w788, "Blinking"=TRUE) -> (error out=w787:errorcluster)  [unwired: 1 out]
            n339 = call <vilib>:"Add State(s) to Queue__JKI_lib_State_Machine.vi"("State(s) in (\"\")"=w799) -> ("States Out"=w800:string)  [unwired: 14 in]
            n340 = Merge Errors(w794, w793, w787) -> (w792:errorcluster)
          }
          frame "---------- Initialization ----------" {
            # "Your code here.\n(You can make a copy of, or modify, this frame)"
            n341 = call <vilib>:"Add State(s) to Queue__JKI_lib_State_Machine.vi"("State(s) in (\"\")"=w809) -> ("States Out"=w810:string)  [unwired: 14 in]
          }
          frame "Update user screen interaction loop" {
            # "Your code here.\n(You can make a copy of, or modify, this frame)"
            n342 = Unbundle By Name(w814) -> ("SendClusterData"=w813:refnum<user-event>)
            n343 = Generate User Event(priority (normal)=usereventprio."high priority", user event=w813, event data cluster=w812, error in=w816) -> (error out=w815:errorcluster)  [unwired: 1 out]
            n344 = call <vilib>:"Add State(s) to Queue__JKI_lib_State_Machine.vi"("State(s) in (\"\")"=w817) -> ("States Out"=w818:string)  [unwired: 14 in]
          }
          frame "Send acknowledge" {
            # "Testbench_label"
            # "Output.vi_code modified(02-08-2018)"
            n345 = Unbundle By Name(w821) -> ("AdditionalFeatures.Core.Current VI Reference"=w825:refnum<vi>)
            n346 = Bundle By Name(cluster=T25 {"Acknowledgement_SM"={"Enqueuer"=refnum, "VIReference"=refnum, "VIName"=""}, "Button name"="", "PartDetails"={"PartName"="", "ConnectorsInReel"=0, "TotalCounts"=0, "OperatorName"="", "StampingMachineID"=0}, "SensorName"="", "CameraName"="", "PopupFeedbackDetails"={"Pop-up Type"=enum."Open Logo Display", "Message"="", "Pressed Button"=""}, "EventResponse"="", "ErrorMessage"="", "FailCountIgnore"={"ReelIgnoreCount"=0, "ProductionIgnoreCount"=0}} ("OutputDetails"), "Acknowledgement_SM.Enqueuer"=w820, "Acknowledgement_SM.VIReference"=w825) -> (w824:T25)
            n347 = call <vilib>:"Add State(s) to Queue__JKI_lib_State_Machine.vi"("State(s) in (\"\")"=w829) -> ("States Out"=w830:string)  [unwired: 14 in]
            n348 = call "Output_UI.vi"("OutputDetails"=w824, "error in"=w828, "Functionality"=Output_choice."SendAcknowledgement", "Testbench"=TRUE, "SMEnqueuer"=w819) -> ("error out"=w827:errorcluster)  [unwired: 6 in]
          }
          frame "Init images and labels" {
            n349 = Unbundle By Name(w836) -> ("ControlsIndicators"=w835:T12, "JSONRead"=w834:T39)
            n350 = control-ref of="SensorDiagnosticsImage"() -> (w831:refnum<vi>)
            n351 = control-ref of="TL"() -> (w838:refnum<vi>)
            n352 = Bundle By Name(cluster=T30 {"Image refnum"=refnum, "Label refnum"=refnum} ("References"), "Image refnum"=w831, "Label refnum"=w838) -> (w837:T30)
            n353 = call "Init images and labels.vi"("error in (no error)"=w841, "JSON Read"=w834, "References"=w837, "ControlsIndicators"=w835) -> ("error out"=w840:errorcluster)  [unwired: 7 in]
            n354 = call <vilib>:"Add State(s) to Queue__JKI_lib_State_Machine.vi"("State(s) in (\"\")"=w833) -> ("States Out"=w832:string)  [unwired: 14 in]
          }
          frame "Read init JSON params" {
            n355 = Unbundle By Name(w843) -> ("JSONRead.ConfigurationFilePaths.Rack Controller Override JSON file path in"=w850:path, "JSONRead.ConfigurationFilePaths.Algorithm Overrride JSON file path in"=w849:path)
            n356 = call "Read Configuration Variant.vi"("error in"=w846, "JSON file path in"=w850) -> ("error out"=w851:errorcluster, "JSON variant out"=w847:variant)  [unwired: 8 in]
            n357 = call "Read Configuration Variant.vi"("error in"=w846, "JSON file path in"=w849) -> ("error out"=w845:errorcluster, "JSON variant out"=w848:variant)  [unwired: 8 in]
            n358 = Bundle By Name(cluster=w843, "JSONRead.ConfigurationVariants.Rack Controller Override\nJSON Variant"=w847, "JSONRead.ConfigurationVariants.Algorithm Override\nJSON Variant"=w848) -> (w842:T38)
            n359 = Merge Errors(w851, w845) -> (w844:errorcluster)
            n360 = call <vilib>:"Add State(s) to Queue__JKI_lib_State_Machine.vi"("State(s) in (\"\")"=w852) -> ("States Out"=w853:string)  [unwired: 14 in]
          }
          frame "Populate partslist" {
            w861 = "SELECT PART" ("Text.Text")
            n361 = Unbundle By Name(w862) -> ("ControlsIndicators.Edit Tolerance Limits.Select a part"=w854:refnum<vi>, "ControlsIndicators.General.SelectionCluster.PART NAME"=w855:refnum<vi>, "Inspection.parts List"=w860:string[])
            n362 = property class="CmbBox"(reference=w855, error in=w859, "Text.Text"=w861, "Strings[]"=w860) -> (error out=w857:errorcluster)  [unwired: 1 out]
            n363 = property class="CmbBox"(reference=w854, error in=w859, "Text.Text"=w861, "Strings[]"=w860) -> (error out=w858:errorcluster)  [unwired: 1 out]
            n364 = Merge Errors(w857, w858) -> (w856:errorcluster)
            n365 = call <vilib>:"Add State(s) to Queue__JKI_lib_State_Machine.vi"("State(s) in (\"\")"=w863) -> ("States Out"=w864:string)  [unwired: 14 in]
          }
          frame "Enable image label dropdown" {
            n366 = Unbundle By Name(w872) -> ("ControlsIndicators.Inspection.Label array"=w871:refnum<vi>[], "AdditionalFeatures.DynamicImageHandling.Enable DIH?"=w870:bool)
            n367 = Select(t=T28."Enabled" ("Disabled"), s=w870, f=T28."Disabled and Grayed Out" ("Disabled")) -> (s? t:f=w867:T28)
            n368 = for {
              tunnel: w871 -> [w878] mode=indexing
              tunnel: w867 -> [w877]
              shift-right: [w875] -> w865
              shift-left: w866 -> [w876]
              n369 = property class="CmbBox"(reference=w878, error in=w876, "DisabledEnum"=w877) -> (error out=w875:errorcluster)  [unwired: 1 out]
            }
            n370 = call <vilib>:"Add State(s) to Queue__JKI_lib_State_Machine.vi"("State(s) in (\"\")"=w874) -> ("States Out"=w873:string)  [unwired: 14 in]
          }
          frame "----------Diagnostics----------" {
            n371 = call <vilib>:"Add State(s) to Queue__JKI_lib_State_Machine.vi"("State(s) in (\"\")"=w882) -> ("States Out"=w881:string)  [unwired: 14 in]
          }
          frame "UpdateDiagnosticsStatusString" {
            # "modified(11.12.2018)"
            n372 = in-place {
              in-place-border: w888 -> [w894]
              in-place-border: [w893] -> w887
              in-place-border: w886 -> [w892]
              n373 = in-place-cluster #6(w885) -> ("ControlsIndicators.Diagnostics.Diagnostics Status\nString"=w891:refnum<vi>)
              n374 = property class="Str"(reference=w891, error in=w894, "Value"=w892) -> (error out=w893:errorcluster)  [unwired: 1 out]
              n375 = in-place-cluster #6("ControlsIndicators.Diagnostics.Diagnostics Status\nString"=w891) -> (w884:T38)
            }
            n376 = call <vilib>:"Add State(s) to Queue__JKI_lib_State_Machine.vi"("State(s) in (\"\")"=w890) -> ("States Out"=w889:string)  [unwired: 14 in]
          }
          frame "DisplayDiagnosticsPage" {
            n377 = Unbundle By Name(w931) -> ("ControlsIndicators.Diagnostics.Current Diagnostics Status"=w911:refnum<vi>, "ControlsIndicators.Diagnostics.Diagnostics Status"=w920:refnum<vi>, "ControlsIndicators.Diagnostics.Diagnostics Tab"=w930:refnum<vi>, "ControlsIndicators.General.Main Tab"=w929:refnum<vi>, "ControlsIndicators.Diagnostics.Logout_Diagnostics"=w928:refnum<vi>, "ControlsIndicators.General.Command tab"=w927:refnum<vi>, "ControlsIndicators.General.Right Pane Tab"=w926:refnum<vi>, "ControlsIndicators.Diagnostics.Select a diagnostics"=w908:refnum<vi>, "ControlsIndicators.Diagnostics.Select a sub diagnostics"=w906:refnum<vi>, "ControlsIndicators.Diagnostics.Logout_Diagnostics"=w903:refnum<vi>)
            n378 = property class="Bool (strict)"(reference=w903, error in=w902, "DisabledEnum"=T28."Enabled" ("Disabled"), "Visible"=TRUE) -> (error out=w901:errorcluster)  [unwired: 1 out]
            n379 = property class="TabCtl (strict)"(reference=w930, error in=w902, "Value"=T2."Arduino Motor") -> (error out=w917:errorcluster)  [unwired: 1 out]
            n380 = property class="TabCtl (strict)"(reference=w929, error in=w902, "Value"=T1."Diagnostics") -> (error out=w916:errorcluster)  [unwired: 1 out]
            n381 = property class="TabCtl (strict)"(reference=w927, error in=w902, "Value"=T5."Diagnostics") -> (error out=w912:errorcluster)  [unwired: 1 out]
            n382 = property class="TabCtl (strict)"(reference=w926, error in=w902, "Value"=T8."Diagnostics") -> (error out=w915:errorcluster)  [unwired: 1 out]
            n383 = property class="CmbBox"(reference=w908, error in=w902, "DisabledEnum"=T28."Enabled" ("Disabled"), "Value"="Select diagnostics") -> (error out=w907:errorcluster)  [unwired: 1 out]
            n384 = property class="CmbBox"(reference=w906, error in=w902, "Visible"=FALSE) -> (error out=w905:errorcluster)  [unwired: 1 out]
            n385 = property class="Bool (strict)"(reference=w928, error in=w902, "DisabledEnum"=T28."Enabled" ("Disabled")) -> (error out=w913:errorcluster)  [unwired: 1 out]
            n386 = property class="ColBox"(reference=w911, error in=w902, "Value"=u32 12829635) -> (error out=w919:errorcluster)  [unwired: 1 out]
            n387 = property class="Str"(reference=w920, error in=w902, "Value"="No diagnostics\nselected") -> (error out=w918:errorcluster)  [unwired: 1 out]
            n388 = call <vilib>:"Add State(s) to Queue__JKI_lib_State_Machine.vi"("State(s) in Front (\"\")"="Populate diagnostics list" ("State(s) in Front (\"\")"), "State(s) in (\"\")"=w933) -> ("States Out"=w932:string)  [unwired: 13 in]
            n389 = Merge Errors(w919, w918, w917, w916, w913, w912, w915, w907, w905, w901) -> (w914:errorcluster)
          }
          frame "Run" {
            n390 = Unbundle By Name(w934) -> ("AdditionalFeatures.PageHandling.Current state"=w937:string)
            n391 = case shown="\"inspection\", Default" w937 {
              tunnel: w936 -> [w940 w944]
              tunnel: [w940 w943] -> w935
              tunnel: w934 -> [_ w941]
              frame "inspection", Default {
              }
              frame "diagnostics" {
                n392 = Unbundle By Name(w941) -> ("ControlsIndicators.Diagnostics.RUN"=w945:refnum<vi>)
                n393 = property class="ColBox"(reference=w945, error in=w944, "Value"=u32 8978365 ("Color Box")) -> (error out=w943:errorcluster)  [unwired: 1 out]
              }
            }
            n394 = call <vilib>:"Add State(s) to Queue__JKI_lib_State_Machine.vi"("State(s) in (\"\")"=w939) -> ("States Out"=w938:string)  [unwired: 14 in]
          }
          frame "BuzzerOff" {
            n395 = Unbundle By Name(w946) -> ("AdditionalFeatures.PageHandling.Current state"=w949:string)
            n396 = case shown="\"inspection\", Default" w949 {
              tunnel: w946 -> [_ w957]
              tunnel: w948 -> [w952 w955]
              tunnel: [w952 w954] -> w947
              frame "inspection", Default {
              }
              frame "diagnostics" {
                n397 = Unbundle By Name(w957) -> ("ControlsIndicators.Diagnostics.BUZZER OFF"=w956:refnum<vi>)
                n398 = property class="ColBox"(reference=w956, error in=w955, "Value"=u32 8978365 ("Color Box")) -> (error out=w954:errorcluster)  [unwired: 1 out]
              }
            }
            n399 = call <vilib>:"Add State(s) to Queue__JKI_lib_State_Machine.vi"("State(s) in (\"\")"=w951) -> ("States Out"=w950:string)  [unwired: 14 in]
          }
          frame "DiagnosticsFail", "DiagnosticsPass" {
            n400 = Unbundle By Name(w966) -> ("ControlsIndicators.Diagnostics"=w972:T15, "AdditionalFeatures.PageHandling.Current state"=w962:string)
            n401 = Equal?(x=w969, y="DiagnosticsPass") -> (x = y?=w967:bool)
            n402 = Select(t=u32 8978330, s=w967, f=u32 16711680) -> (s? t:f=w958:u32)
            n403 = Unbundle By Name(w972) -> ("Select a diagnostics"=w965:refnum<vi>, "Current Diagnostics Status"=w959:refnum<vi>, "Logout_Diagnostics"=w963:refnum<vi>)
            n404 = property class="ColBox"(reference=w959, error in=w961, "Value"=w958) -> (error out=w960:errorcluster)  [unwired: 1 out]
            n405 = case shown="\"diagnostics\"" w962 {
              tunnel: w965 -> [_ w983]
              tunnel: [w975 w980] -> w964
              tunnel: w960 -> [w975 w976]
              tunnel: w963 -> [_ w979]
              frame "POST", Default {
              }
              frame "diagnostics" {
                n406 = property class="Bool (strict)"(reference=w979, error in=w976, "DisabledEnum"=T28."Enabled" ("Disabled")) -> (error out=w977:errorcluster)  [unwired: 1 out]
                n407 = property class="CmbBox"(reference=w983, error in=w976, "DisabledEnum"=T28."Enabled" ("Disabled")) -> (error out=w981:errorcluster)  [unwired: 1 out]
                n408 = Merge Errors(w981, w977) -> (w980:errorcluster)
              }
            }
            n409 = call <vilib>:"Add State(s) to Queue__JKI_lib_State_Machine.vi"("State(s) in (\"\")"=w974) -> ("States Out"=w973:string)  [unwired: 14 in]
          }
          frame "Populate diagnostics list" {
            n410 = Unbundle By Name(w986) -> ("Diagnostics"=w985:T42, "ControlsIndicators.Diagnostics.Select a diagnostics"=w984:refnum<vi>)
            n411 = call "Popuplate diagnostics selecction.vi"("error in (no error)"=w988, "MainDiagnostics"=w984, "Diagnostics in"=w985) -> ("error out"=w987:errorcluster)  [unwired: 8 in]
            n412 = call <vilib>:"Add State(s) to Queue__JKI_lib_State_Machine.vi"("State(s) in (\"\")"=w990) -> ("States Out"=w989:string)  [unwired: 14 in]
          }
          frame "----------Analytics----------" {
            n413 = call <vilib>:"Add State(s) to Queue__JKI_lib_State_Machine.vi"("State(s) in (\"\")"=w994) -> ("States Out"=w993:string)  [unwired: 14 in]
          }
          frame "DisplayAnalyticsGraphs" {
            # "code modified (08-08-2018)\nanalytics"
            n414 = Unbundle By Name(w1001) -> ("ControlsIndicators.Inspection.Analytics_Inspection"=w998:refnum<vi>, "ControlsIndicators.General.Main Tab"=w1003:refnum<vi>)
            n415 = property class="TabCtl (strict)"(reference=w1003, error in=w999, "Value"=T1."Analytics") -> (error out=w997:errorcluster)  [unwired: 1 out]
            n416 = property class="Bool (strict)"(reference=w998, error in=w999, "Value"=TRUE) -> (error out=w995:errorcluster)  [unwired: 1 out]
            n417 = Merge Errors(w995, w997) -> (w996:errorcluster)
            n418 = call <vilib>:"Add State(s) to Queue__JKI_lib_State_Machine.vi"("State(s) in (\"\")"=w1005) -> ("States Out"=w1004:string)  [unwired: 14 in]
          }
          frame "DisplayImages" {
            # "code modified (08-08-2018)\nanalytics"
            n419 = Unbundle By Name(w1013) -> ("ControlsIndicators.Inspection.Analytics_Inspection"=w1010:refnum<vi>, "ControlsIndicators.General.Main Tab"=w1011:refnum<vi>)
            n420 = property class="TabCtl (strict)"(reference=w1011, error in=w1012, "Value"=T1."Run") -> (error out=w1008:errorcluster)  [unwired: 1 out]
            n421 = property class="Bool (strict)"(reference=w1010, error in=w1012, "Value"=FALSE) -> (error out=w1007:errorcluster)  [unwired: 1 out]
            n422 = Merge Errors(w1007, w1008) -> (w1006:errorcluster)
            n423 = call <vilib>:"Add State(s) to Queue__JKI_lib_State_Machine.vi"("State(s) in (\"\")"=w1016) -> ("States Out"=w1015:string)  [unwired: 14 in]
          }
          frame "----------Part Select----------" {
            n424 = call <vilib>:"Add State(s) to Queue__JKI_lib_State_Machine.vi"("State(s) in (\"\")"=w1020) -> ("States Out"=w1019:string)  [unwired: 14 in]
          }
          frame "Part selection" {
            # "code modified (31-07-2018)\nCountUpdate"
            n425 = Unbundle By Name(w1036) -> ("ControlsIndicators.General.SelectionCluster"=w1025:T18, "ControlsIndicators.General.Event  Reason  List"=w1033:refnum<vi>, "ControlsIndicators"=w1037:T12)
            n426 = Unbundle By Name(w1037) -> ("General.SelectionCluster.PART NAME"=w1048:refnum<vi>, "General.SelectionCluster.VERIFIED"=w1047:refnum<vi>, "General.SelectionCluster.change"=w1046:refnum<vi>, "General.SelectionCluster.confirm"=w1045:refnum<vi>, "General.SelectionCluster.ok"=w1044:refnum<vi>, "General.SelectionCluster.reset"=w1043:refnum<vi>, "General.SelectionCluster.TOTAL COUNT"=w1042:refnum<vi>, "General.SelectionCluster.REEL COUNT"=w1041:refnum<vi>, "General.SelectionCluster.OPERATOR NAME"=w1049:refnum<vi>, "General.SelectionCluster.Select message"=w1024:refnum<vi>, "Inspection.Run_Inspection"=w1022:refnum<vi>)
            n427 = Bundle By Name(cluster=T32 {"Selection cluster"={"ok"=refnum, "confirm"=refnum, "reset"=refnum, "change"=refnum, "TOTAL COUNT"=refnum, "REEL COUNT"=refnum, "PART NAME"=refnum, "VERIFIED"=refnum, "OPERATOR NAME"=refnum, "Select message"=refnum}, "Event  Reason  List"=refnum} ("Select control references"), "Selection cluster"=w1025, "Event  Reason  List"=w1033) -> (w1026:T32)
            n428 = Bundle By Name(cluster=T31 {"Part Name"=refnum, "Verification"=refnum, "Change"=refnum, "Confirm"=refnum, "OK Button"=refnum, "Reset Button"=refnum, "Total count"=refnum, "Reel count"=refnum, "Operator ID"=refnum, "Select message"=refnum, "Inspection Run"=refnum} ("Reference Cluster"), "Part Name"=w1048, "Verification"=w1047, "Change"=w1046, "Confirm"=w1045, "OK Button"=w1044, "Reset Button"=w1043, "Total count"=w1042, "Reel count"=w1041, "Operator ID"=w1049, "Select message"=w1024, "Inspection Run"=w1022) -> (w1021:T31)
            n429 = call "Select.vi"("error in (no error)"=w1050, "State"=w1028, "Reference Cluster"=w1021) -> ("error out"=w1031:errorcluster, "Count error?"=w1032:bool, "Confirmed?"=w1038:bool)  [unwired: 6 in]
            n430 = case shown="True" w1038 {
              tunnel: w1031 -> [w1059 w1074]
              tunnel: [w1059 w1070] -> w1039
              tunnel: w1034 -> [_ w1068]
              tunnel: w1036 -> [w1058 w1073]
              tunnel: [w1058 w1061] -> w1035
              tunnel: w1026 -> [_ w1060]
              frame False {
              }
              frame True {
                # "Output.vi_code modified (02-08-2018)"
                n431 = call "Select message creator.vi"("error in (no error)"=w1074, "Select control references"=w1060) -> ("error out"=w1069:errorcluster, "PartDetails"=w1065:T64)  [unwired: 8 in]
                n432 = Unbundle By Name(w1065) -> ("ConnectorsInReel"=w1072:u64, "TotalCounts"=w1071:u64)
                n433 = Bundle By Name(cluster=T25 {"Acknowledgement_SM"={"Enqueuer"=refnum, "VIReference"=refnum, "VIName"=""}, "Button name"="", "PartDetails"={"PartName"="", "ConnectorsInReel"=0, "TotalCounts"=0, "OperatorName"="", "StampingMachineID"=0}, "SensorName"="", "CameraName"="", "PopupFeedbackDetails"={"Pop-up Type"=enum."Open Logo Display", "Message"="", "Pressed Button"=""}, "EventResponse"="", "ErrorMessage"="", "FailCountIgnore"={"ReelIgnoreCount"=0, "ProductionIgnoreCount"=0}} ("OutputDetails"), "PartDetails"=w1065) -> (w1064:T25)
                n434 = call "Output_UI.vi"("OutputDetails"=w1064, "error in"=w1069, "Functionality"=Output_choice."SendPartDetails", "Testbench"=TRUE, "SMEnqueuer"=w1068) -> ("error out"=w1070:errorcluster)  [unwired: 6 in]
                n435 = Bundle By Name(cluster=w1073, "Diagnostics.Selection Done?"=TRUE, "Inspection.Max limits.Production max"=w1072, "Inspection.Max limits.Reel max"=w1071) -> (w1061:T38)
              }
            }
            n436 = case shown="\"Button press\", Default" w1028 {
              tunnel: w1032 -> [_ w1055]
              tunnel: w1030 -> [_ w1054]
              tunnel: ["" w1053] -> w1029
              frame "Button press", Default {
              }
              frame "OK" {
                n437 = case shown="False" w1055 {
                  tunnel: w1054 -> [_ _]
                  tunnel: ["Part selection>>Confirm" ("FunctionalityName") "Part selection>>Enable selection" ("FunctionalityName")] -> w1053
                  frame False {
                  }
                  frame True {
                  }
                }
              }
            }
            n438 = call <vilib>:"Add State(s) to Queue__JKI_lib_State_Machine.vi"("State(s) in Front (\"\")"=w1029, "State(s) in (\"\")"=w1040) -> ("States Out"=w1051:string)  [unwired: 13 in]
          }
          frame "Read Algo and RC override JSON" {
            n439 = Unbundle By Name(w1078) -> ("EditToleranceSettings.IsPartSelected"=w1077:bool)
            n440 = Bundle By Name(cluster=w1078, "AdditionalFeatures.Popup.Popup data.Loading bar data.Open?"=TRUE ("Display fail image?"), "AdditionalFeatures.Popup.Popup data.Loading bar data.Display string"="Loading...Please Wait..." ("Loading bar data.Display string")) -> (w1076:T38)
            n441 = case shown="False" w1077 {
              tunnel: ["Display loading bar\nRead ET parameters\nUpdate user screen interaction loop\nDisplay loading bar" ("State(s) in Front (\"\")") "Read ET parameters\nUpdate user screen interaction loop" ("State(s) in Front (\"\")")] -> w1079
              tunnel: w1076 -> [w1085 w1089]
              tunnel: [w1085 w1088] -> w1075
              frame False {
              }
              frame True {
                n442 = Bundle By Name(cluster=w1089, "EditToleranceSettings.IsPartSelected"=FALSE ("Part select?")) -> (w1088:T38)
              }
            }
            n443 = call <vilib>:"Add State(s) to Queue__JKI_lib_State_Machine.vi"("State(s) in Front (\"\")"=w1079, "State(s) in (\"\")"=w1082) -> ("States Out"=w1084:string)  [unwired: 13 in]
          }
          frame "Read ET parameters" {
            n444 = in-place {
              in-place-border: [w1107] -> w1092
              in-place-border: w1095 -> [w1105]
              n445 = in-place-cluster #7(w1094) -> ("JSONRead"=w1099:T39, "ControlsIndicators.Edit Tolerance Limits.Tolerance Limits Listbox"=w1100:refnum<vi>, "EditToleranceSettings"=w1103:T43, "ControlsIndicators.Edit Tolerance Limits.Select a part"=w1102:refnum<vi>)  [unwired: 1 out]
              n446 = property class="CmbBox"(reference=w1102, error in=w1105) -> (error out=w1104:errorcluster, "Text.Text"=w1106:string)  [unwired: 1 out]
              n447 = call "Read tolerance limits params.vi"("JSON Read"=w1099, "error in (no error)"=w1104, "MeasurementListBox"=w1100, "Part Name"=w1106, "Edit Tolerance Settings Cluster"=w1103) -> ("error out"=w1107:errorcluster, "Edit Tolerance Settings Cluster 2"=w1098:T43)  [unwired: 4 in, 1 out]
              n448 = in-place-cluster #7("JSONRead"=w1099, "ControlsIndicators.Edit Tolerance Limits.Tolerance Limits Listbox"=w1100, "AdditionalFeatures.Popup.Popup data.Loading bar data.Open?"=FALSE, "EditToleranceSettings"=w1098, "ControlsIndicators.Edit Tolerance Limits.Select a part"=w1102) -> (w1093:T38)
            }
            n449 = call <vilib>:"Add State(s) to Queue__JKI_lib_State_Machine.vi"("State(s) in (\"\")"=w1096) -> ("States Out"=w1097:string)  [unwired: 14 in]
            n450 = call <vilib>:"Clear Errors.vi"("error in (no error)"=w1092) -> ("error out"=w1091:errorcluster)  [unwired: 5 in, 1 out]
          }
          frame "---------- Inspection ----------" {
            n451 = call <vilib>:"Add State(s) to Queue__JKI_lib_State_Machine.vi"("State(s) in (\"\")"=w1110) -> ("States Out"=w1111:string)  [unwired: 14 in]
          }
          frame "UpdateFailIgnoreCounts" {
            n452 = in-place {
              n453 = in-place-cluster #8(w1113) -> ("AdditionalFeatures.Fail Ignore Count Reversal.Production ignored count"=w1118:u64, "AdditionalFeatures.Fail Ignore Count Reversal.Reel ignored count"=w1117:u64)
              "Reel Fail Ignore Count" <- w1117
              "Production Fail Ignore Count" <- w1118
              n454 = in-place-cluster #8("AdditionalFeatures.Fail Ignore Count Reversal.Production ignored count"=w1118, "AdditionalFeatures.Fail Ignore Count Reversal.Reel ignored count"=w1117) -> (w1112:T38)
            }
            n455 = call <vilib>:"Add State(s) to Queue__JKI_lib_State_Machine.vi"("State(s) in (\"\")"=w1115) -> ("States Out"=w1116:string)  [unwired: 14 in]
          }
          frame "Complete" {
            n456 = case shown="\"Production\"" w1119 {
              tunnel: w1121 -> [w1126 w1131]
              tunnel: [w1127 w1130] -> w1120
              frame "Production" {
                w1125 = u64 0 ("AdditionalFeatures.Master sample validation.Reel ignored count")
                n457 = Bundle By Name(cluster=w1126, "Inspection.Reel complete"=TRUE, "AdditionalFeatures.Fail Ignore Count Reversal.Reel ignored count"=w1125, "AdditionalFeatures.Fail Ignore Count Reversal.Production ignored count"=w1125) -> (w1127:T38)
              }
              frame "Reel", Default {
                n458 = Bundle By Name(cluster=w1131, "Inspection.Reel complete"=TRUE, "AdditionalFeatures.Fail Ignore Count Reversal.Reel ignored count"=u64 0 ("AdditionalFeatures.Master sample validation.Reel ignored count")) -> (w1130:T38)
              }
            }
            n459 = call <vilib>:"Add State(s) to Queue__JKI_lib_State_Machine.vi"("State(s) in (\"\")"=w1123) -> ("States Out"=w1124:string)  [unwired: 14 in]
          }
          frame "Flush event queue" {
            n460 = Flush Event Queue(0:w1135, 3:w1137, 5:3 ("keep most recent")) -> (11:w1136:errorcluster)  [unwired: 3 in, 2 out]
            n461 = call <vilib>:"Add State(s) to Queue__JKI_lib_State_Machine.vi"("State(s) in (\"\")"=w1138) -> ("States Out"=w1139:string)  [unwired: 14 in]
          }
          frame "ReadyToInsert" {
            w1168 = u16 0 items=["Combo", "String"] ("Type of label")
            # "modified (11.12.2018)"
            # "code modified (31-07-2018)\nappended array removed\nString label removed"
            n462 = Unbundle By Name(w1161) -> ("AdditionalFeatures.PageHandling.Current state"=w1154:string, "JSONRead.ConfigurationCluster.UIParameters.ImageIndicatorLayouts"=w1176:T7, "ControlsIndicators.General.Image Reference array"=w1180:refnum<vi>[], "ControlsIndicators.Inspection.Label array"=w1179:refnum<vi>[], "ControlsIndicators.General.Main Tab"=w1178:refnum<vi>, "JSONRead.ConfigurationCluster.UIParameters.CameraLabelMapping"=w1174:T65, "ControlsIndicators.Diagnostics.Diagnostics Tab"=w1169:refnum<vi>)
            n463 = Unbundle By Name(w1161) -> ("ControlsIndicators.Inspection.Pass-Fail Indicator String"=w1145:refnum<vi>, "ControlsIndicators.Inspection.Inspection Status"=w1149:refnum<vi>, "ControlsIndicators.Inspection.Cards array"=w1153:refnum<vi>, "Inspection.Image details_init"=w1160:T57, "ControlsIndicators.Inspection.Counts"=w1164:refnum<vi>, "Inspection.Max limits.Reel max"=w1166:u64, "Inspection.Max limits.Production max"=w1165:u64)
            n464 = Unbundle By Name(w1155) -> ("Enable shortkey"=w1157:refnum<user-event>)
            n465 = case shown="\"Inspection\", Default" w1154 {
              tunnel: ["UI controls access>>[Inspection,Ready to insert]\nPart selection>>EnableChange" ("State(s) in Front (\"\")") ""] -> w1177
              frame "Inspection", Default {
              }
              frame "Master sample", "diagnostics" {
              }
            }
            n466 = Generate User Event(user event=w1157, event data cluster=TRUE ("event data"), error in=w1156) -> (error out=w1147:errorcluster)  [unwired: 1 in, 1 out]
            n467 = call "Create RBCIA.vi"("Camera image mapping"=w1174, "Inspection.Image details_init"=w1160) -> ("RBCIA (Rack based camera image indicator mapping) out"=w1172:cluster{"Rack Id":u8, "Label names":string[]}[])  [unwired: 9 in]
            n468 = call "Initialize dynamic image handling.vi"("Camera label mapping"=w1174, "Inspection.Image details_init"=w1160) -> ("ISIM"=w1175:u8[], "Combined camera names"=w1171:string[], "Image indicator labels"=w1173:string[])  [unwired: 7 in]
            n469 = property class="Arr (strict)"(reference=w1153, error in=w1147, "Value"=T9 []) -> (error out=w1150:errorcluster)  [unwired: 1 out]
            n470 = property class="ColBox"(reference=w1149, error in=w1147, "DisabledEnum"=T28."Enabled" ("Disabled")) -> (error out=w1146:errorcluster)  [unwired: 1 out]
            n471 = call "Set count lmits.vi"("error in (no error)"=w1147, "Production max limit"=w1165, "Reel max limit"=w1166, "Counts"=w1164) -> ("error out"=w1151:errorcluster)  [unwired: 7 in]
            n472 = call "Initialize update array.vi"("Camera label names"=w1171, "RBCIA (Rack based camera image indicator mapping) out"=w1172) -> ("Dynamic image update params.Image update"=w1170:cluster{"Rack Id":i32, "Update image":bool[]}[])  [unwired: 9 in]
            n473 = Merge Errors(w1146, w1150, w1151) -> (w1143:errorcluster)
            n474 = call <vilib>:"Add State(s) to Queue__JKI_lib_State_Machine.vi"("State(s) in Front (\"\")"=w1177, "State(s) in (\"\")"=w1181) -> ("States Out"=w1182:string)  [unwired: 13 in]
            n475 = Bundle By Name(cluster=T33 {"Label array"=[], "Image ref array"=[], "Rack 1 Tbl Refnum"=refnum, "Tab control"=refnum, "Rack 2 Tbl Refnum"=refnum, "String label"=[], "Diagnostics tab ref"=refnum, "Counts"=refnum} ("References"), "Diagnostics tab ref"=w1169, "Label array"=w1179, "Image ref array"=w1180, "Tab control"=w1178, "Counts"=w1164) -> (w1162:T33)
            n476 = property class="Str"(reference=w1145, error in=w1143, "DisabledEnum"=T28."Enabled" ("Disabled")) -> (error out=w1140:errorcluster)  [unwired: 1 out]
            n477 = Bundle By Name(cluster=w1161, "AdditionalFeatures.DynamicImageHandling.RBCIA"=w1172, "AdditionalFeatures.DynamicImageHandling.ISIM"=w1175, "AdditionalFeatures.DynamicImageHandling.Camera labels list"=w1173, "AdditionalFeatures.DynamicImageHandling.Image update"=w1170) -> (w1159:T38)
            n478 = call "Rearrange images (15..05).vi"("Selet tab"=enum16{"Diagnostics", "Main"}."Main", "Image indicator layouts 2"=w1176, "Camera names"=w1173, "Type of label"=w1168, "References"=w1162, "error in (no error)"=w1143) -> ("error out"=w1142:errorcluster)  [unwired: 9 in]
            n479 = Merge Errors(w1140, w1142) -> (w1141:errorcluster)
          }
          frame "ReadyToRun" {
            n480 = Unbundle By Name(w1198) -> ("AdditionalFeatures.DynamicImageHandling"=w1206:T59, "AdditionalFeatures.DynamicImageHandling.ISIM"=w1204:u8[], "Inspection.#Racks"=w1203:u8, "AdditionalFeatures.DynamicImageHandling.Enable DIH?"=w1201:bool)
            n481 = Unbundle By Name(w1198) -> ("AdditionalFeatures.PageHandling.Current state"=w1186:string, "Inspection.Inspection After Stop"=w1195:bool, "ControlsIndicators.Inspection.Label array"=w1197:refnum<vi>[])
            n482 = Concatenate Strings("\r", "DisplayImages") -> (w1188:string)
            n483 = Bundle By Name(cluster=cluster{"ISIM":u8[], "#Racks":i32} {"ISIM"=[], "#Racks"=0} ("Rack deatils"), "ISIM"=w1204, "#Racks"=w1203) -> (w1202:cluster{"ISIM":u8[], "#Racks":i32})
            n484 = Select(t=w1188, s=w1195, f="") -> (s? t:f=w1191:string)
            n485 = case shown="\"Master sample\", \"diagnostics\"" w1186 {
              tunnel: ["" "UI controls access>>[Inspection,Ready to run]\nPart selection>>Disable selection" ("State(s) in Front (\"\")")] -> w1187
              frame "Master sample", "diagnostics" {
              }
              frame "Inspection", Default {
              }
            }
            n486 = call "Set image label attributes.vi"("Enable dynamic stream change?"=w1201, "error in (no error)"=w1200, "Rack deatils"=w1202, "Dynamic image update params"=w1206, "Label array"=w1197) -> ("error out"=w1207:errorcluster)  [unwired: 6 in]
            n487 = call "Ready to run.vi"("error in (no error)"=w1200, "ZenGage v3.0 UI in"=w1198) -> ("error out"=w1212:errorcluster)  [unwired: 8 in, 1 out]
            n488 = Concatenate Strings(w1187, w1191) -> (w1192:string)
            n489 = Merge Errors(w1207, w1212) -> (w1211:errorcluster)
            n490 = Bundle By Name(cluster=w1198, "AdditionalFeatures.PageHandling.Previous control access state"="Inspection", "AdditionalFeatures.Popup.Restore main tab"="[Inspection,Ready to run]", "Inspection.Inspection After Stop"=FALSE, "Inspection.Reel complete"=FALSE) -> (w1196:T38)
            n491 = call <vilib>:"Add State(s) to Queue__JKI_lib_State_Machine.vi"("State(s) in Front (\"\")"=w1192, "State(s) in (\"\")"=w1209) -> ("States Out"=w1208:string)  [unwired: 13 in]
          }
          frame "Pause" {
            n492 = Unbundle By Name(w1217) -> ("SendClusterData"=w1216:refnum<user-event>)
            n493 = Unbundle By Name(w1219) -> ("AdditionalFeatures.PageHandling.Current state"=w1220:string)
            n494 = case shown="\"fail\"" w1223 {
              tunnel: [FALSE TRUE] -> w1222
              frame "pass", Default {
              }
              frame "fail" {
              }
            }
            n495 = case shown="\"inspection\", Default" w1220 {
              tunnel: w1226 -> [w1232 w1241]
              tunnel: w1225 -> [_ w1238]
              tunnel: [w1231 w1236] -> w1224
              tunnel: w1222 -> [_ w1240]
              tunnel: w1219 -> [w1229 w1239]
              tunnel: [w1229 w1234] -> w1218
              tunnel: w1216 -> [_ w1235]
              frame "diagnostics" {
                n496 = Unbundle By Name(w1229) -> ("ControlsIndicators.Diagnostics.PAUSE"=w1233:refnum<vi>)
                n497 = property class="ColBox"(reference=w1233, error in=w1232, "Value"=u32 8978365 ("Color Box")) -> (error out=w1231:errorcluster)  [unwired: 1 out]
              }
              frame "inspection", Default {
                n498 = call "Pause state.vi"("error in (no error)"=w1241, "fail?"=w1240, "Event Registration Refnum"=w1238, "ZenGage v3.0 UI in"=w1239) -> ("error out"=w1237:errorcluster, "ZenGage v3.0 UI in"=w1234:T38)  [unwired: 6 in]
                n499 = Generate User Event(user event=w1235, event data cluster=w1234, error in=w1237) -> (error out=w1236:errorcluster)  [unwired: 1 in, 1 out]
              }
            }
            n500 = call <vilib>:"Add State(s) to Queue__JKI_lib_State_Machine.vi"("State(s) in Front (\"\")"="Idle" ("State(s) in Front (\"\")"), "State(s) in (\"\")"=w1221) -> ("States Out"=w1228:string)  [unwired: 13 in]
          }
          frame "Stop" {
            w1258 = T60 {"Image update"=[], "RBCIA"=[], "ISIM"=[], "Camera labels list"=[], "Enable DIH?"=FALSE, "Init params"=TRUE}  # Dynamic image update params
            # "modified(11.12.2018)"
            n501 = Unbundle By Name(w1252) -> ("AdditionalFeatures.PageHandling.Current state"=w1254:string)
            n502 = case shown="\"inspection\", Default" w1254 {
              tunnel: [w1262 w1277] -> w1250
              tunnel: w1257 -> [_ w1268]
              tunnel: w1252 -> [w1262 w1274]
              tunnel: w1256 -> [w1266 w1273]
              tunnel: [w1265 w1270] -> w1255
              tunnel: w1251 -> [_ w1269]
              tunnel: ["Idle" ("State(s) in Front (\"\")") "UI controls access>>[Inspection,Stop]\nPart selection>>Enable selection\nPart selection>>Initialize\nInitialize images" ("State(s) in Front (\"\")")] -> w1247
              frame "diagnostics" {
                n503 = Unbundle By Name(w1262) -> ("ControlsIndicators.Diagnostics.STOP"=w1264:refnum<vi>)
                n504 = property class="ColBox"(reference=w1264, error in=w1266, "Value"=u32 8978365 ("Color Box")) -> (error out=w1265:errorcluster)  [unwired: 1 out]
              }
              frame "inspection", Default {
                n505 = Unbundle By Name(w1269) -> ("Enable shortkey"=w1276:refnum<user-event>)
                n506 = call "Stop state.vi"("error in (no error)"=w1273, "Event Registration Refnum"=w1268, "ZenGage v3.0 UI in"=w1274) -> ("error out"=w1272:errorcluster, "ZenGage v3.0 out"=w1277:T38)  [unwired: 7 in]
                n507 = Generate User Event(user event=w1276, event data cluster=FALSE ("event data"), error in=w1273) -> (error out=w1271:errorcluster)  [unwired: 1 in, 1 out]
                n508 = Merge Errors(w1272, w1271) -> (w1270:errorcluster)
              }
            }
            n509 = call <vilib>:"Add State(s) to Queue__JKI_lib_State_Machine.vi"("State(s) in Front (\"\")"=w1247, "State(s) in (\"\")"=w1259) -> ("States Out"=w1260:string)  [unwired: 13 in]
            n510 = Bundle By Name(cluster=w1250, "Inspection.#Racks"=u8 0, "AdditionalFeatures.DynamicImageHandling"=w1258, "Inspection.Inspection After Stop"=TRUE, "AdditionalFeatures.Fail Ignore Count Reversal.Production ignored count"=u64 0, "AdditionalFeatures.Fail Ignore Count Reversal.Reel ignored count"=u64 0) -> (w1249:T38)
          }
          frame "DisplayAnalytics" {
            n511 = Unbundle By Name(w1279) -> ("ControlsIndicators.Inspection.Analytics VI\nreference"=w1280:refnum<vi>, "ControlsIndicators.General.Inspection SubPanel_Inspection"=w1278:refnum<vi>)
            n512 = invoke class="SubPnl" method="Insert VI"(reference=w1278, error in=w1282, "VI Ref"=w1280) -> (error out=w1281:errorcluster)  [unwired: 1 in, 3 out]
            n513 = call <vilib>:"Add State(s) to Queue__JKI_lib_State_Machine.vi"("State(s) in Front (\"\")"="UI controls access>>[Inspection,Stop]" ("State(s) in Front (\"\")"), "State(s) in (\"\")"=w1284) -> ("States Out"=w1285:string)  [unwired: 13 in]
          }
          frame "---------- Settings ----------" {
            n514 = call <vilib>:"Add State(s) to Queue__JKI_lib_State_Machine.vi"("State(s) in (\"\")"=w1288) -> ("States Out"=w1289:string)  [unwired: 14 in]
          }
          frame "DisplaySettingsOptions" {
            n515 = in-place {
              in-place-border: w1296 -> [w1306]
              in-place-border: w1295 -> [w1305]
              in-place-border: [w1304] -> w1294
              in-place-border: [w1303] -> w1293
              in-place-border: w1290 -> [w1301]
              n516 = in-place-cluster #9(w1292) -> ("ControlsIndicators.Inspection.Settings_Inspection"=w1299:refnum<vi>, "Diagnostics.Selection Done?"=w1302:bool)  [unwired: 1 out]
              n517 = case shown="\"user exists\", Default" w1306 {
                tunnel: w1305 -> [w1307 w1315]
                tunnel: w1302 -> [_ w1320]
                tunnel: [w1307 w1311] -> w1304
                tunnel: ["Idle" ("State(s) in Front (\"\")") w1318] -> w1303
                tunnel: [_ w1317] -> w1300
                tunnel: w1301 -> [_ w1316]
                tunnel: w1299 -> [_ w1314]
                frame "user doesn't exist" {
                }
                frame "user exists", Default {
                  n518 = call "settings_options_general.vi"("error in (no error)"=w1315, "Selection Done?"=w1320) -> ("error IO"=w1309:errorcluster, "button pressed"=w1319:T66)  [unwired: 8 in]
                  n519 = case shown="\"diagnostics\"" w1319 {
                    tunnel: ["Idle" "UI controls access>>[Diagnostics,Enable all]\nDisplayDiagnosticsPage" "Reset tolerance settings page"] -> w1318
                    tunnel: [_ _ TRUE] -> w1317
                    tunnel: w1309 -> [w1321 w1325 w1328]
                    tunnel: [w1321 w1324 w1328] -> w1312
                    tunnel: w1316 -> [_ w1323 _]
                    frame "cancel", Default {
                    }
                    frame "diagnostics" {
                      n520 = call "Send ButtonPress_UI.vi"("error in (no error)"=w1325, "FunctionalityName"="StateChange>>diagnostics", "Message Enqueuer"=w1323) -> ("error out"=w1324:errorcluster)  [unwired: 7 in, 1 out]
                    }
                    frame "edit tolerance" {
                    }
                  }
                  n521 = property class="Bool (strict)"(reference=w1314, error in=w1309, "DisabledEnum"=T28."Enabled" ("Disabled")) -> (error out=w1310:errorcluster)  [unwired: 1 out]
                  n522 = Merge Errors(w1310, w1312) -> (w1311:errorcluster)
                }
              }
              n523 = in-place-cluster #9("EditToleranceSettings.IsETLSelected"=w1300, "ControlsIndicators.Inspection.Settings_Inspection"=w1299, "Diagnostics.Selection Done?"=w1302) -> (w1291:T38)
            }
            n524 = call <vilib>:"Add State(s) to Queue__JKI_lib_State_Machine.vi"("State(s) in Front (\"\")"=w1293, "State(s) in (\"\")"=w1297) -> ("States Out"=w1298:string)  [unwired: 13 in]
          }
          frame "Reset tolerance settings page" {
            # "Your code here.\n(You can make a copy of, or modify, this frame)"
            n525 = Unbundle By Name(w1334) -> ("Diagnostics.Selection Done?"=w1348:bool, "ControlsIndicators.Edit Tolerance Limits.Select a part"=w1339:refnum<vi>, "ControlsIndicators.General.SelectionCluster.PART NAME"=w1331:refnum<vi>)
            n526 = case shown="True" w1348 {
              tunnel: ["Idle" "Read Algo and RC override JSON"] -> w1344
              tunnel: [T28."Enabled" ("Disabled") T28."Disabled and Grayed Out" ("Disabled")] -> w1338
              tunnel: ["Select a part" w1355] -> w1335
              tunnel: w1331 -> [_ w1358]
              tunnel: w1337 -> [w1351 w1357]
              tunnel: [w1351 w1356] -> w1336
              frame False {
                # "JSON is not read until a part is \nselected"
              }
              frame True {
                # "Read JSON after a part is selected"
                n527 = property class="CmbBox"(reference=w1358, error in=w1357) -> (error out=w1356:errorcluster, "Value"=w1355:string)  [unwired: 1 out]
              }
            }
            n528 = call "Update tolerance settings table.vi"("error in (no error)"=w1337, "ZenGage v3.0 UI in"=w1334) -> ("error out"=w1342:errorcluster, "ZenGage v3.0 UI out"=w1333:T38)  [unwired: 8 in]
            n529 = Concatenate Strings("UI controls access>>[Edit tolerance limits,default]", "\r", w1344) -> (w1345:string)
            n530 = call <vilib>:"Add State(s) to Queue__JKI_lib_State_Machine.vi"("State(s) in Front (\"\")"=w1345, "State(s) in (\"\")"=w1349) -> ("States Out"=w1350:string)  [unwired: 13 in]
            n531 = property class="CmbBox"(reference=w1339, error in=w1337, "DisabledEnum"=w1338, "Value"=w1335) -> (error out=w1340:errorcluster)  [unwired: 1 out]
            n532 = Bundle By Name(cluster=w1333, "AdditionalFeatures.PageHandling.Previous control access state"="Edit tolerance limits") -> (w1332:T38)
            n533 = Merge Errors(w1336, w1340, w1342) -> (w1341:errorcluster)
          }
          frame "---------- Master sample validation ----------" {
            n534 = call <vilib>:"Add State(s) to Queue__JKI_lib_State_Machine.vi"("State(s) in (\"\")"=w1363) -> ("States Out"=w1364:string)  [unwired: 14 in]
          }
          frame "MoveToNextSample" {
            n535 = call <vilib>:"Add State(s) to Queue__JKI_lib_State_Machine.vi"("State(s) in Front (\"\")"="UI controls access>>[Master sample,Move to next sample]" ("State(s) in Front (\"\")"), "State(s) in (\"\")"=w1368) -> ("States Out"=w1369:string)  [unwired: 13 in]
          }
          frame "InitializeMasterSample" {
            n536 = in-place {
              in-place-border: w1372 -> [w1380]
              in-place-border: [w1384] -> w1371
              n537 = in-place-cluster #10(w1373) -> ("ControlsIndicators.General.Image Reference array"=w1379:refnum<vi>[], "ControlsIndicators.Inspection.Cards array"=w1383:refnum<vi>)
              n538 = for {
                tunnel: w1379 -> [w1387] mode=indexing
                tunnel: w1380 -> [w1388]
                tunnel: [w1385] -> _ mode=indexing
                # "Reinit images"
                n539 = property class="ImageControl"(reference=w1387, error in=w1388, "Value"=variant) -> (reference out=w1385:refnum<vi>)  [unwired: 1 out]
              }
              n540 = property class="Arr (strict)"(reference=w1383, error in=w1380, "Value"=T9 []) -> (reference out=w1381:refnum<vi>, error out=w1384:errorcluster)
              n541 = in-place-cluster #10("ControlsIndicators.General.Image Reference array"=w1379, "ControlsIndicators.Inspection.Cards array"=w1381) -> (w1370:T38)
            }
            n542 = call <vilib>:"Add State(s) to Queue__JKI_lib_State_Machine.vi"("State(s) in Front (\"\")"="UI controls access>>[Master sample,Initialize master sample]" ("State(s) in Front (\"\")"), "State(s) in (\"\")"=w1377) -> ("States Out"=w1378:string)  [unwired: 13 in]
            n543 = Bundle By Name(cluster=w1370, "AdditionalFeatures.PageHandling.Current state"="Master sample") -> (w1374:T38)
          }
          frame "MasterSampleValidationPass" {
            n544 = call <vilib>:"Add State(s) to Queue__JKI_lib_State_Machine.vi"("State(s) in Front (\"\")"="UI controls access>>[Master sample,Master sample validation pass]" ("State(s) in Front (\"\")"), "State(s) in (\"\")"=w1392) -> ("States Out"=w1393:string)  [unwired: 13 in]
          }
          frame "MasterSampleValidationFail" {
            n545 = call <vilib>:"Add State(s) to Queue__JKI_lib_State_Machine.vi"("State(s) in Front (\"\")"="UI controls access>>[Master sample,Master sample validation fail]" ("State(s) in Front (\"\")"), "State(s) in (\"\")"=w1397) -> ("States Out"=w1398:string)  [unwired: 13 in]
          }
          frame "Update master sample message" {
            n546 = Unbundle By Name(w1411) -> ("ControlsIndicators.General.Main Tab"=w1401:refnum<vi>, "AdditionalFeatures.Master sample validation.Master sample part message"=w1408:string, "AdditionalFeatures.Master sample validation.Master sample general message"=w1404:string, "ControlsIndicators.Master sample.Master sample part message"=w1409:refnum<vi>, "ControlsIndicators.Master sample.Master sample message"=w1410:refnum<vi>)
            n547 = Equal?(x=w1404, y="") -> (x = y?=w1402:bool)
            n548 = case shown="False" w1402 {
              tunnel: w1401 -> [w1417 _]
              tunnel: w1400 -> [w1416 w1418]
              tunnel: [w1415 w1418] -> w1399
              frame False {
                n549 = property class="TabCtl (strict)"(reference=w1417, error in=w1416, "Value"=T1."Run") -> (error out=w1415:errorcluster)  [unwired: 1 out]
              }
              frame True {
              }
            }
            n550 = property class="Str"(reference=w1409, error in=w1400, "Value"=w1408) -> (error out=w1406:errorcluster)  [unwired: 1 out]
            n551 = property class="Str"(reference=w1410, error in=w1400, "Value"=w1404) -> (error out=w1407:errorcluster)  [unwired: 1 out]
            n552 = Merge Errors(w1399, w1406, w1407) -> (w1405:errorcluster)
            n553 = call <vilib>:"Add State(s) to Queue__JKI_lib_State_Machine.vi"("State(s) in (\"\")"=w1412) -> ("States Out"=w1413:string)  [unwired: 14 in]
          }
          frame "---------- Software exit ----------" {
            n554 = call <vilib>:"Add State(s) to Queue__JKI_lib_State_Machine.vi"("State(s) in (\"\")"=w1421) -> ("States Out"=w1422:string)  [unwired: 14 in]
          }
          frame "SoftwareExit" {
            n555 = case shown="\"stop\"" w1435 {
              tunnel: [TRUE FALSE] -> w1431
              frame "stop" {
              }
              frame "continue", Default {
              }
            }
            n556 = Unbundle By Name(w1426) -> ("User Events Cluster_UI"=w1423:T37, "Stop slave user event_UI"=w1425:refnum<user-event>)
            n557 = Unbundle By Name(w1428) -> ("AdditionalFeatures.Core.Current VI Reference"=w1427:refnum<vi>)
            n558 = call "UI exit.vi"("ZenGage v3.0 UI in"=w1428, "SM_Stop_Stop_UI"=w1431, "Event Registration Refnum"=w1429, "User Events Cluster_UI"=w1423, "This VI"=w1427, "error in (no error)"=w1432, "SlaveLoop_UI"=w1425) -> ("ZenGage v3.0 UI out"=w1430:T38, "Stop Actor Loop"=w1434:bool, "error out"=w1424:errorcluster)  [unwired: 6 in]
            n559 = call <vilib>:"Add State(s) to Queue__JKI_lib_State_Machine.vi"("State(s) in Front (\"\")"="Idle" ("State(s) in Front (\"\")"), "State(s) in (\"\")"=w1433) -> ("States Out"=w1437:string)  [unwired: 13 in]
          }
        }
        n560 = Concatenate Strings(w174, "\r", w171) -> (w172:string)
        "Program flow" <- w172
        n561 = case shown="False" w168 {
          tunnel: w170 -> [w191 w193]
          tunnel: [w190 w193] -> w169
          tunnel: w167 -> [w189 _]
          tunnel: w166 -> [w188 w192]
          tunnel: [w188 w192] -> w165
          frame False {
            n562 = Generate User Event(user event=w189, event data cluster=w188, error in=w191) -> (error out=w190:errorcluster)  [unwired: 1 in, 1 out]
          }
          frame True {
          }
        }
      }
      n563 = while {
        tunnel: w160 -> [w1453]
        shift-right: [w1448] -> w161
        shift-left: w157 -> [w1450]
        tunnel: w159 -> [w1449]
        shift-right: [w1441] -> _
        shift-left: w149 -> [w1452]
        tunnel: w152 -> [w1447]
        tunnel: w150 -> [w1446]
        tunnel: w147 -> [w1442]
        stop <- w1451 stop-if-true
        # "User screen interaction loop"
        n564 = event shown="[22] \"Fail count reverse\": Value Change" {
          selector: w1446 -> [_ w1467 _ _ _ _ _ _ _ _ _ _ _ _ _ _ _ _ _ _ _ _ _]
          dyn-events: _ -> [_ _ _ _ _ _ _ _ _ _ _ _ _ _ _ _ _ _ _ _ _ _ _]
          timeout: -1 -> [_ _ _ _ _ _ _ _ _ _ _ _ _ _ _ _ _ _ _ _ _ _ _]
          tunnel: w1450 -> [w1460 w1473 w1490 w1501 w1514 w1548 w1565 w1600 w1622 w1631 w1647 w1651 w1667 w1672 w1683 w1697 w1724 w1729 w1744 w1748 w1757 w1762 w1774]
          tunnel: w1453 -> [_ w1472 w1485 _ w1512 _ w1567 w1601 w1619 _ _ w1649 _ _ _ _ _ _ _ _ _ _ w1778]
          tunnel: [w1460 w1463 w1489 w1497 w1511 w1547 w1558 w1602 w1621 w1630 w1644 w1653 w1661 w1671 w1682 w1694 w1723 w1728 w1744 w1745 w1757 w1759 w1769] -> w1445
          tunnel: w1452 -> [w1459 w1468 w1487 w1502 w1509 w1546 w1566 w1603 w1616 w1632 w1643 w1660 w1666 w1670 w1681 w1696 w1725 w1727 w1737 w1751 w1755 w1766 w1775]
          tunnel: [_ _ _ _ _ _ _ _ _ _ _ _ _ _ _ _ _ _ _ w1752 _ _ _] -> w1451
          tunnel: w1449 -> [_ w1466 w1488 w1496 _ _ w1557 _ w1618 w1623 _ _ _ _ _ w1693 _ _ _ _ _ _ w1767]
          tunnel: [w1459 w1464 w1487 w1502 w1509 w1545 w1560 w1603 w1614 w1632 w1643 w1660 w1663 w1669 w1680 w1695 w1725 w1727 w1736 w1751 w1754 w1766 w1772] -> w1441
          tunnel: w1447 -> [_ w1462 _ _ _ _ w1563 _ _ w1627 _ _ _ _ _ w1691 _ _ _ w1746 _ _ w1777]
          tunnel: [_ TRUE _ TRUE TRUE _ TRUE _ _ _ _ _ _ _ _ _ _ _ TRUE _ TRUE _ _] -> w1443
          event Timeout {
            n565 = event-data() -> ()  [unwired: 1 in, 3 out]
          }
          event "Run_Inspection", "Pause_Inspection", "logout_Diagnostics", "Logout_EditTolerance", "Stop_Inspection", "Settings_Inspection", "Update List", "Save", "Next", "Repeat": Value Change {
            n566 = event-data() -> ("CtlRef"=w1469:refnum<vi>, "NewVal"=w1465:bool)  [unwired: 1 in, 4 out]
            n567 = property on="UI Button Control" class="Bool (strict)"(reference=w1469, error in=w1473) -> (error out=w1470:errorcluster, "Label.Text"=w1471:string)  [unwired: 1 out]
            n568 = case shown="False" w1465 {
              tunnel: w1472 -> [w1479 _]
              tunnel: w1471 -> [w1478 _]
              tunnel: w1470 -> [w1482 w1484]
              tunnel: [w1476 w1484] -> w1463
              tunnel: w1468 -> [w1481 w1483]
              tunnel: [w1477 w1483] -> w1464
              tunnel: w1467 -> [_ _]
              tunnel: w1466 -> [w1480 _]
              tunnel: w1462 -> [w1475 _]
              frame False {
                # "Take this particular mechanical action of the switch for data updation"
                n569 = Unbundle By Name(w1475) -> ("SendClusterData to MainLoop"=w1474:refnum<user-event>)
                n570 = call "Process button press.vi"("DataCluster in"=w1481, "Label.Text"=w1478, "Send ClusterData"=w1474, "Self Enqueuer"=w1480, "error in (no error)"=w1482, "Caller Enqueuer"=w1479) -> ("DataCluster out"=w1477:T38, "error out"=w1476:errorcluster)  [unwired: 8 in]
              }
              frame True {
                # "Ignore this value change as it is not be read  for (switch until released)"
              }
            }
          }
          event "Analytics_Inspection": Value Change {
            n571 = event-data() -> ("NewVal"=w1486:bool)  [unwired: 1 in]
            n572 = call "Analytics update.vi"("error in (no error)"=w1490, "SM Enqueuer"=w1485, "User Interface enqueuer"=w1488, "analyticsButtonState"=w1486) -> ("error out"=w1489:errorcluster)  [unwired: 7 in]
          }
          event "change", "reset", "confirm", "ok": Value Change {
            n573 = event-data() -> ("CtlRef"=w1500:refnum<vi>)  [unwired: 1 in, 5 out]
            n574 = property class="Ctl"(reference=w1500, error in=w1501) -> (error out=w1498:errorcluster, "Label.Text"=w1499:string)  [unwired: 1 out]
            n575 = case shown="\"change\", Default" w1499 {
              tunnel: ["Change\nPart selection>>Enable selection" "Reset" "Confirm\nPart selection>>Disable selection" "Part Selection" "OK"] -> w1494
              frame "change", Default {
              }
              frame "reset" {
              }
              frame "confirm" {
              }
              frame "Part Name" {
              }
              frame "ok" {
              }
            }
            n576 = Concatenate Strings("Part selection>>", w1494) -> (w1492:string)
            n577 = call "Send ButtonPress_UI.vi"("Message Priority (Normal)"=Message_Priority."High", "error in (no error)"=w1498, "FunctionalityName"=w1492, "Message Enqueuer"=w1496) -> ("error out"=w1497:errorcluster)  [unwired: 6 in, 1 out]
          }
          event Key Down {
            n578 = event-data() -> ("ScanCode"=w1513:i16)  [unwired: 1 in]
            n579 = Unbundle By Name(w1509) -> ("AdditionalFeatures.SlaveLoopData.EnableShortKeyPress"=w1510:bool)
            n580 = case shown="True" w1510 {
              tunnel: w1514 -> [w1515 w1519]
              tunnel: w1513 -> [_ w1518]
              tunnel: w1512 -> [_ w1517]
              tunnel: [w1515 w1516] -> w1511
              frame False {
              }
              frame True {
                n581 = case shown="48, Default" w1518 {
                  tunnel: w1519 -> [w1527 w1533 w1539 w1544]
                  tunnel: [w1526 w1532 w1538 w1544] -> w1516
                  tunnel: w1517 -> [w1525 w1529 w1537 _]
                  frame 19 {
                    n582 = Bundle By Name(cluster=T25 {"Acknowledgement_SM"={"Enqueuer"=refnum, "VIReference"=refnum, "VIName"=""}, "Button name"="", "PartDetails"={"PartName"="", "ConnectorsInReel"=0, "TotalCounts"=0, "OperatorName"="", "StampingMachineID"=0}, "SensorName"="", "CameraName"="", "PopupFeedbackDetails"={"Pop-up Type"=enum."Open Logo Display", "Message"="", "Pressed Button"=""}, "EventResponse"="", "ErrorMessage"="", "FailCountIgnore"={"ReelIgnoreCount"=0, "ProductionIgnoreCount"=0}} ("OutputDetails"), "Button name"="Run") -> (w1522:T25)
                    n583 = call "Output_UI.vi"("OutputDetails"=w1522, "error in"=w1527, "Functionality"=Output_choice."ButtonPress", "Testbench"=TRUE, "SMEnqueuer"=w1525) -> ("error out"=w1526:errorcluster)  [unwired: 6 in]
                  }
                  frame 25 {
                    n584 = Bundle By Name(cluster=T25 {"Acknowledgement_SM"={"Enqueuer"=refnum, "VIReference"=refnum, "VIName"=""}, "Button name"="", "PartDetails"={"PartName"="", "ConnectorsInReel"=0, "TotalCounts"=0, "OperatorName"="", "StampingMachineID"=0}, "SensorName"="", "CameraName"="", "PopupFeedbackDetails"={"Pop-up Type"=enum."Open Logo Display", "Message"="", "Pressed Button"=""}, "EventResponse"="", "ErrorMessage"="", "FailCountIgnore"={"ReelIgnoreCount"=0, "ProductionIgnoreCount"=0}} ("OutputDetails"), "Button name"="Pause") -> (w1535:T25)
                    n585 = call "Output_UI.vi"("OutputDetails"=w1535, "error in"=w1533, "Functionality"=Output_choice."ButtonPress", "Testbench"=TRUE, "SMEnqueuer"=w1529) -> ("error out"=w1532:errorcluster)  [unwired: 6 in]
                  }
                  frame 31 {
                    n586 = Bundle By Name(cluster=T25 {"Acknowledgement_SM"={"Enqueuer"=refnum, "VIReference"=refnum, "VIName"=""}, "Button name"="", "PartDetails"={"PartName"="", "ConnectorsInReel"=0, "TotalCounts"=0, "OperatorName"="", "StampingMachineID"=0}, "SensorName"="", "CameraName"="", "PopupFeedbackDetails"={"Pop-up Type"=enum."Open Logo Display", "Message"="", "Pressed Button"=""}, "EventResponse"="", "ErrorMessage"="", "FailCountIgnore"={"ReelIgnoreCount"=0, "ProductionIgnoreCount"=0}} ("OutputDetails"), "Button name"="Stop") -> (w1543:T25)
                    n587 = call "Output_UI.vi"("OutputDetails"=w1543, "error in"=w1539, "Functionality"=Output_choice."ButtonPress", "Testbench"=TRUE, "SMEnqueuer"=w1537) -> ("error out"=w1538:errorcluster)  [unwired: 6 in]
                  }
                  frame 48, Default {
                  }
                }
              }
            }
          }
          event "Event  Reason  List": Value Change {
            n588 = event-data() -> ("NewVal"=w1549:string)  [unwired: 1 in]
            n589 = in-place {
              in-place-border: w1549 -> [w1551]
              in-place-border: w1548 -> [w1554]
              in-place-border: [w1553] -> w1547
              n590 = in-place-cluster #11(w1546) -> ("ControlsIndicators.General.confirm_eventReason"=w1552:refnum<vi>)  [unwired: 1 out]
              n591 = property class="Bool (strict)"(reference=w1552, error in=w1554, "DisabledEnum"=T28."Enabled" ("Disabled")) -> (error out=w1553:errorcluster)  [unwired: 1 out]
              n592 = in-place-cluster #11("AdditionalFeatures.Chosen event reason"=w1551, "ControlsIndicators.General.confirm_eventReason"=w1552) -> (w1545:T38)
            }
          }
          event "confirm_eventReason": Value Change {
            n593 = event-data() -> ("CtlRef"=w1564:refnum<vi>)  [unwired: 1 in]
            n594 = in-place {
              in-place-border: w1567 -> [w1584]
              in-place-border: w1565 -> [w1582]
              in-place-border: [w1572] -> w1561
              in-place-border: w1564 -> [w1580]
              in-place-border: w1557 -> [_]
              # "code modified (16-09-2018)\nchange sequence"
              n595 = in-place-cluster #12(w1566) -> ("JSONRead.ConfigurationCluster.UIParameters.EventReasonsList.Ignored"=w1573:string[], "AdditionalFeatures.Fail Ignore Count Reversal.Production ignored count"=w1578:u64, "AdditionalFeatures.Fail Ignore Count Reversal.Reel ignored count"=w1575:u64, "AdditionalFeatures.Chosen event reason"=w1568:string, "ControlsIndicators.General.Event reason switching tab"=w1583:refnum<vi>)
              n596 = Bundle By Name(cluster=T25 {"Acknowledgement_SM"={"Enqueuer"=refnum, "VIReference"=refnum, "VIName"=""}, "Button name"="", "PartDetails"={"PartName"="", "ConnectorsInReel"=0, "TotalCounts"=0, "OperatorName"="", "StampingMachineID"=0}, "SensorName"="", "CameraName"="", "PopupFeedbackDetails"={"Pop-up Type"=enum."Open Logo Display", "Message"="", "Pressed Button"=""}, "EventResponse"="", "ErrorMessage"="", "FailCountIgnore"={"ReelIgnoreCount"=0, "ProductionIgnoreCount"=0}} ("OutputDetails"), "EventResponse"=w1568) -> (w1585:T25)
              n597 = Search 1D Array(1D array=w1573, element=w1568) -> (index of element=w1569:i32)  [unwired: 1 in]
              n598 = property class="TabCtl (strict)"(reference=w1583, error in=w1582, "Value"=enum32{"EventReason", "InspectionButtons"}."InspectionButtons") -> (error out=w1588:errorcluster)  [unwired: 1 out]
              n599 = property class="Bool (strict)"(reference=w1580, error in=w1582, "DisabledEnum"=T28."Disabled and Grayed Out" ("Disabled")) -> (error out=w1579:errorcluster)  [unwired: 1 out]
              n600 = Not Equal?(x=w1569, y=-1) -> (x != y?=w1576:bool)
              n601 = call "Output_UI.vi"("OutputDetails"=w1585, "error in"=w1582, "Functionality"=Output_choice."SendEventReasonResponse", "SMEnqueuer"=w1584) -> ("error out"=w1587:errorcluster)  [unwired: 7 in]
              n602 = case shown="False" w1576 {
                tunnel: w1578 -> [w1591 w1594]
                tunnel: [w1591 w1595] -> w1577
                tunnel: w1575 -> [w1590 w1593]
                tunnel: [w1590 w1592] -> w1574
                frame False {
                  # "Not ignored"
                }
                frame True {
                  # "Ignored"
                  n603 = Increment(x=w1594) -> (x+1=w1595:u64)
                  n604 = Increment(x=w1593) -> (x+1=w1592:u64)
                }
              }
              n605 = Merge Errors(w1587, w1588, w1579) -> (w1572:errorcluster)
              n606 = in-place-cluster #12("JSONRead.ConfigurationCluster.UIParameters.EventReasonsList.Ignored"=w1573, "AdditionalFeatures.Fail Ignore Count Reversal.Production ignored count"=w1577, "AdditionalFeatures.Fail Ignore Count Reversal.Reel ignored count"=w1574, "AdditionalFeatures.Chosen event reason"=w1568, "ControlsIndicators.General.Event reason switching tab"=w1583) -> (w1560:T38)
            }
            n607 = Unbundle By Name(w1563) -> ("SendClusterData to MainLoop"=w1562:refnum<user-event>)
            n608 = Generate User Event(user event=w1562, event data cluster=w1560, error in=w1561) -> (error out=w1559:errorcluster)  [unwired: 1 in, 1 out]
            n609 = call "Send ButtonPress_UI.vi"("error in (no error)"=w1559, "FunctionalityName"="UpdateFailIgnoreCounts", "Message Enqueuer"=w1557) -> ("error out"=w1558:errorcluster)  [unwired: 7 in, 1 out]
          }
          event "SoftwareExit": Value Change {
            n610 = event-data() -> ("CtlRef"=w1598:refnum<vi>, "NewVal"=w1596:bool)  [unwired: 1 in, 4 out]
            n611 = property on="UI Button Control" class="Bool (strict)"(reference=w1598, error in=w1600) -> (error out=w1599:errorcluster, "Label.Text"=w1597:string)  [unwired: 1 out]
            n612 = case shown="True" w1596 {
              tunnel: [w1604 w1608] -> w1602
              tunnel: w1601 -> [_ w1607]
              tunnel: w1599 -> [w1604 w1609]
              tunnel: w1597 -> [_ w1606]
              frame False {
              }
              frame True {
                n613 = Bundle By Name(cluster=T25 {"Acknowledgement_SM"={"Enqueuer"=refnum, "VIReference"=refnum, "VIName"=""}, "Button name"="", "PartDetails"={"PartName"="", "ConnectorsInReel"=0, "TotalCounts"=0, "OperatorName"="", "StampingMachineID"=0}, "SensorName"="", "CameraName"="", "PopupFeedbackDetails"={"Pop-up Type"=enum."Open Logo Display", "Message"="", "Pressed Button"=""}, "EventResponse"="", "ErrorMessage"="", "FailCountIgnore"={"ReelIgnoreCount"=0, "ProductionIgnoreCount"=0}} ("OutputDetails"), "Button name"=w1606) -> (w1612:T25)
                n614 = call "Output_UI.vi"("OutputDetails"=w1612, "error in"=w1609, "Functionality"=Output_choice."ButtonPress", "Testbench"=TRUE, "SMEnqueuer"=w1607) -> ("error out"=w1608:errorcluster)  [unwired: 6 in]
              }
            }
          }
          event Value Change {
            n615 = event-data() -> ("NewVal"=w1620:T6)  [unwired: 1 in]
            n616 = control-ref of="SensorDiagnosticsImage"() -> (w1613:refnum<vi>)
            n617 = call "Select a diagnostics.vi"("SensorImageRefnum"=w1613, "Selected label"=w1620, "error in (no error)"=w1622, "User interface Enqueuer"=w1618, "Caller Enqueuer"=w1619, "ZenGage v3.0 UI in"=w1616) -> ("error out"=w1621:errorcluster, "Diagnostic name"=w1617:string, "ZenGage v3.0 UI in"=w1615:T38)  [unwired: 3 in]
            n618 = Bundle By Name(cluster=w1615, "Diagnostics.SelectedDiagnostics"=w1617) -> (w1614:T38)
          }
          event Value Change {
            n619 = event-data() -> ()  [unwired: 1 in, 6 out]
            n620 = in-place {
              in-place-border: w1631 -> [w1641]
              in-place-border: [w1638] -> w1629
              n621 = in-place-cluster #13(w1632) -> ("ControlsIndicators.Edit Tolerance Limits.Back_Edit Tolerance"=w1635:refnum<vi>, "ControlsIndicators.Edit Tolerance Limits.ETL help string"=w1634:refnum<vi>)  [unwired: 1 out]
              n622 = property class="Bool (strict)"(reference=w1635, error in=w1641, "DisabledEnum"=T28."Enabled" ("Disabled")) -> (error out=w1639:errorcluster)  [unwired: 1 out]
              n623 = property class="Str"(reference=w1634, error in=w1641, "Value"="Please select a measurement checkbox to make the required changes for that particular measurement") -> (error out=w1640:errorcluster)  [unwired: 1 out]
              n624 = Merge Errors(w1639, w1640) -> (w1638:errorcluster)
              n625 = in-place-cluster #13("ControlsIndicators.Edit Tolerance Limits.Back_Edit Tolerance"=w1635, "ControlsIndicators.Edit Tolerance Limits.ETL help string"=w1634, "EditToleranceSettings.IsETLSelected"=TRUE) -> (w1625:T38)
            }
            n626 = Unbundle By Name(w1627) -> ("SendClusterData to MainLoop"=w1626:refnum<user-event>)
            n627 = Generate User Event(user event=w1626, event data cluster=w1625, error in=w1629) -> (error out=w1628:errorcluster)  [unwired: 1 in, 1 out]
            n628 = call "Send ButtonPress_UI.vi"("error in (no error)"=w1628, "FunctionalityName"="Read Algo and RC override JSON\nRead ET parameters" ("State(s) in Front (\"\")"), "Message Enqueuer"=w1623) -> ("error out"=w1630:errorcluster)  [unwired: 7 in, 1 out]
          }
          event "Measurement\nEnable": Value Change {
            n629 = event-data() -> ("NewVal"=w1646:bool)  [unwired: 1 in, 5 out]
            n630 = Unbundle By Name(w1643) -> ("EditToleranceSettings.Input ListBox.Current Active Position"=w1645:T46, "ControlsIndicators.Edit Tolerance Limits.Tolerance Limits Listbox"=w1642:refnum<vi>)
            n631 = call "Update eneble-disable measurement.vi"("error in (no error)"=w1647, "MeasurementListBox"=w1642, "Current Position on Listbox"=w1645, "Enabled?"=w1646) -> ("error out"=w1644:errorcluster)  [unwired: 7 in]
          }
          event Value Change {
            n632 = event-data() -> ("NewVal"=w1656:T6)  [unwired: 1 in]
            n633 = Unbundle By Name(w1660) -> ("ControlsIndicators.Diagnostics.Diagnostics Status"=w1658:refnum<vi>, "JSONRead.ConfigurationCluster"=w1659:T40, "Diagnostics.SelectedDiagnostics"=w1648:string)
            n634 = Concatenate Strings(w1656, "\r", "Status") -> (w1654:string)
            n635 = property class="Str"(reference=w1658, error in=w1651, "Value"=w1654) -> (error out=w1652:errorcluster)  [unwired: 1 out]
            n636 = call "Get name from label (Sub-diagnostics).vi"("SMEnqueuer"=w1649, "error in"=w1651, "Current diagnostics"=w1648, "Selected label"=w1656, "UI JSON read cluster"=w1659) -> ("error out"=w1650:errorcluster)  [unwired: 5 in, 1 out]
            n637 = Merge Errors(w1652, w1650) -> (w1653:errorcluster)
          }
          event "Tolerance Limits Listbox": Mouse Down {
            n638 = event-data() -> ("Coords"=w1665:T46)  [unwired: 1 in, 7 out]
            n639 = call "Measurement selected.vi"("error in (no error)"=w1667, "Coords"=w1665, "ZenGage v3.0 UI in"=w1666) -> ("error out"=w1662:errorcluster, "ZenGage v3.0 UI in"=w1664:T38)  [unwired: 7 in]
            n640 = Bundle By Name(cluster=w1664, "AdditionalFeatures.SlaveLoopData.Point32"=w1665) -> (w1663:T38)
            n641 = call <vilib>:"Clear Errors.vi"("error in (no error)"=w1662) -> ("error out"=w1661:errorcluster)  [unwired: 5 in, 1 out]
          }
          event "Cluster of limits": Value Change {
            n642 = event-data() -> ("CtlRef"=w1668:refnum<vi>)  [unwired: 1 in]
            n643 = in-place {
              in-place-border: w1672 -> [w1678]
              in-place-border: [w1677] -> w1671
              in-place-border: w1668 -> [w1674]
              n644 = in-place-cluster #14(w1670) -> ("ControlsIndicators"=w1673:T12, "EditToleranceSettings.Input ListBox"=w1675:T44)
              n645 = call "Cluster of Limits_UI.vi"("ControlsIndicators"=w1673, "error in (no error)"=w1678, "Cluster of limits"=w1674, "Input ListBox Cluster"=w1675) -> ("error out"=w1677:errorcluster, "ListBox Cluster out"=w1676:T44)  [unwired: 6 in]
              n646 = in-place-cluster #14("ControlsIndicators"=w1673, "EditToleranceSettings.Input ListBox"=w1676) -> (w1669:T38)
            }
          }
          event "Threshold limits": Value Change {
            n647 = event-data() -> ("CtlRef"=w1679:refnum<vi>)  [unwired: 1 in]
            n648 = in-place {
              in-place-border: w1683 -> [w1689]
              in-place-border: [w1686] -> w1682
              in-place-border: w1679 -> [w1684]
              n649 = in-place-cluster #15(w1681) -> ("EditToleranceSettings.Input ListBox"=w1688:T44, "ControlsIndicators"=w1685:T12)
              n650 = call "Cluster of M and N_UI.vi"("ControlsIndicators"=w1685, "error in (no error)"=w1689, "Threshold limits"=w1684, "Input ListBox Cluster"=w1688) -> ("error out"=w1686:errorcluster, "ListBox Cluster out"=w1687:T44)  [unwired: 6 in]
              n651 = in-place-cluster #15("EditToleranceSettings.Input ListBox"=w1687, "ControlsIndicators"=w1685) -> (w1680:T38)
            }
          }
          event "Restore to defaults_Edit Tolerance": Value Change {
            n652 = event-data() -> ("NewVal"=w1692:bool)  [unwired: 1 in, 5 out]
            n653 = Unbundle By Name(w1691) -> ("SendClusterData"=w1690:refnum<user-event>)
            n654 = case shown="True" w1692 {
              tunnel: w1697 -> [w1698 w1716]
              tunnel: w1696 -> [w1699 w1714]
              tunnel: [w1699 w1711] -> w1695
              tunnel: [w1698 w1710] -> w1694
              tunnel: w1693 -> [_ w1700]
              tunnel: w1690 -> [_ w1713]
              frame False {
              }
              frame True {
                w1709 = T47 {"Pop-up Type"=enum."Open Logo Display", "Title"="", "Message"="", "Button 1 Text"="", "Button 2 Text"="", "Show Close? T/F"=FALSE, "Title Blink? T/F"=FALSE, "Title Blink Colour"=0} ("PopupDetails")
                n655 = Bundle By Name(cluster=w1709, "Pop-up Type"=T35."Open Loading Bar", "Message"="Loading...Please Wait..." ("Loading string?")) -> (w1707:T47)
                n656 = call "Send DisplayPopup_UI.vi"("error in (no error)"=w1716, "PopupDetails"=w1707, "Message Enqueuer"=w1700) -> ("error out"=w1715:errorcluster)  [unwired: 7 in, 1 out]
                n657 = call "Restore to default.vi"("error in (no error)"=w1715, "User interface enqueuer"=w1700, "UIDataCluster"=w1714) -> ("error out"=w1704:errorcluster, "UIDataCluster out"=w1711:T38)  [unwired: 7 in]
                n658 = Bundle By Name(cluster=w1709, "Pop-up Type"=T35."Close Loading Bar") -> (w1701:T47)
                n659 = Generate User Event(priority (normal)=usereventprio."high priority", user event=w1713, event data cluster=w1711, error in=w1704) -> (error out=w1703:errorcluster)  [unwired: 1 out]
                n660 = call "Send DisplayPopup_UI.vi"("error in (no error)"=w1703, "PopupDetails"=w1701, "Message Enqueuer"=w1700) -> ("error out"=w1702:errorcluster)  [unwired: 7 in, 1 out]
                n661 = call "Send ButtonPress_UI.vi"("error in (no error)"=w1702, "FunctionalityName"="Read ET parameters", "Message Enqueuer"=w1700) -> ("error out"=w1710:errorcluster)  [unwired: 7 in, 1 out]
              }
            }
          }
          event "Door Poka \nYoke": Value Change {
            n662 = event-data() -> ("NewVal"=w1718:bool)  [unwired: 1 in, 5 out]
            n663 = Not(x=w1718) -> (.not. x?=w1719:bool)
            n664 = call <vilib>:"Application Directory.vi"() -> ("Application Directory"=w1722:path)
            n665 = Build Path(base path=w1722, name or relative path="Configuration file\\Zengage System JSON Override.json") -> (appended path=w1720:path)
            n666 = call "Door Poka Yoke_UI.vi"("error in (no error)"=w1724, "Door Poka Yoke"=w1719, "JSON FilePath"=w1720) -> ("error out"=w1723:errorcluster)  [unwired: 8 in]
          }
          event "Factory reset": Value Change {
            n667 = event-data() -> ("NewVal"=w1726:bool)  [unwired: 1 in, 5 out]
            n668 = case shown="True" w1726 {
              tunnel: w1729 -> [w1730 w1734]
              tunnel: [w1730 w1733] -> w1728
              tunnel: w1727 -> [_ w1732]
              frame False {
              }
              frame True {
                n669 = Unbundle By Name(w1732) -> ("JSONRead"=w1731:T39)
                n670 = call "Factory reset.vi"("error in (no error)"=w1734, "JSONRead in"=w1731) -> ("error out"=w1733:errorcluster)  [unwired: 9 in]
              }
            }
          }
          event User Event {
            n671 = event-data() -> ("JSONRead"=w1743:T39, "Inspection"=w1742:T41, "Diagnostics"=w1741:T42, "EditToleranceSettings"=w1740:T43, "ControlsIndicators"=w1739:T12, "AdditionalFeatures"=w1738:T58)  [unwired: 1 in]
            n672 = Bundle By Name(cluster=w1737, "JSONRead"=w1743, "Inspection"=w1742, "Diagnostics"=w1741, "EditToleranceSettings"=w1740, "ControlsIndicators"=w1739, "AdditionalFeatures"=w1738) -> (w1736:T38)
          }
          event User Event {
            n673 = event-data() -> ("Stop UI?"=w1752:bool)  [unwired: 1 in]
            n674 = Unbundle By Name(w1746) -> ("ButtonPress_UI"=w1750:refnum<user-event>)
            n675 = Generate User Event(priority (normal)=usereventprio."high priority", user event=w1750, event data cluster="SoftwareExit>>stop" ("Functionality name"), error in=w1748) -> (error out=w1745:errorcluster)  [unwired: 1 out]
          }
          event User Event {
            n676 = event-data() -> ("Enable shortkey"=w1756:bool)  [unwired: 1 in]
            n677 = Bundle By Name(cluster=w1755, "AdditionalFeatures.SlaveLoopData.EnableShortKeyPress"=w1756) -> (w1754:T38)
          }
          event "Hide": Value Change {
            n678 = event-data() -> ("NewVal"=w1763:bool)  [unwired: 1 in]
            n679 = Unbundle By Name(w1766) -> ("ControlsIndicators.Inspection.Counts array"=w1765:refnum<vi>[])
            n680 = Index Array(array=w1765) -> (element #1=w1764:refnum<vi>, element #2=w1758:refnum<vi>)  [unwired: 2 in]
            n681 = call "Test animation.vi"("error in (no error)"=w1762, "Hide?"=w1763, "Counts cluster"=w1764) -> ("error out"=w1761:errorcluster)  [unwired: 8 in]
            n682 = call "Test animation.vi"("error in (no error)"=w1762, "Hide?"=w1763, "Counts cluster"=w1758) -> ("error out"=w1760:errorcluster)  [unwired: 8 in]
            n683 = Merge Errors(w1761, w1760) -> (w1759:errorcluster)
          }
          event "Fail count reverse": Value Change {
            n684 = event-data() -> ("NewVal"=w1771:bool, "CtlRef"=w1782:refnum<vi>)  [unwired: 1 in]
            n685 = property class="Bool (strict)"(reference=w1782, error in=w1774, "BoolText.Text"="REVERSED" ("Boolean Text.Text"), "DisabledEnum"=T28."Disabled and Grayed Out" ("Disabled")) -> (error out=w1779:errorcluster)  [unwired: 1 out]
            n686 = case shown="True" w1771 {
              tunnel: w1779 -> [w1783 w1789]
              tunnel: w1778 -> [_ w1788]
              tunnel: w1775 -> [w1784 w1787]
              tunnel: [w1783 w1786] -> w1773
              tunnel: [w1784 w1785] -> w1772
              frame False {
              }
              frame True {
                n687 = in-place {
                  in-place-border: w1789 -> [w1799]
                  in-place-border: [w1798] -> w1786
                  in-place-border: w1788 -> [w1797]
                  n688 = in-place-cluster #16(w1787) -> ("AdditionalFeatures.Fail Ignore Count Reversal.Production ignored count"=w1792:u64, "AdditionalFeatures.Fail Ignore Count Reversal.Reel ignored count"=w1793:u64)
                  n689 = Bundle By Name(cluster=T25 {"Acknowledgement_SM"={"Enqueuer"=refnum, "VIReference"=refnum, "VIName"=""}, "Button name"="", "PartDetails"={"PartName"="", "ConnectorsInReel"=0, "TotalCounts"=0, "OperatorName"="", "StampingMachineID"=0}, "SensorName"="", "CameraName"="", "PopupFeedbackDetails"={"Pop-up Type"=enum."Open Logo Display", "Message"="", "Pressed Button"=""}, "EventResponse"="", "ErrorMessage"="", "FailCountIgnore"={"ReelIgnoreCount"=0, "ProductionIgnoreCount"=0}} ("OutputDetails"), "FailCountIgnore.ProductionIgnoreCount"=w1792, "FailCountIgnore.ReelIgnoreCount"=w1793) -> (w1794:T25)
                  n690 = in-place-cluster #16("AdditionalFeatures.Fail Ignore Count Reversal.Production ignored count"=u64 0 ("AdditionalFeatures.Master sample validation.Production ignored count"), "AdditionalFeatures.Fail Ignore Count Reversal.Reel ignored count"=u64 0 ("AdditionalFeatures.Master sample validation.Reel ignored count")) -> (w1785:T38)
                  n691 = call "Output_UI.vi"("OutputDetails"=w1794, "error in"=w1799, "Functionality"=Output_choice."SendIgnoredFailCount", "SMEnqueuer"=w1797) -> ("error out"=w1798:errorcluster)  [unwired: 7 in]
                }
              }
            }
            n692 = Unbundle By Name(w1777) -> ("SendClusterData to MainLoop"=w1776:refnum<user-event>)
            n693 = Generate User Event(user event=w1776, event data cluster=w1772, error in=w1773) -> (error out=w1770:errorcluster)  [unwired: 1 in, 1 out]
            n694 = call "Send ButtonPress_UI.vi"("error in (no error)"=w1770, "FunctionalityName"="UpdateFailIgnoreCounts", "Message Enqueuer"=w1767) -> ("error out"=w1769:errorcluster)  [unwired: 7 in, 1 out]
          }
        }
        n695 = case shown="False" w1443 {
          tunnel: w1445 -> [w1457 w1458]
          tunnel: [w1456 w1458] -> w1444
          tunnel: w1442 -> [w1455 _]
          tunnel: w1441 -> [w1454 _]
          frame False {
            # "Send data to main cluster"
            n696 = Generate User Event(user event=w1455, event data cluster=w1454, error in=w1457) -> (error out=w1456:errorcluster)  [unwired: 1 in, 1 out]
          }
          frame True {
          }
        }
        n697 = call <vilib>:"Clear Errors.vi"("error in (no error)"=w1444) -> ("error out"=w1448:errorcluster)  [unwired: 5 in, 1 out]
      }
      n698 = Merge Errors(w164, w161) -> (w158:errorcluster)
    }
  }
  n699 = control-ref of="InspectionSubTab"() -> ()  [unwired: 1 out]
  n700 = call-parent "Actor Core.vi"("error in"="error in", "Actor in"="ZenGage v3.0 UI in") -> ("error out"=w7:errorcluster, "Actor out"=→"Actor out":refnum<class "Actor.lvclass">)  [unwired: 8 in]
  n701 = Merge Errors(w7, w9) -> (→"error out":errorcluster)
